vi "Main_Practice.vi"() -> ()   [LabVIEW 2015]
panel:
  in  "Snap Number Counting":dbl=12.0
  out "Movie Point cluster":cluster{"Movie Y":dbl[], "Movie X":dbl[]}={"Movie Y"=[-12.0, -12.0, -12.0, -12.0, -12.0, -12.0, -2.92, -2.92, -2.92, -2.92, -2.92, -2.92], "Movie X"=[-1.0, -1.0, -1.0, -1.0, -1.0, -1.0, 1.02, 1.02, 1.02, 1.02, 1.02, 1.02]}
  out "Movie Point  Y Array":dbl[](array[numeric])=[-12.0, -12.0, -12.0, -12.0, -12.0, -12.0, -2.92, -2.92, -2.92, -2.92, -2.92, -2.92]
  out "Movie Point  X Array":dbl[](array[numeric])=[-1.0, -1.0, -1.0, -1.0, -1.0, -1.0, 1.02, 1.02, 1.02, 1.02, 1.02, 1.02]
  out "Snap Point cluster":cluster{"Snap Y":dbl[], "Snap X":dbl[]}
  out "Snap Point  Y Array":dbl[](array[numeric])
  out "Snap Point  X Array":dbl[](array[numeric])
  out "Stage XY Cluster":cluster{"Stage Y ":dbl[], "Stage X":dbl[]}
  in  "Previous Light control":T1={"Filter Set"=0, "Lasers DO"=[FALSE, FALSE, FALSE, FALSE, FALSE, FALSE], "Lasers AO (V)"=[0.0, 0.0, 0.0, 0.0, 0.0, 0.0], "LED"=FALSE, "Global"=FALSE} {"Lasers AO (V)" min=0.0 max=5.0 step=0.01 scale=0.0..5.0 scale format="%#1.2f"; "Filter Set" items=["R-QuasAr", "R-Cy5", "R-mCherry", "R-mOrange", "R-GFP", "R-CFP/DAPI", "R-BFP", "R-LED", "SDC-Cy5", "SDC-mCherry", "SDC-mO2", "SDC-GFP", "SDC-CFP/DAPI", "SDC-BFP", "SDC-LED"]}
  out "Image Info":T2={"Status"="Ready", "scale bar (μm)"=65.0, "Image"=array512x512[262144 elements], "Histogram"={"max value"=1766, "mean"=1643, "min value"=1545, "Histogram"={"X Values"=[1546.105, 1548.315, 1550.525, 1552.7350000000001, 1554.9450000000002, 1557.1550000000002, 1559.3650000000002, 1561.5750000000003, 1563.7850000000003, 1565.9950000000003, 1568.2050000000004, 1570.4150000000004, 1572.6250000000005, 1574.8350000000005, 1577.0450000000005, 1579.2550000000006, 1581.4650000000006, 1583.6750000000006, 1585.8850000000007, 1588.0950000000007, 1590.3050000000007, 1592.5150000000008, 1594.7250000000008, 1596.9350000000009, 1599.145000000001, 1601.355000000001, 1603.565000000001, 1605.775000000001, 1607.985000000001, 1610.195000000001, 1612.405000000001, 1614.6150000000011, 1616.8250000000012, 1619.0350000000012, 1621.2450000000013, 1623.4550000000013, 1625.6650000000013, 1627.8750000000014, 1630.0850000000014, 1632.2950000000014, 1634.5050000000015, 1636.7150000000015, 1638.9250000000015, 1641.1350000000016, 1643.3450000000016, 1645.5550000000017, 1647.7650000000017, 1649.9750000000017, 1652.1850000000018, 1654.3950000000018, 1656.6050000000018, 1658.8150000000019, 1661.025000000002, 1663.235000000002, 1665.445000000002, 1667.655000000002, 1669.865000000002, 1672.075000000002, 1674.2850000000021, 1676.4950000000022, 1678.7050000000022, 1680.9150000000022, 1683.1250000000023, 1685.3350000000023, 1687.5450000000023, 1689.7550000000024, 1691.9650000000024, 1694.1750000000025, 1696.3850000000025, 1698.5950000000025, 1700.8050000000026, 1703.0150000000026, 1705.2250000000026, 1707.4350000000027, 1709.6450000000027, 1711.8550000000027, 1714.0650000000028, 1716.2750000000028, 1718.4850000000029, 1720.695000000003, 1722.905000000003, 1725.115000000003, 1727.325000000003, 1729.535000000003, 1731.745000000003, 1733.955000000003, 1736.1650000000031, 1738.3750000000032, 1740.5850000000032, 1742.7950000000033, 1745.0050000000033, 1747.2150000000033, 1749.4250000000034, 1751.6350000000034, 1753.8450000000034, 1756.0550000000035, 1758.2650000000035, 1760.4750000000035, 1762.6850000000036, 1764.8950000000036], "Histogram: h(x)"=[1, 1, 0, 1, 1, 4, 2, 5, 3, 18, 22, 16, 26, 37, 83, 73, 96, 128, 153, 340, 297, 408, 511, 1003, 839, 1047, 1268, 1532, 2908, 2476, 2946, 3424, 3916, 7140, 5665, 6592, 6956, 7907, 13141, 9628, 10167, 10808, 16785, 11493, 11379, 11298, 11102, 15845, 9865, 9151, 8683, 7999, 10287, 6013, 5256, 4358, 3885, 4618, 2525, 2027, 1707, 1987, 906, 827, 574, 438, 582, 244, 189, 143, 113, 100, 44, 30, 24, 22, 15, 12, 12, 2, 0, 3, 2, 4, 2, 1, 1, 0, 0, 1, 0, 0, 0, 0, 0, 0, 0, 0, 0, 1]}}, "Scale Info"={"Pixel size (nm)"=650.0, "Total x width (μm)"=332.8, "Total y width (μm)"=332.8}, "Camera View indicator"=array512x512[262144 elements], "max frame rate (Hz)"=100.0}
  out "log path":path=path "C:/Register info of scope/201707 regiser info.txt"
  out "ROI cursor":T3={"Bin"=1, "ROI"={"x offset"=0, "y offset"=376, "x width"=512, "y width"=1296}} caption="ROI" {"ROI"."x offset" min=1 max=512 step=1; "ROI"."y offset" min=1 max=512 step=1; "ROI"."x width" min=1 max=512 step=1; "ROI"."y width" min=1 max=512 step=1; "Bin" items=["1x1"=1, "2x2"=2, "4x4"=4]}
  out "Previous ROI":T3={"Bin"=1, "ROI"={"x offset"=250, "y offset"=500, "x width"=1500, "y width"=1000}} caption="ROI" {"ROI"."x offset" min=1 max=512 step=1; "ROI"."y offset" min=1 max=512 step=1; "ROI"."x width" min=1 max=512 step=1; "ROI"."y width" min=1 max=512 step=1; "Bin" items=["1x1"=1, "2x2"=2, "4x4"=4]}
  in  "Tab":T4(tab)
  in  "Load Excel to table":bool
  in  "Write table to excel":bool
  in  "Goto destination":bool
  in  "Clear Table":bool
  in  "Track on?":bool
  in  "Stage on?":bool
  out "SDC initialized":bool
  in  "Confocal on?":bool
  in  "Camera on?":bool
  out "Stage initialized":bool
  out "Camera initialized":bool[](array[boolean])
  in  "Light control":T1={"Filter Set"=7, "Lasers DO"=[FALSE, FALSE, FALSE, FALSE, FALSE, FALSE], "Lasers AO (V)"=[0.3, 0.3, 0.3, 0.3, 0.3, 0.3], "LED"=TRUE, "Global"=FALSE} {"Lasers AO (V)" min=0.2 max=5.0 step=0.01 scale=0.0..5.0 scale format="%#1.2f"; "Filter Set" items=["R-QuasAr", "R-Cy5", "R-mCherry", "R-mOrange", "R-GFP", "R-CFP/DAPI", "R-BFP", "R-LED", "SDC-Cy5", "SDC-mCherry", "SDC-mO2", "SDC-GFP", "SDC-CFP/DAPI", "SDC-BFP", "SDC-LED", "SDC-Cy3", "SDC-Di4"]}
  in  "Confocal scanner":T5={"SDC shutter"=FALSE, "Filter wheel"=0, "FW speed"=3, "Disk spinning"=FALSE, "Disk speed (rpm)"=3000.0} {"Disk speed (rpm)" min=1500.0 max=10000.0; "FW speed" min=1 max=5 step=1; "Filter wheel" items=["CFP"=1, "GFP"=2, "mCherry"=3, "Alexa-647"=4, "OFP"=5, "empty"=6]}
  in  "Stage-Ctrl":T6={"Console"={"L"=FALSE, "R"=FALSE, "FWD"=FALSE, "BACK"=FALSE}, "Step Width [mm]"=0.2, "Destination [mm]"=[0.0, 0.0], "Move "=FALSE} {"Destination [mm]" format="%_6g"; "Step Width [mm]" min=0.0 format="%_6f"}
  out "Stage Status":T7={" Current Position"=[-1.0, -12.0, 0.0], "Number of Axis"=3, "ILSID"=1}
  in  "Camera Ctrl":T8={"Chosen Camera"=1, "ROI selection"=0, "Live"=FALSE, "ROI define"=FALSE, "Snap"=FALSE, "ROI update"=FALSE, "ROI previous "=FALSE, "ROI"={"Bin"=4, "ROI"={"x offset"=0, "y offset"=0, "x width"=512, "y width"=512}}, "Exposure (ms)"=100.0, "Symmetrical"=TRUE, "Autoscale"=TRUE, "Scale"={"Scale.Min"=2730, "Scale.Max"=5572}} {"Scale"."Scale.Max" min=1 max=5000 step=1; "Scale"."Scale.Min" min=1 max=5000 step=1; "Exposure (ms)" min=1.0 max=5000.0 step=1.0; "ROI"."ROI"."x offset" min=1 max=512 step=1; "ROI"."ROI"."y offset" min=1 max=512 step=1; "ROI"."ROI"."x width" min=1 max=512 step=1; "ROI"."ROI"."y width" min=1 max=512 step=1; "ROI"."Bin" items=["1x1"=1, "2x2"=2, "4x4"=4]; "ROI selection" items=["Full ROI", "Central quad", "Confocal", "Patch 500", "Patch 1000"]; "Chosen Camera" items=["Left", "Right"]}
  in  "TI-Ctrl":T9={"Obj"=2, "Cube Bottom"=2, "Cube Top"=2, "PFS-Ctrl"={"PFS IO"=FALSE, "PSF Err"=FALSE, "PSF Pos"=0}, "Z-Ctrl"={"Z-pos"=499.625, "Home"=TRUE, "Sensitivity"=1}, "Condenser"=2, "Lightpath"=enum."R100"} {"Condenser" items=["A"=1, "DICN2"=2, "- empty 3 -"=3, "- empty 4 -"=4, "- empty 5 -"=5, "- empty 6 -"=6]; "Z-Ctrl"."Sensitivity" min=1 max=3 step=1 scale=1.0..3.0; "PFS-Ctrl"."PSF Pos" scale=0.0..16400.0; "Cube Top" items=["Quad-O"=1, "Quad-R"=2, "empty"=3, "empty"=4, "empty"=5, "DIC"=6]; "Cube Bottom" items=["Cy5"=1, "RFP"=2, "mO2"=3, "empty"=4, "CFP"=5, "GFP"=6]; "Obj" items=["20x/.75 Dry PFS"=1, "40x/1.3 Oil PFS"=2, "60x/1.4 Oil PFS"=3, "- empty 4 -"=4, "- empty 5 -"=5, "- empty 6 -"=6]}
  in  "Scope on?":bool
  out "Ti-E initialized":bool
  in  "stop program":bool
  in  "Record Table":string[][](table)
  out "Stage Trajec":cluster{"Value":dbl[], "Value":dbl[]}[](graph)=[{"Value"=[], "Value"=[]}, {"Value"=[], "Value"=[]}, {"Value"=[-12.0, -12.0, -12.0, -12.0, -12.0, -12.0, -2.92, -2.92, -2.92, -2.92, -2.92, -2.92], "Value"=[-1.0, -1.0, -1.0, -1.0, -1.0, -1.0, 1.02, 1.02, 1.02, 1.02, 1.02, 1.02]}]
  in  "Number":dbl
  out "Color Acquiring":bool
  out "T Acquired Progress":i32(slide)=100 scale=0.0..100.0
  in  "Load from Exel (For XY Scan)":bool
  in  "Load from table (For XY Scan)":bool
  in  "Generate Tiling":bool
  in  "XY Scan List":string[][](table)
  in  "Cal step num":bool
  in  "Cal step size":bool
  in  "Define 1":bool
  in  "Define 2":bool
  in  "Z-Stack":T10={"Z end"=1000.0, "Step Num"=10, "Step Size"=-200.0, "Z0"=3000.0, "z-stack?"=FALSE}
  in  "MD acquisition":bool
  in  "Channel settings":T11={"Take?"=[FALSE, TRUE, FALSE, FALSE], "Channel"=[1, 2, 3, 4], "Exposure time (msec)"=[100.0, 100.0, 100.0, 100.0], "Cumulation"=[1, 1, 1, 1], "Name"=["Cy5", "mCh", "GFO", "CFP"]} {"Exposure time (msec)" format="%0.0f"; "Channel" items=["R-QuasAr", "R-Cy5", "R-mCherry", "R-mOrange", "R-GFP", "R-CFP/DAPI", "R-BFP", "R-LED", "SDC-Cy5", "SDC-mCherry", "SDC-mO2", "SDC-GFP", "SDC-CFP/DAPI", "SDC-BFP", "SDC-LED", "SDC-Cy3"]}
  in  "Period (s)":u32=3
  in  "Timelapse Cycles":i32=100 caption="# Cycles"
  in  "Timelapse?":bool=TRUE
  out "Timelapse Acquired":i32=100 caption="Acquired"
  out "Timelapse Time (s)":dbl=297.037 caption="Time (s)"
  in  "Movie frame rate (Hz)":dbl=10.0 format="%0.0f"
  out "Frames Recorded":i32=1000
  in  "Stream movie":bool
  in  "# frames":i32=1000
  in  "Total time (sec)":dbl=100.0 min=1.0 max=5000.0 step=1.0
  out "Elapsed time (sec)":dbl=100.541 min=1.0 max=5000.0 step=1.0
  in  "Base folder":path=path "C:/Users/ZouOptics/Desktop/test"
  in  "Sub-folder":string="Image"
  out "Full path":path=path "C:/Users/ZouOptics/Desktop/test321/153424_step"
  in  "XY tiling":T12={"Tiling?"=FALSE, "YY/XX"=[1, 1], "X0Y0"=[-1.0, -12.0, 0.0]}
  in  "Excel Loading Path":path=path "X:/Data and analysis/Sicong Wang/Fluorescence Images/test.xlsx"
  out "Z Stack Aquired":i32(slide)=10 scale=0.0..1.0
  out "Stage Trajec for tiling":cluster{"Value":dbl[], "Value":dbl[]}[](graph)
  in  "Ranking":u16(ring) items=["Identical", "Minimum Distance", "Snake"]
  in  "Waveform channels":T13={"Lasers"=[FALSE, FALSE, FALSE, FALSE, FALSE, TRUE], "Patch"=TRUE, "Camera Output"=TRUE}
  out "Lasers DO waveform":digitalwaveform[](graph)=[{"t0"=timestamp(0 s since 1904-01-01), "dt"=4.7260140608370336e-05, "Y"={"transitions"=[0, 255999], "data"=[[0], [0]]}}]
  out "Lasers AO waveform":waveform(dbl)[](graph)=[{"t0"=timestamp(0 s since 1904-01-01), "dt"=4.7260140608370336e-05, "Y"=array[256000 elements]}]
  in  "Load waveform":bool
  in  "Waveform info":T14={"Waveform folder"=path "C:/Users/ZouOptics/Desktop/MATLAB codes/ephys waveforms_new/Voltage step -70 to +30_(Baseline -30)_Sync/1058Hz", "Exposure time (ms)"=0.9452} {"Exposure time (ms)" format="%0.5f"}
  out "AI Waveform":cluster{"xo":i32, dbl, "data":dbl[][]}(graph)={"xo"=0, 4.7260140608370336e-05, "data"=array2x256000[512000 elements]}
  in  "Run waveform":bool
  out "Patch Ex. Command AO waveform":waveform(dbl)(graph)={"t0"=timestamp(0 s since 1904-01-01), "dt"=4.7260140608370336e-05, "Y"=array[256000 elements]}
  out "Seal test DAQ params":T15={"samples"=40000, "Duration (sec)"=2.0, "Downsampling factor"=2000.0}
  out "Patch seal test waveform":waveform(dbl)(graph)={"t0"=timestamp(0 s since 1904-01-01), "dt"=5e-05, "Y"=array[40000 elements]}
  in  "Save patch param":bool
  in  "Pipet tuning parameters":T16={"Amplitude (mV)"=5.0, "Number of repeats"=20, "DAQ rate (Hz)"=18000.0, "Frequency (Hz)"=9.0}
  in  "Test patch":bool
  out "Patch output":cluster{"xo":i32, dbl, "data":dbl[][]}(graph)={"xo"=0, 5e-05, "data"=array2x40000[80000 elements]}
  out "Average I-t curve":cluster{"xo":i32, dbl, dbl[]}(graph)={"xo"=0, 5e-05, [2.0417260685456067, 1253.8993045801826, 886.9786190905347, 94.0376108026094, 3.737020498750642, 2.5067554541169064, 2.855059414906045, 1.8381668770481967, 2.1624219933656548, 1.9509218040771357, 1.934813958158526, 2.2168142088177545, 1.9751965042279445, 2.2611672520831196, 2.8471184161871936, 2.1381472934482746, 1.820186708359053, 1.8463337280397083, 2.2310497350559673, 2.359686654433676, 2.6274513784474043, 1.8685102501320947, 1.719343272932873, 2.1502846440331758, 1.6187256933524625, 1.90072594427519, 1.820186708977287, 1.9952748485030591, 2.1684906670373976, 2.0821086148710837, 2.051765240438174, 1.9411084888144587, 1.8764512456996978, 1.874578923916529, 2.2046768589871264, 2.1624219918808265, 1.777931841388993, 2.214941887916387, 1.5865099995033718, 2.1561274612778965, 1.953019982143028, 2.114098451653413, 1.8120198568928094, 1.7615981390665891, 1.9873338533952503, 1.5101671186868888, 2.104059280816585, 1.8323240586872382, 2.073715905629104, 1.7900691917396214, 2.0618044140191816, 1.6973926068748197, 1.9369121343479463, 1.7174709524842522, 1.939010311682769, 1.7135004544061427, 1.808049358815561, 1.9187061113508848, 2.061804414954046, 1.7819023411100938, 1.8320982021780146, 2.080010438463449, 2.321176429831114, 1.8804217432799095, 1.7898433359161992, 2.2492557591611586, 1.8524024023892816, 1.7114022777723337, 1.5745985068678088, 2.3396083096232805, 1.564559333332313, 2.0235200440709096, 1.9992453448323426, 1.6187256932242051, 1.834196378125948, 1.946951307212812, 1.8885885943614502, 2.2511280790218255, 2.0396278915798467, 1.699490784714807, 1.7898433353808931, 2.2611672530931894, 1.7618239955382338, 1.6047160227187378, 1.578569003498251, 2.0898237532207324, 2.2933829443265292, 2.0597062362316056, 2.188794867746452, 1.8262553835988153, 1.8685102503505795, 2.1201671266063107, 1.9772946809825582, 1.725637803912771, 2.2368925526404, 2.226853380581651, 1.7779318435295863, 1.848431904597925, 1.8038530048083343, 1.9831374992754824, 1.8906867722017346, 2.242961227578504, 2.3295691366227467, 1.866412072533204, 2.087951432500877, 1.8442355506519916, 2.3276968156918723, 1.9289711402578082, 1.9107651168613171, 1.6026178463637668, 1.650941386990575, 1.7074317797698197, 1.4476080503819675, 2.0034416998411837, 1.6509413870358998, 2.301323940994293, 1.6992649283715244, 2.083980935372533, 2.025618221993952, 1.9871079960415765, 2.130206299742764, 1.98313749960743, 2.2249810606757805, 2.0375297146743794, 2.3496474822170694, 2.073941762296804, 2.1243634807635647, 1.836294555506038, 1.5664316540898264, 1.930843460246671, 1.9168337909245647, 1.6107846986292407, 1.7335787989451874, 1.4697845726476597, 2.3375101320698337, 2.0517652410334306, 1.7860986942118973, 1.9691278286266753, 1.7919415130173741, 1.8019806849853486, 1.7174709514363364, 2.1019611029006007, 1.9609609777484944, 2.108029777258671, 1.7819023399187264, 1.9107651151653482, 1.8220590280317805, 2.011382695446457, 1.5986473490021436, 2.265137749580131, 1.842363231100096, 1.4879905973859955, 1.5120394387436262, 1.7800300195077283, 1.7819023391951578, 1.7275101247383826, 1.9772946813973518, 1.8001083639634634, 1.9208042890704071, 2.2025786827075478, 1.9329416381848765, 2.408010195015801, 1.6448727121581632, 1.6791865836289506, 2.0375297144183495, 1.369166992411865, 1.5986473484971557, 1.4375688791075958, 1.5846376787829186, 1.7758336646792983, 1.165833657363045, 1.5302454630146518, 1.9590886567945887, 1.7536571442906714, 2.0013435235088277, 2.238990729530317, 1.655137741170631, 1.9429808095646772, 1.6973926079604522, 2.174559343686368, 1.961186834514391, 1.7858728386224914, 1.9086669384784112, 1.6691474113143505, 1.7394216168008125, 1.8806475999774614, 1.6268925449166818, 1.610784697701938, 2.124137624156634, 2.261167251630461, 1.5685298315907779, 1.7214414495520016, 1.8463337274816893, 1.302637428259863, 1.791941511532541, 1.846333727579565, 1.9730983264031752, 1.969127829425819, 1.7576276417275907, 1.991078494677416, 1.9630591549931873, 1.5603629801471233, 1.8341963779526336, 2.365755329394038, 1.5381864584692415, 1.5181081136589667, 2.365981184961349, 2.3860595294170515, 2.0657749121649114, 2.2308238787652064, 1.898627766299558, 2.154480997036838, 2.3659811852779677, 1.9973730254462516, 1.8825199198835336, 1.969127828920743, 1.8402650527700013, 1.9710001491584872, 1.8484319062491823, 2.2751769222263425, 2.1885690137774216, 2.210745534633673, 1.9892061737384172, 2.3113631129776775, 2.218912385707873, 1.8302258808848253, 2.037755571206306, 1.9651573322226212, 2.3034221162794326, 2.363883009171796, 2.774520177572746, 2.7343634893465834, 2.448392740557692, 2.168490667059863, 1.9408826329759599, 1.96725550825349, 2.178529840196197, 1.8341963784501956, 2.136274973994527, 1.8825199199289142, 1.5664316549795019, 2.073715907310632, 2.1180689501080687, 1.9569904799798323, 2.047568887547033, 2.5511084966285056, 2.017677226969594, 1.81224571403525, 2.11012795493249, 1.8967554466046705, 1.846333727715335, 2.2450594046719448, 2.065774910958578, 1.7798041628477348, 2.408236051403954, 1.9691278298484172, 2.466598764172413, 1.9369121352221241, 2.5188928036985687, 1.7819023398360951, 1.5281472863354846, 2.0578339158734598, 1.5704021517532982, 2.196735862801343, 2.0697454084259803, 2.2186865290702857, 2.053637560366814, 2.0253923651455765, 2.1624219928001716, 1.894431412571606, 2.5571771705714292, 2.0818827578493018, 2.0839809349204486, 1.8724807475689245, 2.0797845824899195, 1.749686645662408, 1.8262553834025186, 1.9189319664129132, 1.6147551962849764, 2.0940201076798166, 1.870608427474335, 1.7919415123238305, 1.8442355508250536, 2.003215844093438, 1.8785494218434278, 1.9147356148789598, 2.198834040694207, 1.9770688248126298, 2.0335592170639467, 1.7114022770863602, 2.055735739503272, 1.5262749656755685, 2.180402160539605, 1.9532458383132008, 2.083980934257628, 2.45843191267586, 1.554294304734296, 2.0678730880224783, 2.1201671253702488, 2.1563533186241064, 1.6450985692932814, 2.21471603171652, 1.8141180334816578, 1.6950685736262683, 1.9369121349281533, 1.6570100613482273, 1.9833633560259472, 1.769764990367449, 1.7940396893950517, 1.9229024642871313, 2.206775036615826, 2.412206549685168, 1.916833790336706, 1.8402650531921256, 2.0557357386966673, 2.301323941575197, 1.6208238698884838, 1.650941386719193, 2.156579174876892, 2.021421868025013, 2.0655490548943023, 2.1946376876522877, 2.1040592798361732, 1.6168533722554814, 1.963059154714062, 1.7396474737095133, 1.3892453377342557, 1.7317064786621372, 1.7214414495968833, 1.9046964418630892, 2.100088782806101, 1.8967554459785505, 1.8524024018016176, 1.9450789871106495, 1.9229024648752293, 1.876451245247103, 1.7919415118941568, 1.8080493590714146, 1.8685102498604655, 1.6448727123768145, 2.0113826953788307, 2.1666183468220446, 1.5500979507351607, 1.6530395637526554, 1.6992649284091805, 1.9067946188889788, 1.7359028328044417, 2.355716156801489, 1.6289907218597313, 1.7436179718854632, 2.3255986392535473, 1.886716273422966, 1.4837942429649134, 1.9210301439589335, 1.62479436811703, 2.0940201079136984, 1.701363104847044, 2.1624219936219564, 1.904696441139299, 1.6630787368364583, 1.5904804965029962, 2.019323690893603, 1.3810784859965395, 1.8241572054572108, 1.7517848232237825, 2.126235801815576, 1.6672750906319491, 1.658882382007932, 1.7034612820839665, 1.8162162109902826, 1.920804288572947, 1.383402520481611, 1.733352941674445, 1.6350593975817627, 1.8019806846911155, 1.8927849489185578, 1.9812651783670654, 1.6509413872696557, 1.7053336024875314, 1.3710393132749839, 1.7940396901564575, 1.9913043503875825, 1.6810589033090495, 1.4476080507361315, 1.3409217971827674, 2.452363237986799, 1.8444614063696958, 1.745716148685112, 2.1182948050494703, 1.6026178456251612, 2.041726068779284, 1.4938334142013308, 1.7576276408757612, 1.8302258813597438, 1.52814728633553, 1.4214610319755243, 1.878549423109973, 1.7618239950556533, 1.8745789255600032, 1.9651573323658094, 2.1423436488193692, 2.017451371055501, 1.928971140001302, 1.9630591539753304, 1.7779318424741113, 1.8019806843820845, 2.29128476931349, 2.108029776775793, 2.2168142086895632, 2.2249810601480116, 2.4887752870341155, 2.132304475652921, 2.1061574572237833, 2.2329220556553806, 1.8785494224843942, 1.9348139584750979, 2.227079238327499, 2.1283339782084414, 1.6551377418114765, 1.9952748491212586, 2.079784582172961, 2.4483927403386407, 2.1785298407089932, 2.3477751616410893, 2.291284770067482, 2.4283143968777567, 2.023520044598679, 1.8806475996686687, 1.7798041623124692, 2.220784706978223, 1.908892794588293, 2.011382694760579, 2.2147160312866627, 2.1180689502740497, 1.7657944929827276, 2.3235004622125333, 1.7457161492882058, 2.2289515586405377, 1.7517848232386506, 1.8986277666611477, 1.7879710155428539, 1.7879710154295854, 2.218912386446616, 1.9387844564703096, 2.242961227789147, 1.8827457768074318, 1.9511476610468554, 2.086079112888892, 1.8703825705431725, 2.2812455957394695, 1.6107846981542202, 2.1988340414854135, 1.9913043504330088, 2.03355921701147, 1.9651573317476483, 1.8524024026533008, 2.438353567232566, 1.9509218038736127, 1.632961218980307, 1.9852356755026288, 2.049667064173556, 2.206775037784609, 1.9871079979416972, 1.9268729632921413, 1.8944314126771873, 2.3699516830767524, 1.4798237450527842, 1.7053336029549873, 2.3678535064352397, 1.7980101868397715, 1.8563728999845757, 2.4000692013024674, 2.277275098445713, 2.1663924901472225, 2.2651377490071303, 1.8825199191826052, 1.854274722740175, 2.1845985137470225, 2.1624219933434756, 2.2530003997646686, 2.112000275931785, 1.707431779468222, 1.701363105661214, 2.0013435232297954, 1.8846180975655467, 2.204676858218378, 1.6289907219202926, 2.1502846428042903, 2.1201671267041435, 2.0396278910672074, 1.7980101863421625, 1.6612064160634072, 1.9733241835983628, 1.9691278283705214, 1.963059153636181, 1.9046964411016603, 2.0235200452016717, 2.1323044764669574, 2.182500337648151, 1.8040788622149084, 1.8503042248289991, 1.7697649911059035, 1.805951182791855, 1.7758336655993383, 1.9088927954323456, 1.4195887120167645, 1.8584710766789028, 2.023520045239711, 2.4042655536885458, 1.6128828744942023, 2.090049610355841, 1.6065883433184167, 2.0074121986127915, 1.7980101870129108, 2.0718435857913406, 1.7377751532079873, 2.019549546739697, 2.1423436490304035, 1.8965295890471285, 1.99924534705629, 1.4415393762732072, 2.283117917047806, 1.7475884692320447, 1.7858728371901473, 1.9046964415991179, 1.781902340190157, 1.810147536888862, 2.0739417631712658, 2.1684906673838857, 1.977294680914829, 1.5886081763107165, 1.9025982639480632, 1.9955007057585885, 1.3409217970243839, 1.971226005954126, 1.6490690674842847, 1.9973730261396336, 1.5444809893511395, 1.701363105058187, 2.0235200450283837, 1.5603629802450054, 2.2852160932823677, 1.5624611576705827, 1.771863167973424, 1.491961093813074, 2.2168142094204515, 2.00531402025977, 1.8946572682140463, 2.0256182217754595, 1.5846376785116276, 1.49802976991177, 2.377892679677175, 1.3651964956905198, 1.7819023397377836, 1.886490417252868, 1.7375492973018554, 1.6992649271048936, 1.5886081764537678, 1.7657944935180827, 1.8563729006631113, 1.699264928371419, 1.67918658408144, 1.5946768507056814, 2.1423436484047174, 1.7840005173140974, 1.7676668136652258, 1.72773598120236, 1.604716023095719, 1.872480746913144, 1.9873338536287857, 2.0898237537486155, 1.4396670565254317, 1.564333477078996, 1.846333727805688, 2.017451369660728, 1.8080493589355398, 1.9551181600662755, 1.808049359109039, 1.9992453442071179, 1.862441574862212, 1.7798041628474537, 1.6731179084498968, 1.7354511194166367, 2.0958924281287343, 2.045696567211292, 1.4658140752029742, 1.7800300193493699, 1.586735856389554, 1.562461156818712, 1.5886081765592495, 1.649069066685036, 1.5503238077193355, 1.9952748481034626, 1.3472163287882577, 1.5664316544592356, 1.4256573866455704, 1.4618435778338141, 2.0456965661409017, 1.8241572074096462, 2.259069075479168, 1.8442355508777972, 1.5825395013424584, 2.1806280173880213, 2.397971021653007, 1.8080493600589471, 1.7536571440568602, 2.0176772259364153, 2.051765240882705, 2.2289515589421964, 2.0335592163180163, 2.359686654049342, 1.8059511815780986, 2.122265304220414, 2.313461289701952, 1.8362945553102352, 1.890686771817199, 1.965157329976442, 2.200706361994751, 2.5450398228886644, 2.494618105711745, 2.1904413330199235, 2.6757749198812735, 2.468471086355231, 2.418275224208858, 2.091921930020546, 2.1302062988454225, 1.7095299565622932, 2.112226131747266, 2.454461415419455, 2.2611672517059094, 1.9308434599905215, 2.619510383098207, 2.508853631165441, 2.148412323071361, 1.6026178459114735, 2.3498733382136674, 1.9651573312350017, 1.9873338529956706, 2.0697454090668015, 1.6208238705367437, 1.6971667506368033, 2.0314610395482378, 2.081882758294369, 1.69716675031265, 2.0898237522183702, 1.9913043505610195, 2.039627892280825, 1.953019983236565, 2.204676858353588, 2.045696566155969, 2.1241376243299483, 2.381863176420567, 1.9590886574805249, 2.065774910853025, 2.1785298392461905, 1.878549421971616, 2.0919219290709794, 1.8423632305647184, 1.7837746604730462, 2.025392365808859, 1.9509218056825584, 2.2329220559043526, 1.8624415748398215, 2.055735739578704, 1.9651573315893587, 1.7478143261558152, 2.025618220795598, 2.1465400027810166, 1.9852356762638328, 1.9390103115926507, 1.9469513073710882, 2.0496670640602064, 2.3778926790741464, 2.424118042509189, 2.0092845183075756, 2.2812455968629446, 1.739647473294951, 2.406137874076526, 2.31158897020288, 1.580441324120492, 2.1764316620847914, 1.799882507386555, 2.1442159703315484, 2.3979710221734156, 2.367853505967976, 2.1906671885266733, 2.101961102192137, 1.993176671243468, 1.840265052852742, 2.267010069335583, 1.5643334773127218, 2.259069074845976, 2.4586577696071203, 1.878549422763292, 2.122265303549268, 1.6147551956214825, 1.7235396269471088, 1.8524024030452582, 2.130206299064254, 2.3314414590240005, 1.7716373119846025, 2.2368925522561764, 2.164520170361931, 1.8806475991936273, 2.3517456592733406, 2.0174513700601957, 1.8101475366626159, 1.9973730254015747, 2.134402653560974, 2.0657749107927996, 1.5160099363767034, 2.0858532546083617, 1.7053336025028405, 1.729608301922552, 2.248804045132951, 2.353617980302397, 1.9691278289359335, 1.576470826774048, 1.900725944494141, 2.1785298397364916, 1.803853004876159, 1.9691278281896698, 1.924774786319161, 2.021421867512374, 1.7858728373632624, 1.9429808098588175, 1.961186834069544, 1.959088657066307, 1.8745789240068607, 1.7375492972417583, 2.158451496562146, 2.2651377493767613, 1.8101475365420427, 1.7174709528459722, 1.6670492340472745, 2.0356573943612837, 2.003441700866309, 1.9429808093686736, 1.8362945561922113, 1.995274848759331, 2.162421992807744, 1.5360882811947394, 2.357588477332434, 1.725411947162465, 1.5442551335883163, 1.9651573312726034, 2.0779122605179836, 1.8281277037157608, 1.387373017677481, 1.6068142007096986, 1.74174565114249, 1.8341963787291373, 1.5463533100711915, 1.7454902917237356, 1.8061770395725318, 1.9490494839598624, 1.5563924819863342, 2.2228828829187854, 1.5965491712222444, 2.0153531932455446, 1.705333603520487, 1.594450994226552, 1.9005000872837428, 1.8239313494074774, 1.92290246530461, 2.047794743091245, 1.933167494580854, 1.6752160861316114, 1.4135200365887752, 2.1423436485705554, 1.9551181589955593, 1.528147285129337, 2.335637812450552, 1.260382561900118, 1.6892257561172657, 1.9046964397373736, 1.5302454630447389, 1.7898433351470369, 1.8664120721185586, 1.3710393138251529, 1.7013631053219356, 1.385274840508333, 1.950921805599686, 1.8080493595688558, 1.846333728069487, 1.8745789237582116, 1.5685298316208696, 1.3792061662563857, 1.5967750285834772, 1.806177039323624, 2.273304600767557, 1.5946768509769889, 2.0435983893713594, 1.8605692546547727, 1.8846180966985673, 1.935039814886539, 1.6430003925839731, 1.65303956305978, 1.6187256929000884, 2.0214218684397056, 1.4718827504802703, 1.693196253644707, 2.1603238164381002, 2.067873087803662, 1.852402402962366, 2.162421992483728, 1.8885885943013212, 2.295481122136617, 1.830225880605879, 1.7093041004900509, 2.265137749188581, 1.8503042258685907, 2.0134808722009763, 1.9168337911509812, 2.315559467511979, 1.939010312821067, 1.8381668754652298, 1.7135004542781156, 1.9651573323582845, 2.3860595301333176, 2.4402258888723853, 2.49461810426367, 2.005314020915589, 2.2207847056594536, 2.410108371400865, 2.1484123228528658, 2.025618220795421, 2.1906671898843872, 2.236892553273628, 2.186696692175095, 2.011382695831485, 2.081882757449709, 2.146314145653459, 2.4243438994483095, 1.9408826330969298, 1.775833666360646, 1.715598632253843, 2.1785298397437356, 2.047794743159447, 1.8864904172451549, 2.1140984526107105, 1.934813958248939, 2.043598389190301, 1.3710393134105237, 1.9791670010324602, 2.325598638575598, 1.8001083642952824, 2.041726069517973, 1.7798041628100871, 1.8806475993067047, 1.8563728998867977, 2.1140984516759396, 2.0538634182628557, 1.961186834770241, 2.2107455335854826, 1.834196378367258, 1.8524024030903585, 2.116196629184252, 2.184598514885569, 2.478736114146293, 1.995274848246722, 1.7676668133335827, 1.9670296527695688, 1.9630591552418681, 2.077912260758919, 2.162421992272752, 1.83045173823091, 1.6068142010263737, 2.102186959070956, 1.8603433979116544, 2.0074121986954863, 1.693196253094183, 1.8825199193181597, 1.9268729612718754, 2.5772555167305544, 1.9854615321248892, 1.6086865204274308, 2.464500587598284, 1.9350398148941326, 1.7436179716291214, 2.2268533808608058, 1.5643334777725424, 2.1423436487139504, 1.9147356131975624, 1.8885885941659173, 1.8120198573301292, 1.8563729004899763, 1.8925590923489641, 1.7335787991410883, 2.180628017357733, 2.265137749421933, 1.8888144501775364, 1.7235396278366626, 2.071843586522187, 2.0174513703618246, 1.9128632931633556, 2.0034416994869524, 2.1320786189252074, 1.5421569553861434, 2.462402410852292, 2.4946181038188757, 1.9710001501237118, 1.7013631057744147, 2.269108247808897, 1.3992845101544231, 1.7737354879776164, 1.7919415115929296, 2.0940201070771485, 2.1523828207269036, 1.9411084890481254, 1.624794367521645, 1.944853130315382, 2.083980935538873, 1.7114022768526274, 1.6331870768313388, 2.1262358001874127, 1.842363230398724, 1.5844118220022894, 2.291284768981405, 1.5141376161541737, 2.1059316004209334, 1.9025982654403493, 1.9348139579851817, 1.5162357935870643, 1.5745985071468078, 2.247157580936482, 1.8703825698344547, 1.864539752317799, 1.6691474112088915, 2.0618044127147663, 2.146314145660671, 2.200706361158693, 2.5793536922414733, 1.377107988431434, 1.4858924201866643, 1.9287452831678833, 1.6630787360900006, 2.0839809345284572, 1.9952748482394085, 1.8542747227628096, 1.29656875336726, 1.83022588099789, 1.62479436795867, 1.9852356762110739, 1.8383927327959004, 1.892784947735756, 1.8624415744550988, 1.6752160865916694, 1.665176912987819, 1.7900691927422279, 1.886716273460648, 1.804078861634215, 2.188569012541085, 1.7536571447883835, 1.7636963155196688, 1.876677101582973, 1.6488432095199888, 1.9226766081094695, 1.7415197946107235, 1.8542747236297008, 2.2046768588663426, 2.4544614149372355, 1.8040788617474774, 1.7314806220171064, 1.852402402728548, 1.8524024021179462, 2.295481122128775, 1.8745789247985618, 1.9873338535156835, 1.7536571439059827, 1.812019856154121, 1.3530591466893196, 1.9147356136573879, 1.8383927331956578, 2.075814083152592, 1.6247943672801977, 1.4576472227868826, 1.9490494837712802, 1.657010061845593, 1.8080493587772708, 1.798010187457645, 2.03168689660025, 1.9973730265015823, 1.705333602668602, 1.854274723576904, 2.0718435858739515, 1.7275101241127848, 2.150284642457391, 1.7114022773877988, 1.876451244855222, 1.5181081136514354, 1.7858728381699671, 1.9793928576544404, 1.9892061741306855, 1.6691474114427807, 1.7256378035509747, 1.6591082391354803, 1.6633045929611012, 1.4616177206762926, 1.7114022775009439]}
  out "Patch quality":T17={"Ra (MΩ)"=7.986924854740489, "Rm (MΩ)"=2698.372739361534, "Cm (pF)"=11.553090440401073, "RC constant (msec)"=0.09227366518750409, "Steady state current (pA)"=1.8529686158862757}
  in  "Path of saving register":path=path "C:/Register info of scope"
  in  "Calibrate stage":bool
  in  "Hardware Settings":T18={"DAQ ports"={"Lasers DO lines"=["Dev2/port0/line0", "Dev2/port0/line1", "Dev2/port0/line2", "Dev2/port0/line3", "Dev2/port0/line4", "Dev2/port0/line5"], "Lasers AO lines"=["Dev2/ao0", "Dev2/ao1", "Dev2/ao2", "Dev2/ao3", "Dev2/ao4", "Dev2/ao5"], "Patch AO line"="Dev1/ao1", "Patch AI lines 1"={"Patch scaled output"="Dev1/ai13", "Patch 10 V_m "="Dev1/ai8"}, "Camera timing DI"="Dev1/port0/line8", "Dev1 timing DO "="Dev1/port0/line15", "Dev1 trigger source"="/Dev1/PFI0", "Dev2 trigger source"="/Dev2/PFI0", "LED line"="Dev1/port0/line0", "Global Shutter line"="Dev2/port0/line6", "Patch AI lines 2"={"Cell capacitance"="Dev1/ai9", "Mode"="Dev1/ai10", "Frequency"="Dev1/ai11", "Gain"="Dev1/ai12"}}, "Camera Setting"={"Camera Output triger mode setiting"={"Mode"=3, "Polarity"=2, "Period"=0.0005, "Delay"=0.0}, "Camera timing port for trigering"=enum."3"}, "Stage setting"={"Baudrate"=57600, "COM Port"="COM10", "Xmax"=118.5, "Xmin"=15.0, "Ymax"=76.5, "Ymin"=12.2}, "Confocal VISA Setting"="COM1"} {"Camera Setting"."Camera Output triger mode setiting"."Polarity" items=["Negative"=1, "Positive"=2]; "Camera Setting"."Camera Output triger mode setiting"."Mode" items=["Low"=1, "Global Exposure"=2, "Programmable"=3, "Trigger Ready"=4, "High"=5]}
  out "Camera":errorcluster
  out "Stage":errorcluster
  out "Confocal":errorcluster
  out "Camera Info":T19={"Camera Details Array"=[{"Model"="C11440-22C", "Camera ID"="S/N: 003222", "Firmware"="3.20.A"}, {"Model"="C11440-22C", "Camera ID"="S/N: 003223", "Firmware"="3.20.A"}], "Handle"=1, "Camera in use "={"Model"="C11440-22C", "Camera ID"="S/N: 003223", "Bits"=16}}
  out "Confocal Info":T20={"Actual Disk speed (rpm)"="3000", "Actual FW speed (rpm)"=3}
  in  "Ti Control Lib":refnum<k7>
  out "TiE Ref":T21 caption="Ref (can be hidden)"
  out "Previous Bin":u16(ring)=1 caption="Cursor Bin" items=["1x1"=1, "2x2"=2, "4x4"=4]
  # "Nikon Scope v2.12"
  # "Red"
  # "637"
  # "561"
  # "488"
  # "405"
  # "532"
  # "Camera"
  # "Left Camera"
  # "Right Camera"
  # "Stage"
  # "DON'T Close the window \nuntil this button turns RED!"
  # "Stage Status"
  # "Confocal Scanner"
  # "Nikon control"
  # "Red"
  # "637"
  # "561"
  # "488"
  # "405"
  # "532"
  # "X"
  # "Y"
  # "X"
  # "Y"
  # "File I/O"
  # "Multidimensional acquisition"
  # "Stream"
  # "1. Timelapse"
  # "2. Channel"
  # "grey out at start up"
  # "3. XY Scan"
  # "4. Z-stack"
  # "Need to add tiling function"
  # "X"
  # "Y"
  # "Load waveform"
  # "637"
  # "561"
  # "532"
  # "488"
  # "405"
  # "Red"
  # "Pipet tuning"
  # "Need to restart the program if these settings are changed."
  # "Trigger source: PFI0= right camera (default);\n                           PFI8= left camera"
  # "637"
  # "561"
  # "532"
  # "488"
  # "405"
  # "Red"
  # "Camera information"
  # "Confocal Status"
  # "Power calibration (2017-02-09) Confocal mode\nLaser\t     Voltage\t   mW\n405nm     1             1.22\n488nm\t    1\t            2.90    \n532nm\t    1\t            4.76    \n561nm\t    1\t            4.47       \n637nm\t   \t1             9.95"
  # "Low gain = 100mV/nA\nWith external set to div10,\nthis means DAQ 1mV = 1 pA"
  # "When updating filter set information, please edit:\nsubDAQ_SetFilterSet.vi"
  # "Global shutter mode : 4"
  # "Minimum AO for all lasers: 0.3 V"
  # "Frame        DAQ rate       Exposure\nrate (Hz)       (Hz)            time (ms)\n986.1          9681.46         1.03290\n1058          21159.48        0.9452"
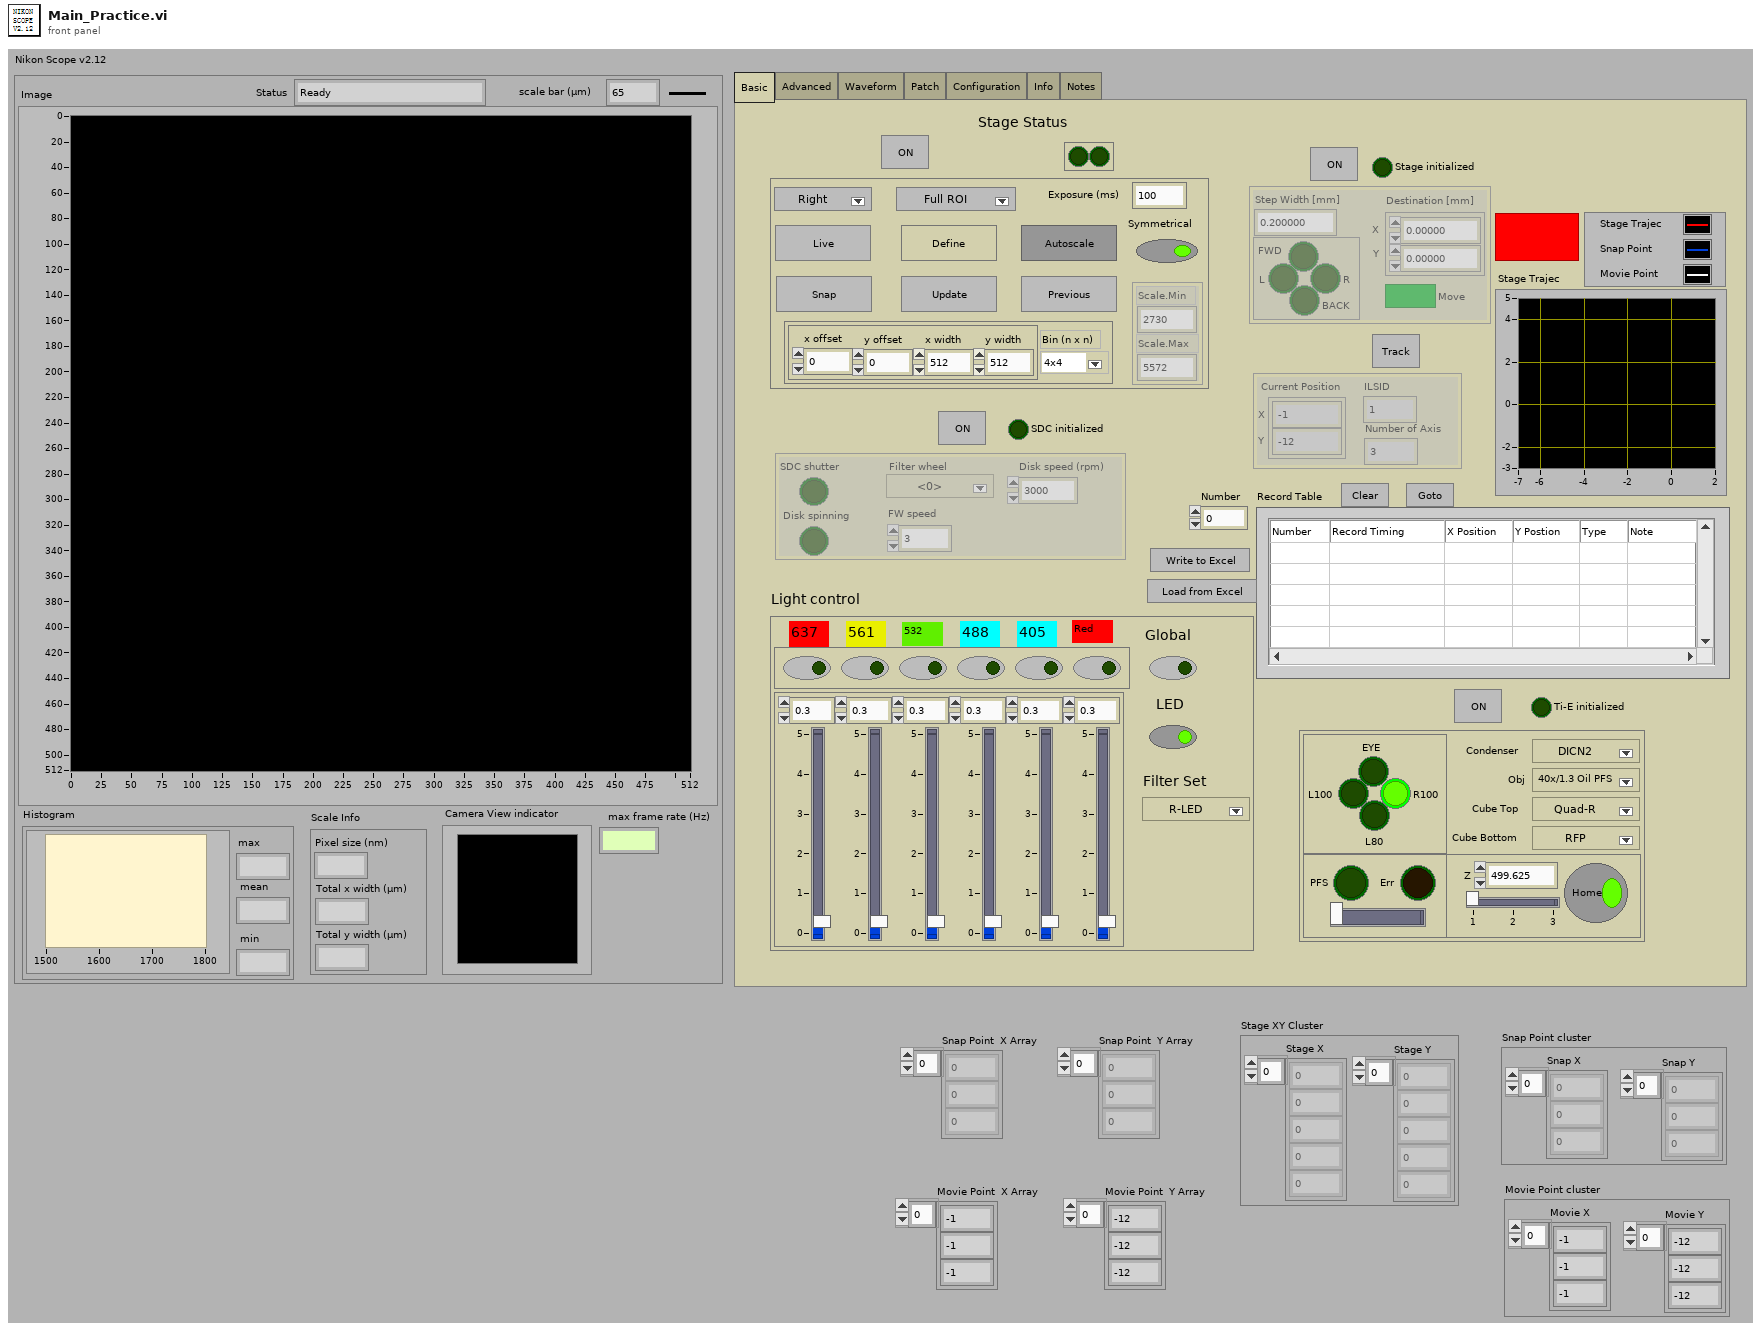
[diagram p1: front panel]
types:
  T1 = cluster{"Filter Set":i32, "Lasers DO":bool[], "Lasers AO (V)":dbl[], "LED":bool, "Global":bool}
  T2 = cluster{"Status":string, "scale bar (μm)":dbl, "Image":u16[][], "Histogram":cluster{"max value":u16, "mean":i16, "min value":u16, "Histogram":cluster{"X Values":dbl[], "Histogram: h(x)":i32[]}}, "Scale Info":cluster{"Pixel size (nm)":dbl, "Total x width (μm)":dbl, "Total y width (μm)":dbl}, "Camera View indicator":u16[][], "max frame rate (Hz)":dbl}
  T3 = cluster{"Bin":u16, "ROI":cluster{"x offset":i32, "y offset":i32, "x width":i32, "y width":i32}}
  T4 = enum32{"Basic", "Advanced", "Waveform", "Patch", "Configuration", "Info", "Notes"}
  T5 = cluster{"SDC shutter":bool, "Filter wheel":u16, "FW speed":i32, "Disk spinning":bool, "Disk speed (rpm)":dbl}
  T6 = cluster{"Console":cluster{"L":bool, "R":bool, "FWD":bool, "BACK":bool}, "Step Width [mm]":dbl, "Destination [mm]":dbl[], "Move ":bool}
  T7 = cluster{" Current Position":dbl[], "Number of Axis":i32, "ILSID":i32}
  T8 = cluster{"Chosen Camera":u32, "ROI selection":u16, "Live":bool, "ROI define":bool, "Snap":bool, "ROI update":bool, "ROI previous ":bool, "ROI":cluster{"Bin":u16, "ROI":cluster{"x offset":i32, "y offset":i32, "x width":i32, "y width":i32}}, "Exposure (ms)":dbl, "Symmetrical":bool, "Autoscale":bool, "Scale":cluster{"Scale.Min":i32, "Scale.Max":i32}}
  T9 = cluster{"Obj":u16, "Cube Bottom":u16, "Cube Top":u16, "PFS-Ctrl":cluster{"PFS IO":bool, "PSF Err":bool, "PSF Pos":u32}, "Z-Ctrl":cluster{"Z-pos":dbl, "Home":bool, "Sensitivity":u8}, "Condenser":u16, "Lightpath":enum32{"EYE", "L100", "R100", "L80"}}
  T10 = cluster{"Z end":dbl, "Step Num":i32, "Step Size":dbl, "Z0":dbl, "z-stack?":bool}
  T11 = cluster{"Take?":bool[], "Channel":i32[], "Exposure time (msec)":dbl[], "Cumulation":i32[], "Name":string[]}
  T12 = cluster{"Tiling?":bool, "YY/XX":i32[], "X0Y0":dbl[]}
  T13 = cluster{"Lasers":bool[], "Patch":bool, "Camera Output":bool}
  T14 = cluster{"Waveform folder":path, "Exposure time (ms)":dbl}
  T15 = cluster{"samples":i32, "Duration (sec)":dbl, "Downsampling factor":dbl}
  T16 = cluster{"Amplitude (mV)":dbl, "Number of repeats":i32, "DAQ rate (Hz)":dbl, "Frequency (Hz)":dbl}
  T17 = cluster{"Ra (MΩ)":dbl, "Rm (MΩ)":dbl, "Cm (pF)":dbl, "RC constant (msec)":dbl, "Steady state current (pA)":dbl}
  T18 = cluster{"DAQ ports":cluster{"Lasers DO lines":tag[], "Lasers AO lines":tag[], "Patch AO line":tag, "Patch AI lines 1":cluster{"Patch scaled output":tag, "Patch 10 V_m ":tag}, "Camera timing DI":tag, "Dev1 timing DO ":tag, "Dev1 trigger source":tag, "Dev2 trigger source":tag, "LED line":tag, "Global Shutter line":tag, "Patch AI lines 2":cluster{"Cell capacitance":tag, "Mode":tag, "Frequency":tag, "Gain":tag}}, "Camera Setting":cluster{"Camera Output triger mode setiting":cluster{"Mode":u32, "Polarity":u32, "Period":dbl, "Delay":dbl}, "Camera timing port for trigering":enum16{"1", "2", "3"}}, "Stage setting":cluster{"Baudrate":i32, "COM Port":string, "Xmax":dbl, "Xmin":dbl, "Ymax":dbl, "Ymin":dbl}, "Confocal VISA Setting":refnum<visa-resource-name>}
  T19 = cluster{"Camera Details Array":cluster{"Model":string, "Camera ID":string, "Firmware":string}[], "Handle":u32, "Camera in use ":cluster{"Model":string, "Camera ID":string, "Bits":i32}}
  T20 = cluster{"Actual Disk speed (rpm)":string, "Actual FW speed (rpm)":i32}
  T21 = cluster{"TI":refnum<k7>, "Nosepiece":refnum<k7>, "LightPathDrive":refnum<k7>, "ZDrive":refnum<k7>, "PFS":refnum<k7>, "CondenserCassette":refnum<k7>, "FilterBlockCassette1":refnum<k7>, "FilterBlockCassette2":refnum<k7>}
  T22 = cluster{"width":u32, "height":u32, "datatype":u32}
  T23 = enum8{"Enabled", "Disabled", "Disabled and Grayed Out"}
  T24 = cluster{"SDC shutter":bool, "FWPosition":i32, "FW speed":i32, "Disk spinning?":bool, "Disk speed (rpm)":dbl}
  T25 = cluster{"Lasers DO lines":tag[], "Lasers AO lines":tag[], "Patch AO line":tag, "Patch AI lines 1":cluster{"Patch scaled output":tag, "Patch 10 V_m ":tag}, "Camera timing DI":tag, "Dev1 timing DO ":tag, "Dev1 trigger source":tag, "Dev2 trigger source":tag, "LED line":tag, "Global Shutter line":tag, "Patch AI lines 2":cluster{"Cell capacitance":tag, "Mode":tag, "Frequency":tag, "Gain":tag}}
  T26 = cluster{"Baudrate":i32, "COM Port":string, "Xmax":dbl, "Xmin":dbl, "Ymax":dbl, "Ymin":dbl}
  T27 = cluster{"LEFT":bool, "RIGHT":bool, "FWD":bool, "BACK":bool}
  T28 = cluster{"Total x width (μm)":refnum<vi>, "Total y width (μm)":refnum<vi>, "Pixel size (nm)":refnum<vi>, "scale bar (μm)":refnum<vi>}
  T29 = cluster{"Ra (Mohm)":dbl, "Rm (Mohm)":dbl, "Cm (pF)":dbl, "RC constant (msec)":dbl, "Steady state current (pA)":dbl}
  T30 = cluster{"max value":u16, "mean":i16, "min value":u16, "Histogram":cluster{"X Values":dbl[], "Histogram: h(x)":i32[]}}
  T31 = cluster{"Camera Output triger mode setiting":cluster{"Mode":u32, "Polarity":u32, "Period":dbl, "Delay":dbl}, "Camera timing port for trigering":enum16{"1", "2", "3"}}
  T32 = cluster{"Model":string, "Camera ID":string, "Bits":i32}
  T33 = cluster{"Lasers DO lines":tag[], "Lasers AO lines":tag[], "Patch AO line":tag, "Patch AI lines":tag[], "Dev1 timing DO":tag, "Camera timing DI":tag, "Dev1 trigger source":tag, "Dev2 trigger source":tag}
  T34 = cluster{"Sampling rate (Hz)":dbl, "dt (sec)":dbl, "total time (sec)":dbl, "# samples":i32, "Exposure time (ms)":dbl, "# frames":i32}
  T35 = cluster{"TI-Ctrl":refnum<vi>, "TiE Ref":cluster{"TI":refnum<k7>, "Nosepiece":refnum<k7>, "LightPathDrive":refnum<k7>, "ZDrive":refnum<k7>, "PFS":refnum<k7>, "CondenserCassette":refnum<k7>, "FilterBlockCassette1":refnum<k7>, "FilterBlockCassette2":refnum<k7>}}
  T36 = cluster{"Filter Set":i32, "Light control":refnum<vi>, "Confocal scanner":refnum<vi>, "Value":cluster{"Lasers DO lines":tag[], "Lasers AO lines":tag[], "Patch AO line":tag, "Patch AI lines 1":cluster{"Patch scaled output":tag, "Patch 10 V_m ":tag}, "Camera timing DI":tag, "Dev1 timing DO ":tag, "Dev1 trigger source":tag, "Dev2 trigger source":tag, "LED line":tag, "Global Shutter line":tag, "Patch AI lines 2":cluster{"Cell capacitance":tag, "Mode":tag, "Frequency":tag, "Gain":tag}}, "Value":refnum<visa-resource-name>}
  T37 = cluster{"XY tiling":cluster{"Tiling?":bool, "YY/XX":i32[], "X0Y0":dbl[]}, "Stage Status":refnum<vi>}
  T38 = cluster{i32, "appended path":path, "Z-Stack":cluster{"Z end":dbl, "Step Num":i32, "Step Size":dbl, "Z0":dbl, "z-stack?":bool}, "Arch_Dragon cumulation":i32, "Image Info":refnum<vi>, "Camera Ctrl":cluster{"Chosen Camera":u32, "ROI selection":u16, "Live":bool, "ROI define":bool, "Snap":bool, "ROI update":bool, "ROI previous ":bool, "ROI":cluster{"Bin":u16, "ROI":cluster{"x offset":i32, "y offset":i32, "x width":i32, "y width":i32}}, "Exposure (ms)":dbl, "Symmetrical":bool, "Autoscale":bool, "Scale":cluster{"Scale.Min":i32, "Scale.Max":i32}}}
  T39 = cluster{"NewVal":i32, "Light control":refnum<vi>, "Confocal scanner":refnum<vi>, "Value":cluster{"Lasers DO lines":tag[], "Lasers AO lines":tag[], "Patch AO line":tag, "Patch AI lines 1":cluster{"Patch scaled output":tag, "Patch 10 V_m ":tag}, "Camera timing DI":tag, "Dev1 timing DO ":tag, "Dev1 trigger source":tag, "Dev2 trigger source":tag, "LED line":tag, "Global Shutter line":tag, "Patch AI lines 2":cluster{"Cell capacitance":tag, "Mode":tag, "Frequency":tag, "Gain":tag}}, "Value":refnum<visa-resource-name>}
  T40 = cluster{"Obj":u16, "Cube 1":u16, "Cube 2":u16, "PFS-Ctrl":cluster{"PFS IO":bool, "PSF Err":bool, "PSF Pos":u32}, "Z-Ctrl":cluster{"Z-pos":dbl, "Home":bool, "Sensitivity":u8}, "Condenser":u16, "Lightpath":enum32{"EYE", "L100", "R100", "L80"}}
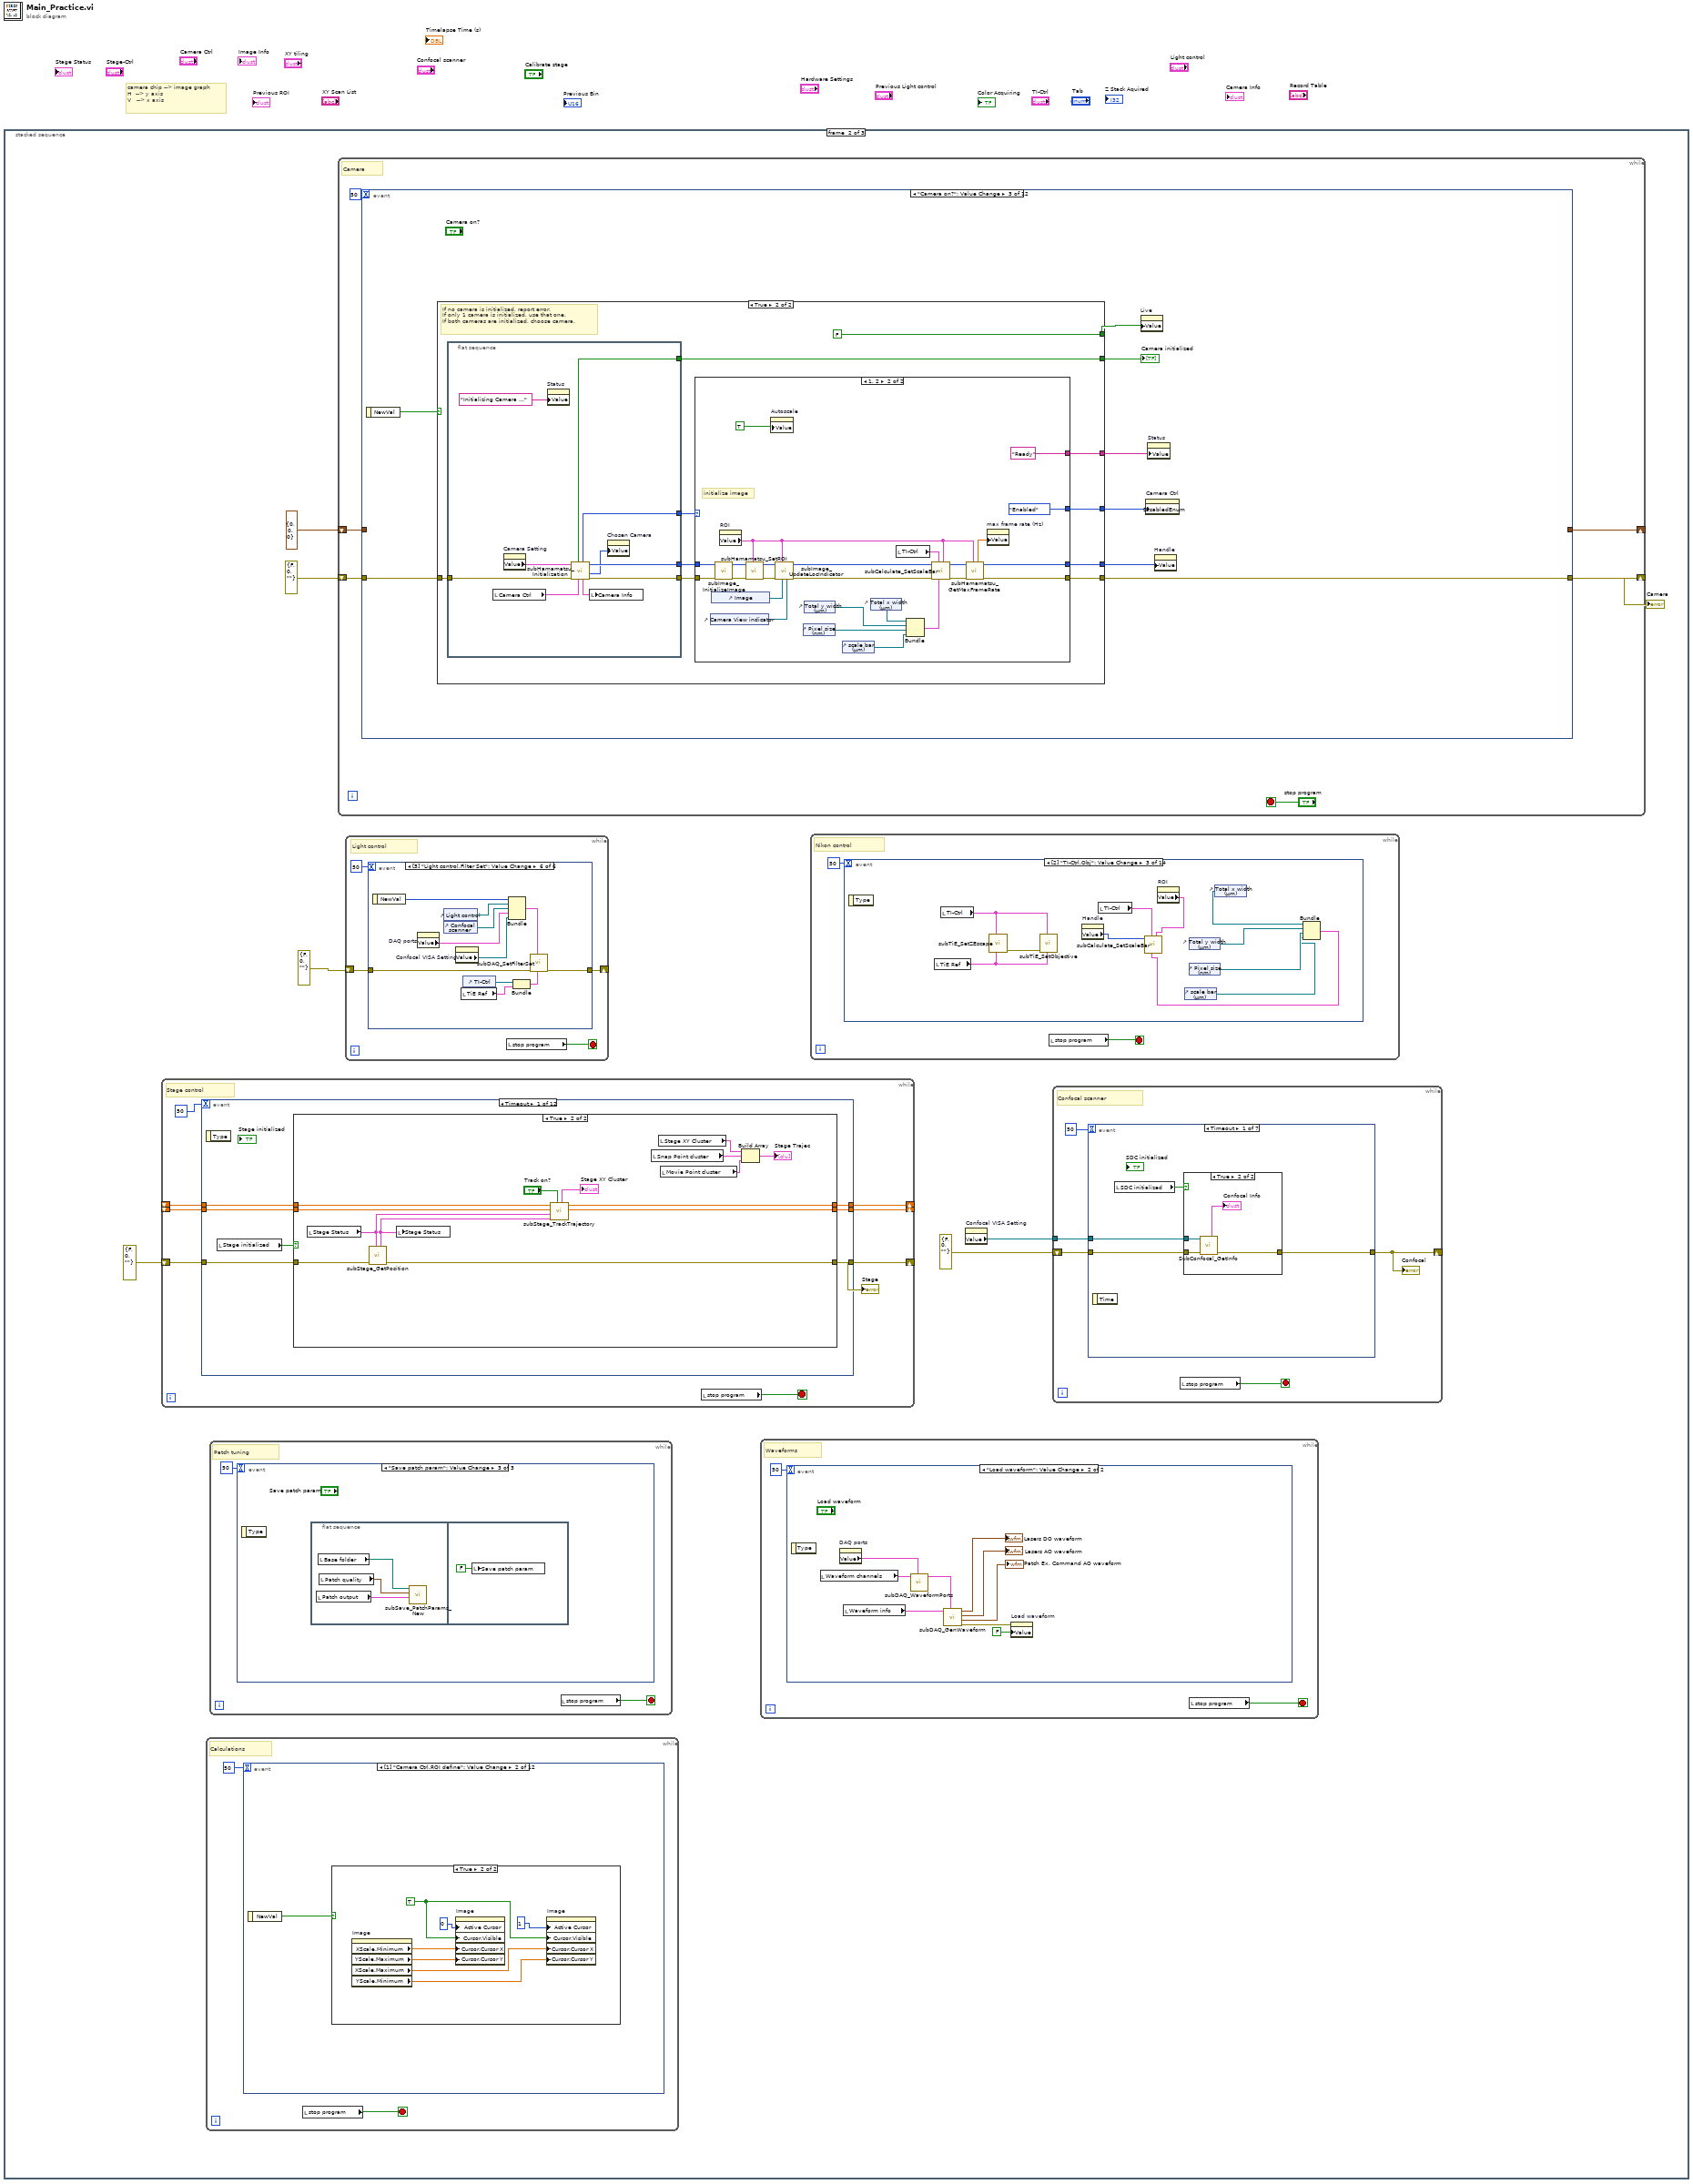
[diagram p0: block diagram]
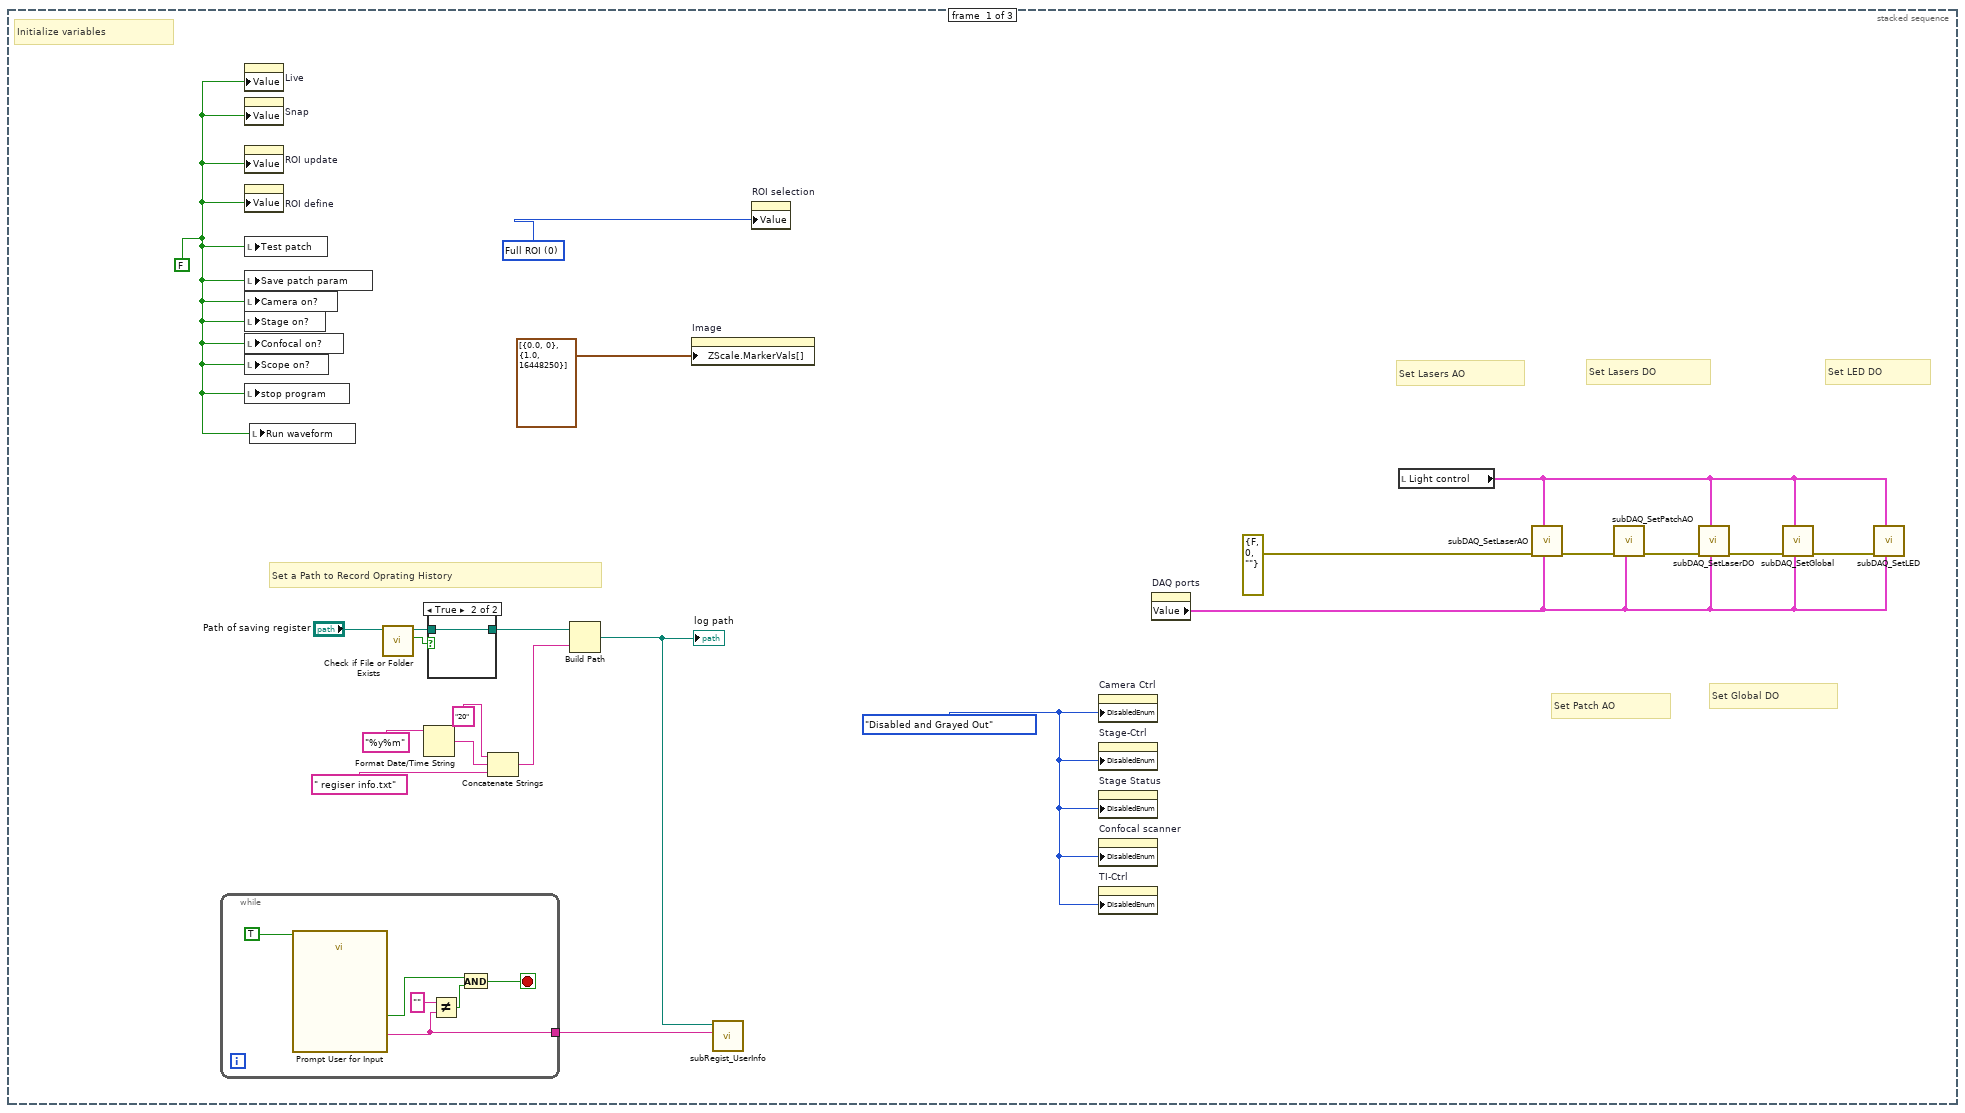
[diagram p2: hidden frame]
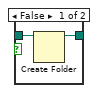
[diagram p3: hidden frame]
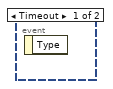
[diagram p4: hidden frame]
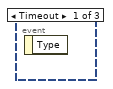
[diagram p5: hidden frame]
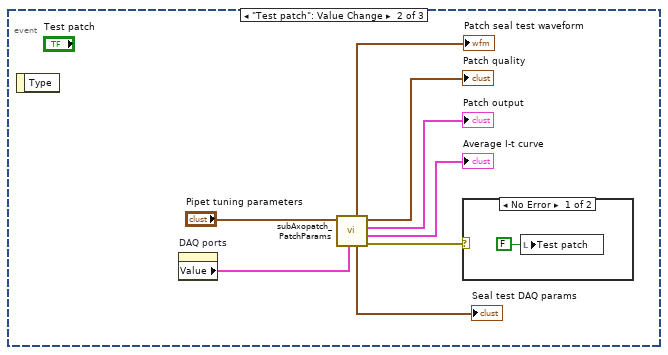
[diagram p6: hidden frame]
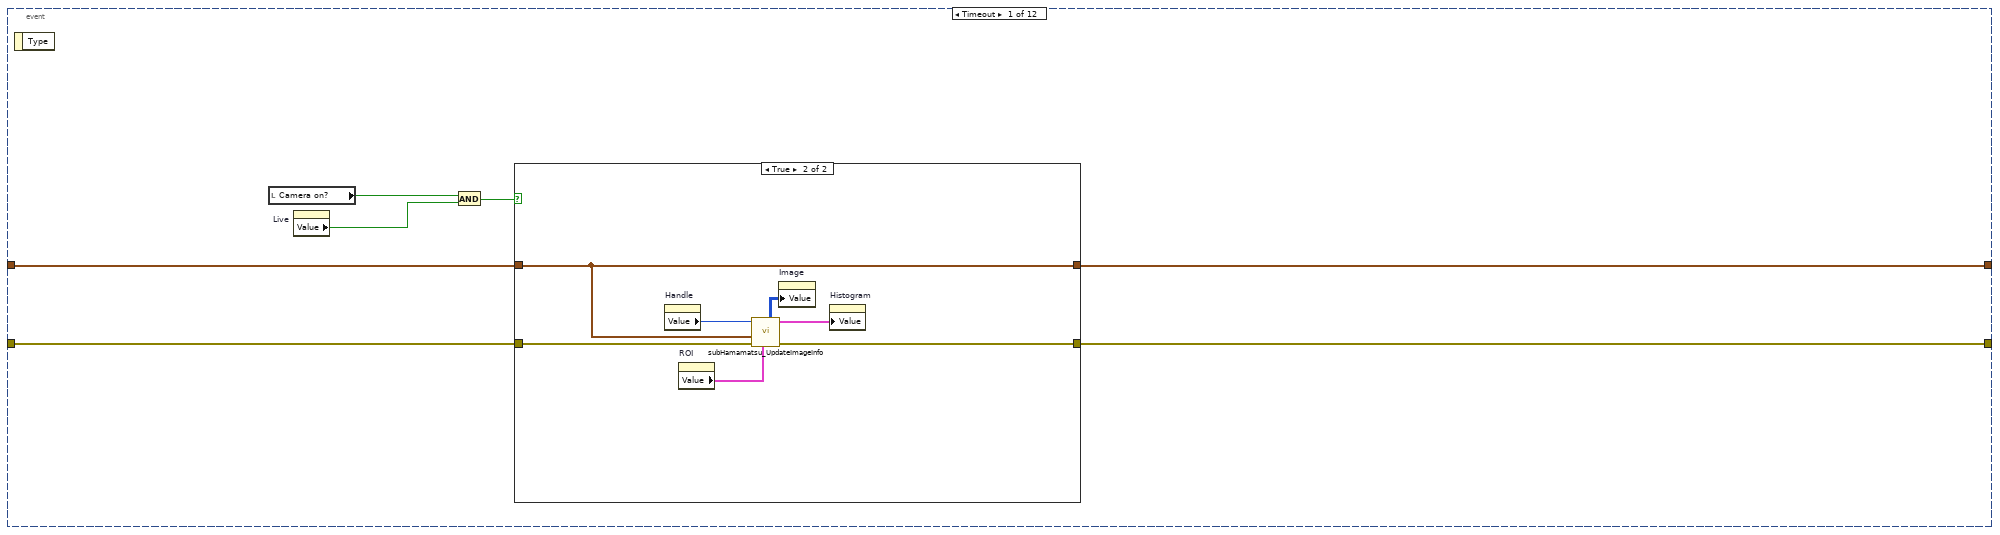
[diagram p8: hidden frame]
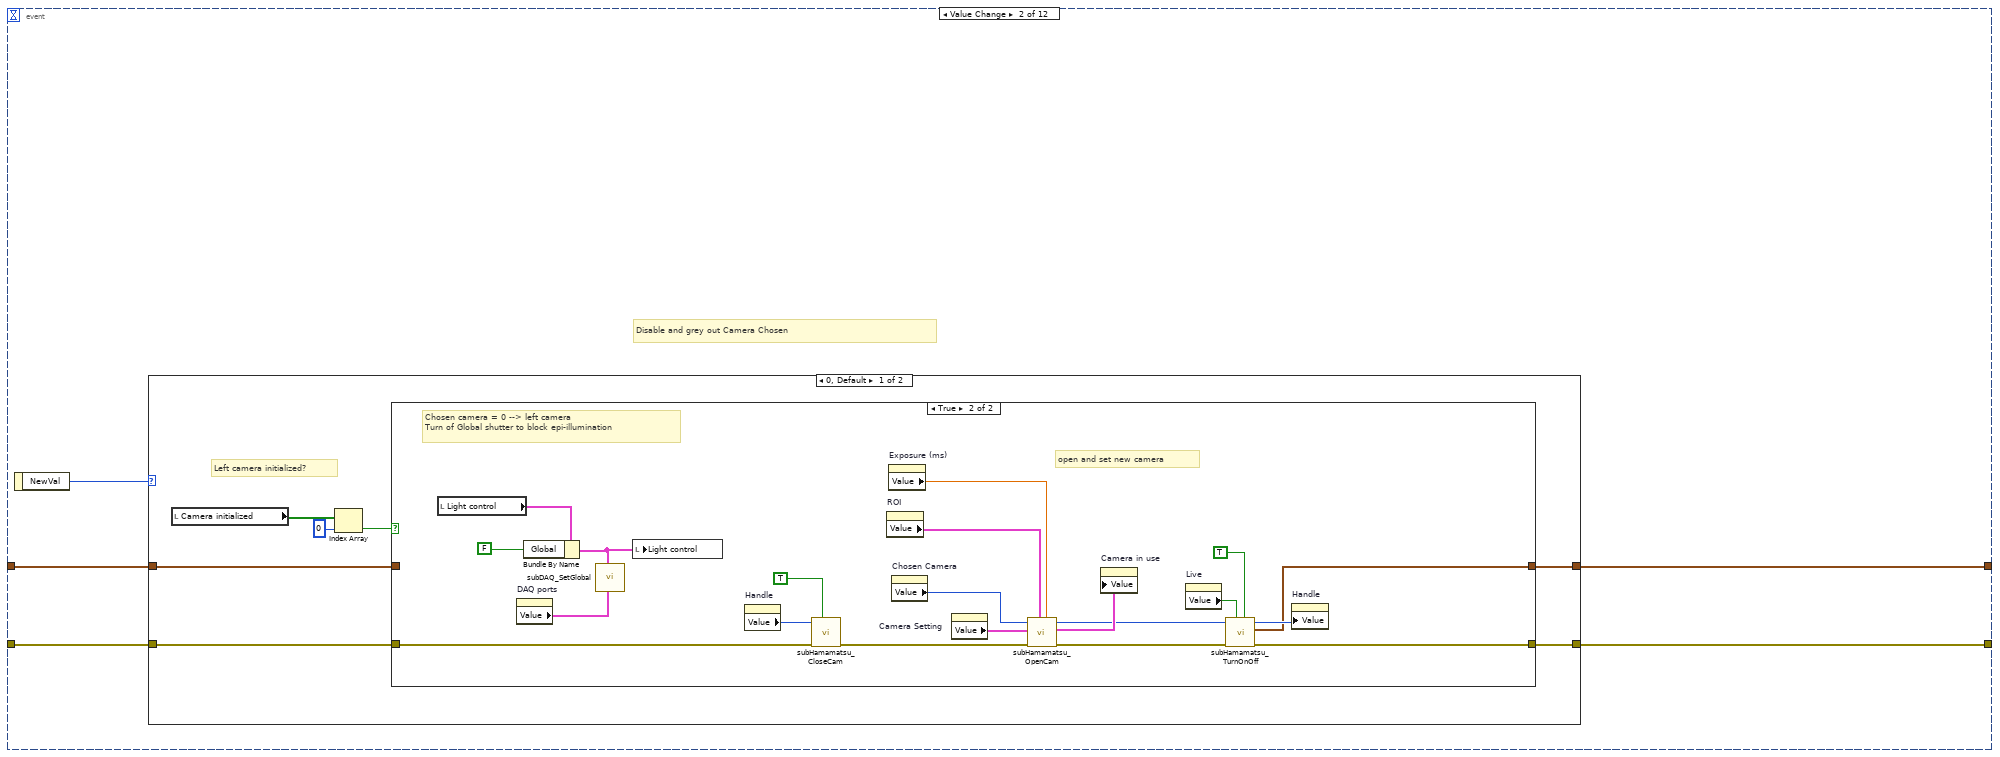
[diagram p10: hidden frame]
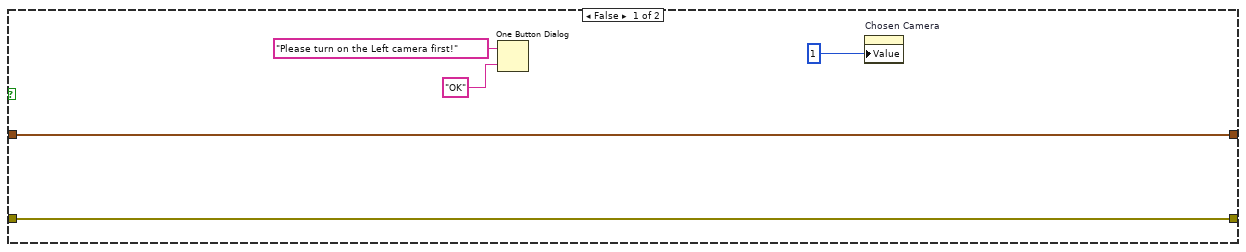
[diagram p11: hidden frame]
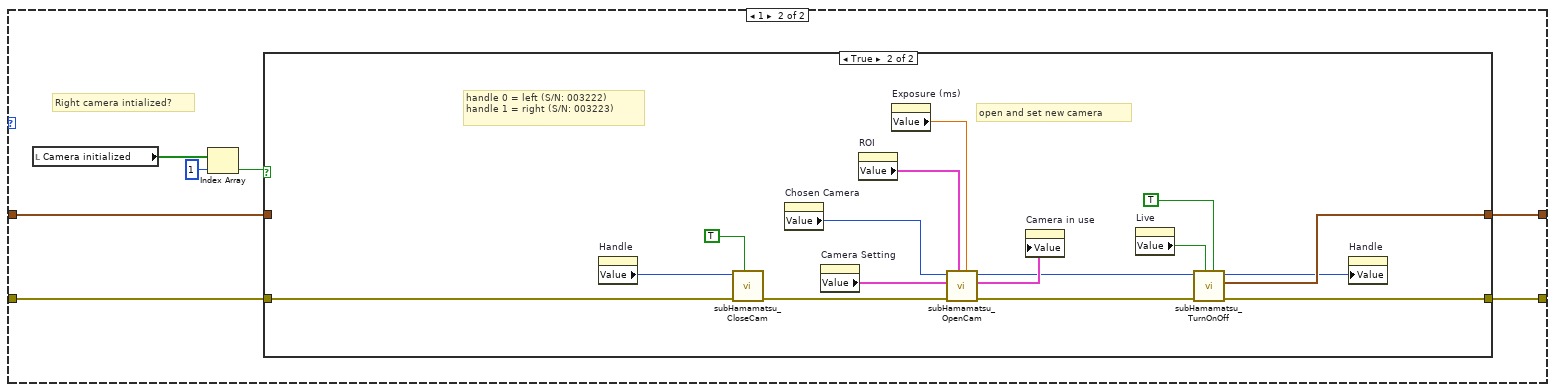
[diagram p12: hidden frame]
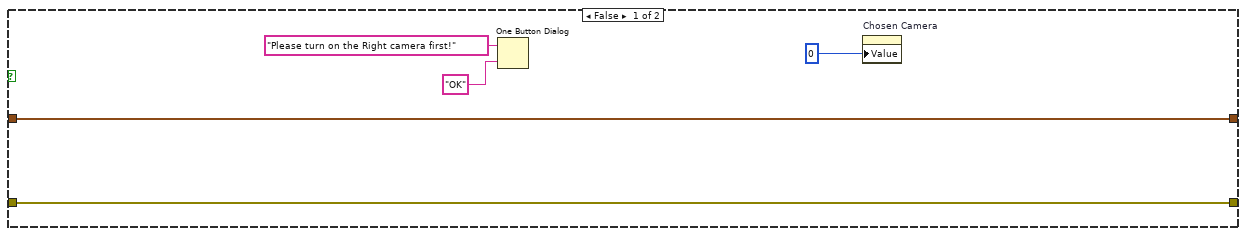
[diagram p13: hidden frame]
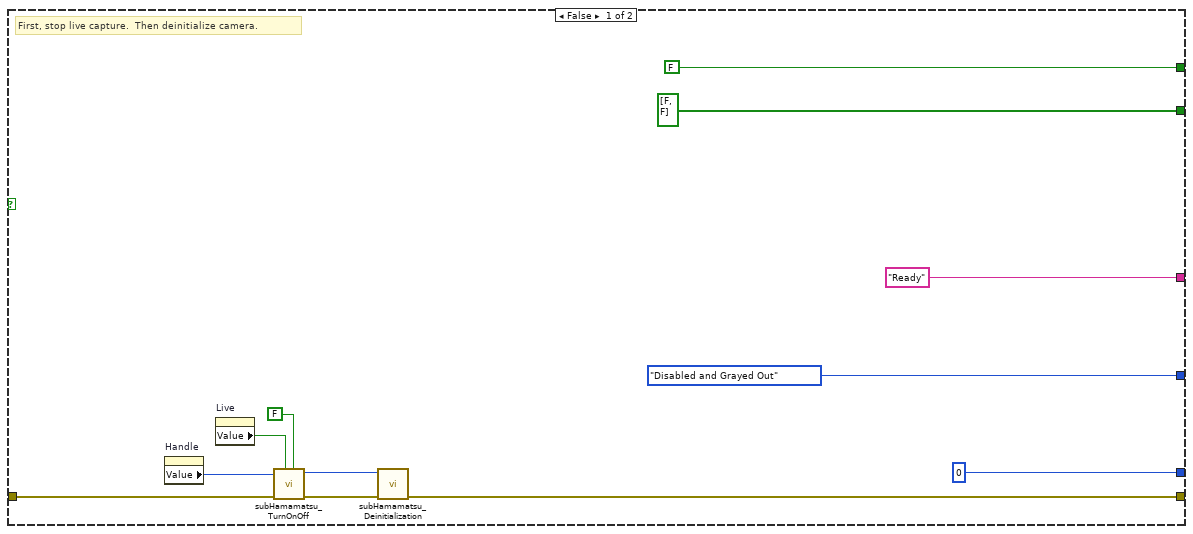
[diagram p14: hidden frame]
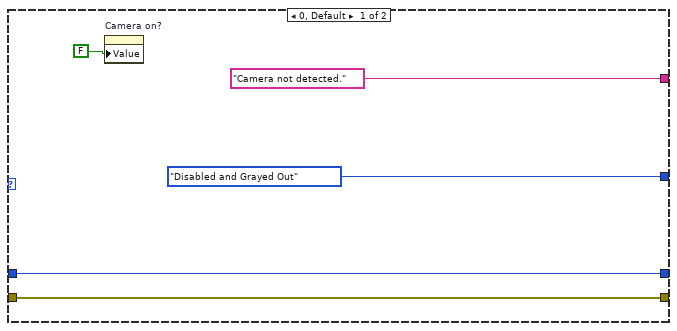
[diagram p15: hidden frame]
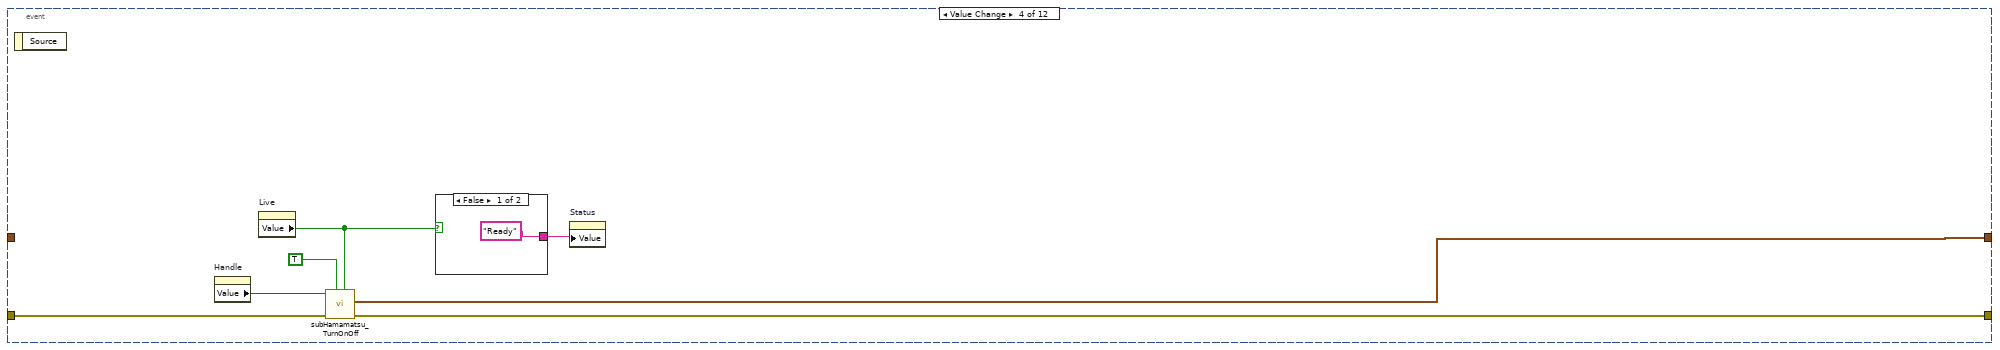
[diagram p16: hidden frame]
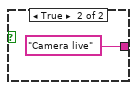
[diagram p17: hidden frame]
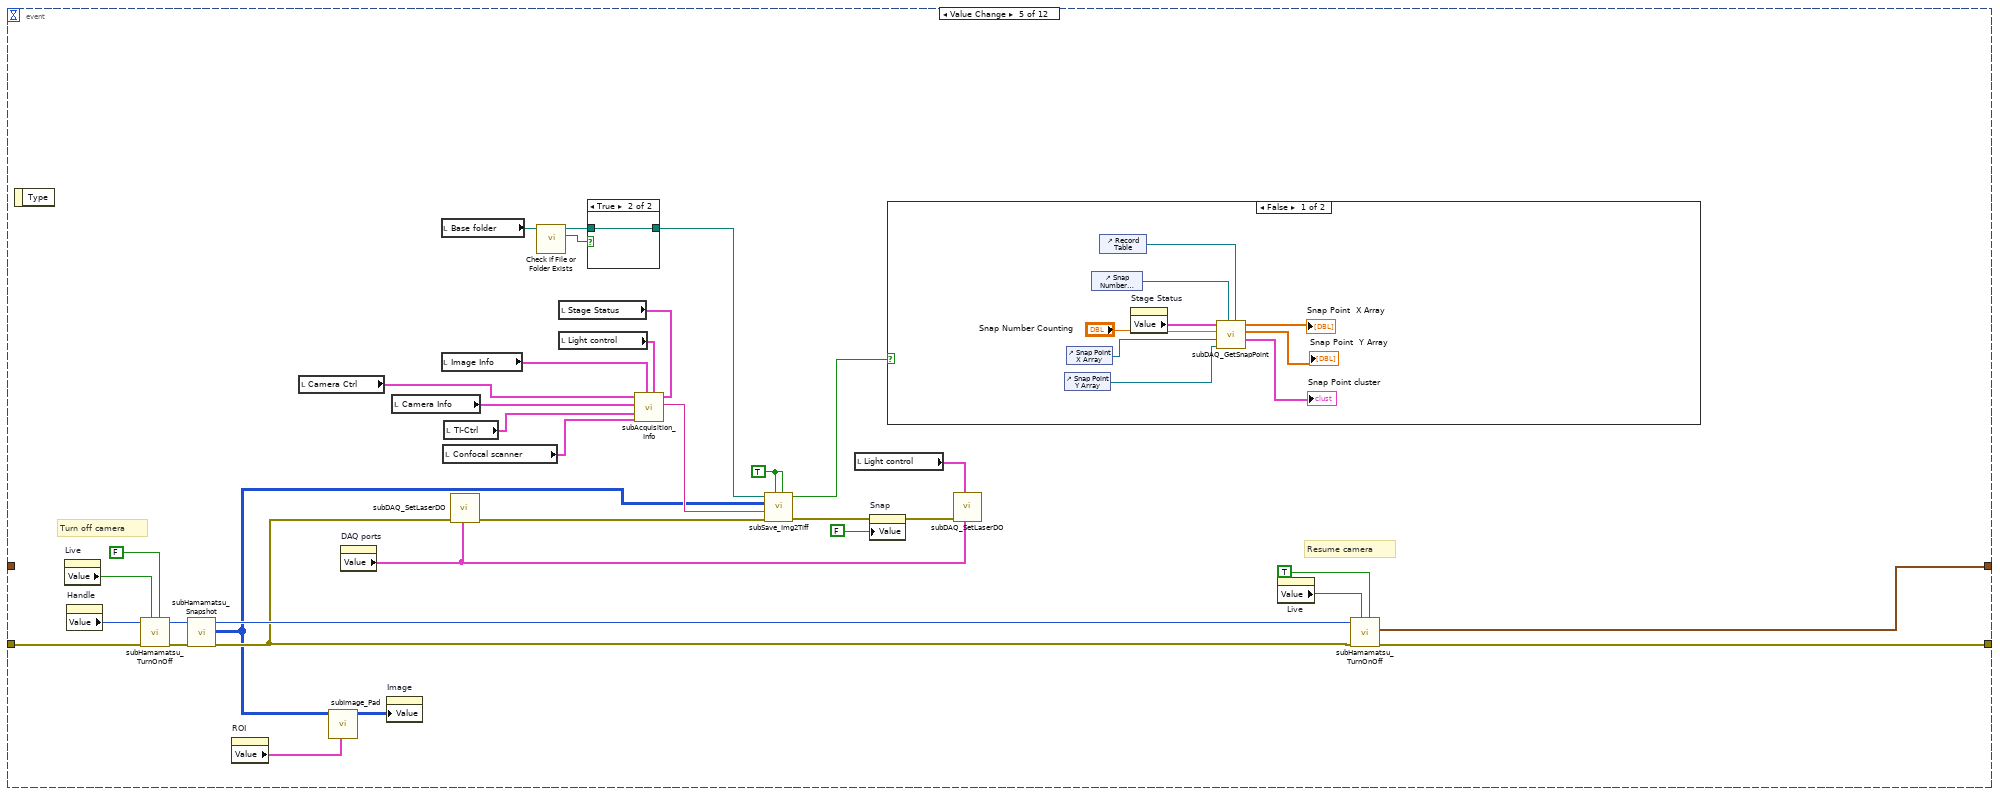
[diagram p18: hidden frame]
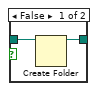
[diagram p20: hidden frame]
diagram:
  # "camera chip --> image graph\nH  --> y axis\nV   --> x axis"
  n1 = stacked-sequence {
    frame #0 {
      w5 = T23."Disabled and Grayed Out" ("Disabled")
      w3 = u16 0 items=["Full ROI", "Central quad", "Custom ROI"] ("ROI selection")
      w4 = FALSE ("stop program")
      # "Set LED DO"
      # "Set Global DO"
      # "Set Patch AO"
      # "Set Lasers DO"
      # "Set Lasers AO"
      # "Set a Path to Record Oprating History"
      # "Initialize variables"
      n2 = while {
        tunnel: [w23] -> w20
        stop <- w24 stop-if-true
        n3 = call "Prompt User for Input"("Enable"=TRUE) -> ("Name"=w23:string, "OK"=w28:bool)  [unwired: 16 in, 1 out]
        n4 = Not Equal?(x="", y=w23) -> (x != y?=w27:bool)
        n5 = And(x=w28, y=w27) -> (x .and. y?=w24:bool)
      }
      n6 = property on="Live" class="Bool (strict)"("Value"=w4) -> ()  [unwired: 2 in, 2 out]
      n7 = property on="Snap" class="Bool (strict)"("Value"=w4) -> ()  [unwired: 2 in, 2 out]
      n8 = property on="ROI update" class="Bool (strict)"("Value"=w4) -> ()  [unwired: 2 in, 2 out]
      n9 = property on="ROI define" class="Bool (strict)"("Value"=w4) -> ()  [unwired: 2 in, 2 out]
      n10 = local write "Test patch"(w4) -> ()
      n11 = local write "Save patch param"(w4) -> ()
      n12 = local write "Camera on?"(w4) -> ()
      n13 = local write "Stage on?"(w4) -> ()
      n14 = local write "Confocal on?"(w4) -> ()
      n15 = local write "Scope on?"(w4) -> ()
      n16 = local write "stop program"(w4) -> ()
      n17 = local write "Run waveform"(w4) -> ()
      n18 = call <vilib>:"Check if File or Folder Exists.vi"("path"="Path of saving register") -> ("file or folder exists?"=w21:bool, "dup path"=w22:path)  [unwired: 8 in, 1 out]
      n19 = Format Date/Time String(time format string (%c)="%y%m") -> (date/time string=w18:string)  [unwired: 2 in]
      n20 = case shown="True" w21 {
        tunnel: w22 -> [w30 w31]
        tunnel: [w29 w31] -> w14
        frame False {
          n21 = Create Folder(path (use dialog)=w30) -> (created path=w29:path)  [unwired: 2 in, 2 out]
        }
        frame True {
        }
      }
      n22 = Concatenate Strings("20" ("string"), w18, " regiser info.txt" ("string")) -> (w17:string)
      n23 = Build Path(base path=w14, name or relative path=w17) -> (appended path=w6:path)
      "log path" <- w6
      n24 = property on="Image" class="IntGraph (strict)"("ZScale.MarkerVals[]"=cluster{dbl, u32}[] [{0.0, 0}, {1.0, 16448250}] ("Z Scale.Marker Values[]")) -> ()  [unwired: 2 in, 2 out]
      n25 = call "subRegist_UserInfo.vi"("user name"=w20, "log path"=w6) -> ()  [unwired: 10 in]
      n26 = property on="ROI selection" class="Ring (strict)"("Value"=w3) -> ()  [unwired: 2 in, 2 out]
      n27 = property on="Camera Ctrl" class="Clust (strict)"("DisabledEnum"=w5) -> ()  [unwired: 2 in, 2 out]
      n28 = property on="Stage-Ctrl" class="Clust (strict)"("DisabledEnum"=w5) -> ()  [unwired: 2 in, 2 out]
      n29 = property on="Stage Status" class="Clust (strict)"("DisabledEnum"=w5) -> ()  [unwired: 2 in, 2 out]
      n30 = property on="Confocal scanner" class="Clust (strict)"("DisabledEnum"=w5) -> ()  [unwired: 2 in, 2 out]
      n31 = property on="TI-Ctrl" class="Clust (strict)"("DisabledEnum"=w5) -> ()  [unwired: 2 in, 2 out]
      n32 = property on="DAQ ports" class="Clust (strict)"() -> ("Value"=w1:T25)  [unwired: 2 in, 2 out]
      n33 = local read "Light control"() -> (w7:T1)
      n34 = call "subDAQ_SetLaserAO.vi"("DAQ ports"=w1, "Light control (All off)"=w7, "Error in (no error)"=errorcluster {"status"=FALSE, "code"=0, "source"=""} ("error out")) -> ("Error out"=w11:errorcluster)  [unwired: 8 in]
      n35 = call "subDAQ_SetPatchAO.vi"("DAQ ports"=w1, "Error in (no error)"=w11) -> ("Error out"=w10:errorcluster)  [unwired: 9 in]
      n36 = call "subDAQ_SetLaserDO.vi"("DAQ ports"=w1, "Light control (All off)"=w7, "Error in (no error)"=w10) -> ("Error out"=w9:errorcluster)  [unwired: 8 in]
      n37 = call "subDAQ_SetGlobal.vi"("DAQ ports"=w1, "Light control (All off)"=w7, "Error in (no error)"=w9) -> ("Error out"=w8:errorcluster)  [unwired: 8 in]
      n38 = call "subDAQ_SetLED.vi"("DAQ ports"=w1, "Light control (All Off)"=w7, "Error in (no error)"=w8) -> ()  [unwired: 8 in, 1 out]
    }
    frame #1 {
      n39 = while {
        shift-right: [w786] -> _
        shift-left: errorcluster {"status"=FALSE, "code"=0, "source"=""} ("Error out") -> [w788]
        shift-right: [w785] -> _
        shift-left: _ -> [w784]
        shift-right: [w783] -> _
        shift-left: _ -> [w782]
        stop <- w787 stop-if-true
        # "Stage control"
        n40 = event shown="[0] Timeout" {
          selector: _ -> [_ _ _ _ _ _ _ _ _ _ _ _]
          dyn-events: _ -> [_ _ _ _ _ _ _ _ _ _ _ _]
          timeout: 50 -> [_ _ _ _ _ _ _ _ _ _ _ _]
          tunnel: w788 -> [w796 _ w824 w835 w841 w850 w860 w868 w875 w900 w920 w927]
          tunnel: [w795 _ w822 w833 w846 w847 w856 w864 w877 w896 w916 w925] -> w786
          tunnel: [w793 _ w817 w837 w843 w852 w861 w869 _ w892 w911 w921] -> w785
          tunnel: w784 -> [w792 _ w817 w837 w843 w852 w861 w869 _ w892 w911 w921]
          tunnel: [w791 _ w818 w838 w844 w853 w862 w870 _ w893 w912 w922] -> w783
          tunnel: w782 -> [w790 _ w818 w838 w844 w853 w862 w870 _ w893 w912 w922]
          event Timeout {
            n41 = event-data() -> ()  [unwired: 1 in, 1 out]
            n42 = local read "Stage initialized"() -> (w794:bool)
            n43 = case shown="True" w794 {
              tunnel: w796 -> [w799 w812]
              tunnel: [w799 w813] -> w795
              tunnel: [w797 w806] -> w793
              tunnel: w792 -> [w797 w809]
              tunnel: [w798 w807] -> w791
              tunnel: w790 -> [w798 w808]
              frame False {
              }
              frame True {
                n44 = local read "Stage Status"() -> (w810:T7)
                n45 = call "subStage_GetPosition.vi"("Stage Info In"=w810, "Error In"=w812) -> ("Error out"=w813:errorcluster, "Stage Info Out"=w811:T7)  [unwired: 8 in]
                n46 = local write "Stage Status"(w811) -> ()
                n47 = call "subStage_TrackTrajectory.vi"("Track on?"="Track on?", "Stage Current Status"=w811, "Stage Previous Status"=w810, "Stage X Array In"=w809, "Stage Y Array In"=w808) -> ("Stage X Array Out"=w806:dbl[], "Stage Y Array Out"=w807:dbl[], "Stage XY Cluster"=→"Stage XY Cluster":cluster{dbl[], dbl[]})  [unwired: 4 in]
                n48 = local read "Snap Point cluster"() -> (w802:cluster{"Snap Y":dbl[], "Snap X":dbl[]})
                n49 = local read "Stage XY Cluster"() -> (w803:cluster{"Stage Y ":dbl[], "Stage X":dbl[]})
                n50 = local read "Movie Point cluster"() -> (w801:cluster{"Movie Y":dbl[], "Movie X":dbl[]})
                n51 = Build Array(w803, w802, w801) -> (→"Stage Trajec":cluster{"Movie Y":dbl[], "Movie X":dbl[]}[])
              }
            }
          }
          event "Track on?": Value Change {
            w815 = dbl[] [] ("Movie Point  X Array")
            w816 = cluster{dbl[], dbl[]} {[], []}
            n52 = event-data() -> ()  [unwired: 1 in, 1 out]
            n53 = property on="Snap Point cluster" class="Clust (strict)"("Value"=w816) -> ()  [unwired: 2 in, 2 out]
            n54 = property on="Stage XY Cluster" class="Clust (strict)"("Value"=w816) -> ()  [unwired: 2 in, 2 out]
            n55 = property on="Movie Point cluster" class="Clust (strict)"("Value"=w816) -> ()  [unwired: 2 in, 2 out]
            n56 = property on="Movie Point  X Array" class="Arr (strict)"("Value"=w815) -> ()  [unwired: 2 in, 2 out]
            n57 = property on="Movie Point  Y Array" class="Arr (strict)"("Value"=w815) -> ()  [unwired: 2 in, 2 out]
            n58 = property on="Snap Number Counting" class="DigNum (strict)"("Value"=0.0 ("Snap Number Counting")) -> ()  [unwired: 2 in, 2 out]
            n59 = property on="Snap Point  X Array" class="Arr (strict)"("Value"=w815) -> ()  [unwired: 2 in, 2 out]
            n60 = property on="Snap Point  Y Array" class="Arr (strict)"("Value"=w815) -> ()  [unwired: 2 in, 2 out]
          }
          event "Clear Table": Value Change {
            n61 = event-data() -> ()  [unwired: 1 in, 1 out]
            n62 = Two Button Dialog(message="Are you sure to clear this table?\nPlease write the tabel to Excel first.") -> (T button?=w819:bool)  [unwired: 2 in]
            n63 = case shown="True" w819 {
              tunnel: w824 -> [w825 w829]
              tunnel: [w825 w827] -> w823
              frame False {
              }
              frame True {
                w826 = string[][] [] ("Record Table")
                n64 = property on="Record Table" class="Tbl (strict)"(error in=w829, "Value"=w826) -> (error out=w828:errorcluster)  [unwired: 1 in, 1 out]
                n65 = property on="XY Scan List" class="Tbl (strict)"(error in=w828, "Value"=w826) -> (error out=w827:errorcluster)  [unwired: 1 in, 1 out]
              }
            }
            n66 = property on="Clear Table" class="Bool (strict)"(error in=w823, "Value"=FALSE ("Clear Table")) -> (error out=w822:errorcluster)  [unwired: 1 in, 1 out]
          }
          event "Goto destination": Value Change {
            n67 = event-data() -> ()  [unwired: 1 in, 1 out]
            n68 = local read "Record Table"() -> (w830:string[][])
            n69 = property on="ILSID" class="DigNum (strict)"() -> ("Value"=w832:i32)  [unwired: 2 in, 2 out]
            n70 = call "subStage_GotoAccordingtoTable.vi"("Record Table"=w830, "error in (no error)"=w835, "ILSID"=w832, "Number"="Number") -> ("error out"=w834:errorcluster)  [unwired: 7 in]
            n71 = property on="Goto destination" class="Bool (strict)"(error in=w834, "Value"=FALSE ("Goto destination")) -> (error out=w833:errorcluster)  [unwired: 1 in, 1 out]
          }
          event "Write table to excel": Value Change {
            n72 = event-data() -> ()  [unwired: 1 in, 1 out]
            n73 = local read "Excel Loading Path"() -> (w839:path)
            n74 = local read "Record Table"() -> (w842:string[][])
            n75 = call "SubStage_WriteTableToExcel.vi"("Record Table"=w842, "error in (no error)"=w841, "Path"=w839) -> ("error out"=w840:errorcluster)  [unwired: 8 in]
            n76 = property on="Write table to excel" class="Bool (strict)"(error in=w840, "Value"=FALSE ("Write table to excel")) -> (error out=w846:errorcluster)  [unwired: 1 in, 1 out]
          }
          event "Load Excel to table": Value Change {
            n77 = event-data() -> ()  [unwired: 1 in, 1 out]
            n78 = call "subStage_ReadExcelToTable.vi"("error in (no error)"=w850, "File Path"="Excel Loading Path") -> ("error out"=w848:errorcluster, "Record Table"=w851:string[][])  [unwired: 8 in]
            n79 = local write "Record Table"(w851) -> ()
            n80 = property on="Load Excel to table" class="Bool (strict)"(error in=w848, "Value"=FALSE ("Load Excel to table")) -> (error out=w847:errorcluster)  [unwired: 1 in, 1 out]
          }
          event "Load from table (For XY Scan)": Value Change {
            n81 = event-data() -> ()  [unwired: 1 in, 1 out]
            n82 = property on="Record Table" class="Tbl (strict)"(error in=w860) -> (error out=w859:errorcluster, "Value"=w858:string[][])  [unwired: 1 in, 1 out]
            n83 = property on="XY Scan List" class="Tbl (strict)"(error in=w859, "Value"=w858) -> (error out=w857:errorcluster)  [unwired: 1 in, 1 out]
            n84 = property on="Load from table (For XY Scan)" class="Bool (strict)"(error in=w857, "Value"=FALSE ("Load from table (For XY Scan)")) -> (error out=w856:errorcluster)  [unwired: 1 in, 1 out]
          }
          event "Load from Exel (For XY Scan)": Value Change {
            n85 = event-data() -> ()  [unwired: 1 in, 1 out]
            n86 = local read "Excel Loading Path"() -> (w866:path)
            n87 = call "subStage_ReadExcelToTable.vi"("error in (no error)"=w868, "File Path"=w866) -> ("error out"=w865:errorcluster, "Record Table"=w867:string[][])  [unwired: 8 in]
            n88 = local write "XY Scan List"(w867) -> ()
            n89 = property on="Load from Exel (For XY Scan)" class="Bool (strict)"(error in=w865, "Value"=FALSE ("Load Excel to table")) -> (error out=w864:errorcluster)  [unwired: 1 in, 1 out]
          }
          event "Stage on?": Value Change {
            n90 = event-data() -> ("NewVal"=w876:bool)  [unwired: 1 in]
            n91 = case shown="False" w876 {
              tunnel: [w881 w889] -> w877
              tunnel: w875 -> [w880 w890]
              tunnel: [T23."Disabled and Grayed Out" ("Disabled") T23."Enabled" ("Disabled")] -> w874
              tunnel: [FALSE w888] -> w873
              tunnel: [T23."Disabled and Grayed Out" ("Disabled") T23."Enabled" ("Disabled")] -> w872
              tunnel: [T7 {" Current Position"=[-1.0, -12.0, 0.0], "Number of Axis"=3, "ILSID"=1} ("Stage Info") w886] -> w871
              frame False {
                n92 = local read "Stage Status"() -> (w879:T7)
                n93 = call "Disconnect.vi"("Stage Info"=w879, "Error In"=w880) -> ("Error out"=w881:errorcluster)  [unwired: 9 in]
              }
              frame True {
                n94 = property on="Stage setting" class="Clust (strict)"() -> ("Value"=w885:T26)  [unwired: 2 in, 2 out]
                n95 = call "subStage_Initialize.vi"("Stage setting"=w885, "Error In"=w890) -> ("Error out"=w889:errorcluster, "Stage initialized"=w888:bool, "Stage Info"=w886:T7)  [unwired: 7 in]
              }
            }
            n96 = property on="Stage Status" class="Clust (strict)"("Value"=w871) -> ()  [unwired: 2 in, 2 out]
            n97 = property on="Stage initialized" class="Bool (strict)"("Value"=w873) -> ()  [unwired: 2 in, 2 out]
            n98 = property on="Stage Status" class="Clust (strict)"("DisabledEnum"=w872) -> ()  [unwired: 2 in, 2 out]
            n99 = property on="Stage-Ctrl" class="Clust (strict)"("DisabledEnum"=w874) -> ()  [unwired: 2 in, 2 out]
          }
          event "Stage-Ctrl.Move": Value Change {
            n100 = event-data() -> ()  [unwired: 1 in, 1 out]
            n101 = local read "Stage-Ctrl"() -> (w898:T6)
            n102 = property on="Stage setting" class="Clust (strict)"() -> ("Value"=w894:T26)  [unwired: 2 in, 2 out]
            n103 = call "subStage_MoveLimitation.vi"("Stage-Ctrl"=w898, "Stage setting"=w894) -> ("Allow?"=w902:bool)  [unwired: 9 in]
            n104 = case shown="False" w902 {
              selector: w902 -> [w908 _]
              tunnel: [w908 w909] -> w901
              frame True {
              }
              frame False, Default {
                n105 = Two Button Dialog(message="WARNING: Are you sure?\n It may collide the objective.") -> (T button?=w909:bool)  [unwired: 2 in]
              }
            }
            n106 = local read "Stage Status"() -> (w899:T7)
            n107 = case shown="True" w901 {
              tunnel: w900 -> [w903 w907]
              tunnel: [w903 w906] -> w897
              tunnel: w898 -> [_ w904]
              tunnel: w899 -> [_ w905]
              frame False {
              }
              frame True {
                n108 = call "subStage_MoveAbs.vi"("Stage Info"=w905, "error in (no error)"=w907, "Stage-Ctrl"=w904) -> ("error out"=w906:errorcluster)  [unwired: 8 in]
              }
            }
            n109 = property on="Move" class="Bool (strict)"(error in=w897, "Value"=FALSE ("Move absolute")) -> (error out=w896:errorcluster)  [unwired: 1 in, 1 out]
          }
          event "Calibrate stage": Value Change {
            n110 = event-data() -> ()  [unwired: 1 in, 1 out]
            n111 = local read "TiE Ref"() -> (w914:T21)
            n112 = local read "TI-Ctrl"() -> (w913:T9)
            n113 = call "subTiE_SetZEscape.vi"("Wait for a second? (F)"=TRUE, "Ref"=w914, "TI-Ctrl"=w913, "error in"=w920) -> ("error out"=w919:errorcluster)  [unwired: 7 in]
            n114 = local read "Stage Status"() -> (w918:T7)
            n115 = call "subStage_Calibrate.vi"("Stage Info"=w918, "error in (no error)"=w919) -> ("error out"=w916:errorcluster, "Calibrate"=w917:bool)  [unwired: 7 in]
            n116 = property on="Calibrate stage" class="Bool (strict)"("Value"=w917) -> ()  [unwired: 2 in, 2 out]
          }
          event "Stage-Ctrl.Console": Value Change {
            n117 = event-data() -> ()  [unwired: 1 in, 1 out]
            n118 = local read "Stage Status"() -> (w926:T7)
            n119 = local read "Stage-Ctrl"() -> (w923:T6)
            n120 = call "subStage_MoveRelative.vi"("Stage-Ctrl"=w923, "error in"=w927, "Stage Info"=w926) -> ("error out"=w925:errorcluster, "Console Out"=w924:T27)  [unwired: 7 in]
            n121 = property on="Console" class="Clust (strict)"("Value"=w924) -> ()  [unwired: 2 in, 2 out]
          }
        }
        "Stage" <- w786
        n122 = local read "stop program"() -> (w787:bool)
      }
      n123 = while {
        stop <- w628 stop-if-true
        # "Calculations"
        n124 = event shown="[1] \"Camera Ctrl.ROI define\": Value Change" {
          selector: _ -> [_ _ _ _ _ _ _ _ _ _ _ _]
          dyn-events: _ -> [_ _ _ _ _ _ _ _ _ _ _ _]
          timeout: 50 -> [_ _ _ _ _ _ _ _ _ _ _ _]
          event Timeout {
            n125 = event-data() -> ()  [unwired: 1 in, 1 out]
            n126 = local read "Camera on?"() -> (w630:bool)
            n127 = case shown="True" w630 {
              frame False {
              }
              frame True {
                n128 = property on="ROI define" class="Bool (strict)"() -> ("Value"=w632:bool)  [unwired: 2 in, 2 out]
                n129 = property on="Autoscale" class="Bool (strict)"() -> ("Value"=w631:bool)  [unwired: 2 in, 2 out]
                n130 = case shown="True" w632 {
                  frame False {
                  }
                  frame True {
                    # "set ROI cursor"
                    # "calculate frame rate\nbased on cursor"
                    # "update cursor info"
                    n131 = control-ref of="Image"() -> (w634:refnum<vi>)
                    n132 = property on="ROI" class="Clust (strict)"() -> ("Value"=w637:T3)  [unwired: 2 in, 2 out]
                    n133 = property on="Symmetrical" class="Bool (strict)"() -> ("Value"=w635:bool)  [unwired: 2 in, 2 out]
                    n134 = call "subImage_ApplyCursorLimit.vi"("Symmetrical ROI"=w635, "IntGraph Refnum"=w634, "Current ROI"=w637) -> ("ROI cursor"=w633:T3)  [unwired: 8 in]
                    "ROI cursor" <- w633
                    n135 = call "subHamamatsu_GetMaxFrameRate.vi"("ROI in"=w633) -> ("max frame rate (Hz)"=w636:dbl)  [unwired: 8 in, 2 out]
                    n136 = property on="max frame rate (Hz)" class="DigNum (strict)"("Value"=w636) -> ()  [unwired: 2 in, 2 out]
                  }
                }
                n137 = case shown="False" w631 {
                  frame False {
                    # "update cursor info"
                    n138 = control-ref of="Image"() -> (w640:refnum<vi>)
                    n139 = control-ref of="Histogram"() -> (w639:refnum<vi>)
                    n140 = call "subHistogram_ApplyScaleLimit.vi"("IntGraph Refnum"=w640, "XYGraph Refnum"=w639) -> ("Scale"=w638:cluster{"Scale.Min":i32, "Scale.Max":i32})  [unwired: 8 in, 1 out]
                    n141 = property on="Scale" class="Clust (strict)"("Value"=w638) -> ()  [unwired: 2 in, 2 out]
                  }
                  frame True {
                  }
                }
              }
            }
          }
          event "Camera Ctrl.ROI define": Value Change {
            n142 = event-data() -> ("NewVal"=w641:bool)  [unwired: 1 in]
            n143 = case shown="True" w641 {
              frame False {
                w643 = FALSE ("Visible")
                # "hide cursors from image graph"
                n144 = property on="Image" class="IntGraph (strict)"("Active Cursor"=u32 0, "Cursor.Visible"=w643) -> ()  [unwired: 2 in, 2 out]
                n145 = property on="Image" class="IntGraph (strict)"("Active Cursor"=u32 1, "Cursor.Visible"=w643) -> ()  [unwired: 2 in, 2 out]
              }
              frame True {
                w645 = TRUE ("Visible")
                n146 = property on="Image" class="IntGraph (strict)"() -> ("XScale.Minimum"=w650:dbl, "YScale.Maximum"=w649:dbl, "XScale.Maximum"=w648:dbl, "YScale.Minimum"=w647:dbl)  [unwired: 2 in, 2 out]
                n147 = property on="Image" class="IntGraph (strict)"("Active Cursor"=u32 0, "Cursor.Visible"=w645, "Cursor.Cursor X"=w650, "Cursor.Cursor Y"=w649) -> ()  [unwired: 2 in, 2 out]
                n148 = property on="Image" class="IntGraph (strict)"("Active Cursor"=u32 1, "Cursor.Visible"=w645, "Cursor.Cursor X"=w648, "Cursor.Cursor Y"=w647) -> ()  [unwired: 2 in, 2 out]
              }
            }
          }
          event "Timelapse?": Value Change {
            n149 = event-data() -> ()  [unwired: 1 in, 1 out]
            n150 = Select(t=T23."Enabled" ("Disabled"), s="Timelapse?", f=T23."Disabled and Grayed Out" ("Disabled")) -> (s? t:f=w652:T23)
            n151 = property on="Timelapse Wait (s)" class="DigNum (strict)"("DisabledEnum"=w652) -> ()  [unwired: 2 in, 2 out]
            n152 = property on="Timelapse Cycles" class="DigNum (strict)"("DisabledEnum"=w652) -> ()  [unwired: 2 in, 2 out]
          }
          event "Camera Ctrl.Autoscale": Value Change {
            n153 = event-data() -> ("NewVal"=w658:bool)  [unwired: 1 in]
            n154 = case shown="False" w658 {
              tunnel: [T23."Enabled" ("Disabled") T23."Disabled and Grayed Out" ("Disabled")] -> w656
              tunnel: [u8 0 ("X Scale.Scale Fit") u8 2 ("X Scale.Scale Fit")] -> w657
              frame False {
                # "autoscale OFF"
                # "initialize scale cursors to\nthe current histogram"
                n155 = property on="Histogram" class="XYGraph (strict)"() -> ("XScale.Minimum"=w663:dbl, "XScale.Maximum"=w659:dbl)  [unwired: 2 in, 2 out]
                n156 = property on="Histogram" class="XYGraph (strict)"("Active Cursor"=u32 0, "Cursor.Visible"=TRUE, "Cursor.Cursor X"=w663, "Cursor.Cursor Y"=-1000.0 ("y")) -> ()  [unwired: 2 in, 2 out]
                n157 = property on="Histogram" class="XYGraph (strict)"("Active Cursor"=u32 1, "Cursor.Visible"=TRUE, "Cursor.Cursor X"=w659, "Cursor.Cursor Y"=-1000.0 ("y")) -> ()  [unwired: 2 in, 2 out]
              }
              frame True {
                w669 = FALSE ("Visible")
                # "autoscale ON"
                # "hide cursors from image graph"
                n158 = property on="Histogram" class="XYGraph (strict)"("Active Cursor"=u32 0, "Cursor.Visible"=w669) -> ()  [unwired: 2 in, 2 out]
                n159 = property on="Histogram" class="XYGraph (strict)"("Active Cursor"=u32 1, "Cursor.Visible"=w669) -> ()  [unwired: 2 in, 2 out]
              }
            }
            n160 = property on="Histogram" class="XYGraph (strict)"("XScale.ScaleFit"=w657) -> ()  [unwired: 2 in, 2 out]
            n161 = property on="Image" class="IntGraph (strict)"("ZScale.ScaleFit"=w657) -> ()  [unwired: 2 in, 2 out]
            n162 = property on="Scale" class="Clust (strict)"("DisabledEnum"=w656) -> ()  [unwired: 2 in, 2 out]
          }
          event "Camera Ctrl.Scale": Value Change {
            n163 = event-data() -> ("NewVal"=w680:cluster{"Scale.Min":i32, "Scale.Max":i32})  [unwired: 1 in]
            n164 = Unbundle By Name(w680) -> ("Scale.Min"=w678:i32, "Scale.Max"=w674:i32)
            n165 = property on="Histogram" class="XYGraph (strict)"("Active Cursor"=u32 0, "Cursor.Visible"=TRUE, "Cursor.Cursor X"=w678) -> ()  [unwired: 2 in, 2 out]
            n166 = property on="Histogram" class="XYGraph (strict)"("Active Cursor"=u32 1, "Cursor.Visible"=TRUE, "Cursor.Cursor X"=w674) -> ()  [unwired: 2 in, 2 out]
            n167 = property on="Image" class="IntGraph (strict)"("ZScale.Minimum"=w678, "ZScale.Maximum"=w674) -> ()  [unwired: 2 in, 2 out]
          }
          event "Cal step num": Value Change {
            n168 = event-data() -> ()  [unwired: 1 in, 1 out]
            n169 = local read "Z-Stack"() -> (w688:T10)
            n170 = Unbundle By Name(w688) -> ("Z end"=w687:dbl, "Z0"=w686:dbl, "Step Size"=w685:dbl)
            n171 = Subtract(x=w687, y=w686) -> (x-y=w689:dbl)
            n172 = Divide(x=w689, y=w685) -> (x/y=w684:dbl)
            n173 = local read "Z-Stack"() -> (w683:T10)
            n174 = Bundle By Name(cluster=w683, "Step Num"=w684) -> (w682:T10)
            n175 = local write "Z-Stack"(w682) -> ()
            n176 = local write "Cal step size"(FALSE) -> ()
          }
          event "Cal step size": Value Change {
            n177 = event-data() -> ()  [unwired: 1 in, 1 out]
            n178 = local read "Z-Stack"() -> (w696:T10)
            n179 = Unbundle By Name(w696) -> ("Z end"=w695:dbl, "Z0"=w694:dbl, "Step Num"=w693:i32)
            n180 = Subtract(x=w695, y=w694) -> (x-y=w698:dbl)
            n181 = Divide(x=w698, y=w693) -> (x/y=w692:dbl)
            n182 = local read "Z-Stack"() -> (w691:T10)
            n183 = Bundle By Name(cluster=w691, "Step Size"=w692) -> (w690:T10)
            n184 = local write "Z-Stack"(w690) -> ()
            n185 = local write "Cal step size"(FALSE) -> ()
          }
          event "# frames": Value Change {
            n186 = event-data() -> ()  [unwired: 1 in, 1 out]
            n187 = local read "Movie frame rate (Hz)"() -> (w699:dbl)
            n188 = Divide(x="# frames", y=w699) -> (x/y=w701:dbl)
            n189 = local write "Total time (sec)"(w701) -> ()
          }
          event "Total time (sec)": Value Change {
            n190 = event-data() -> ()  [unwired: 1 in, 1 out]
            n191 = local read "Movie frame rate (Hz)"() -> (w702:dbl)
            n192 = Multiply(x="Total time (sec)", y=w702) -> (x*y=w704:dbl)
            n193 = Round To Nearest(number=w704) -> (nearest integer value=w703:dbl)
            n194 = Divide(x=w703, y=w702) -> (x/y=w706:dbl)
            n195 = local write "# frames"(w703) -> ()
            n196 = local write "Total time (sec)"(w706) -> ()
          }
          event "Movie frame rate (Hz)": Value Change {
            n197 = event-data() -> ()  [unwired: 1 in, 1 out]
            n198 = local read "# frames"() -> (w709:i32)
            n199 = Divide(x=w709, y="Movie frame rate (Hz)") -> (x/y=w707:dbl)
            n200 = local write "Total time (sec)"(w707) -> ()
          }
          event "Scope on?", "Camera on?", "TI-Ctrl.Obj": Value Change {
            n201 = event-data() -> ()  [unwired: 1 in, 1 out]
            n202 = control-ref of="Pixel size (nm)"() -> (w714:refnum<vi>)
            n203 = control-ref of="Total y width (μm)"() -> (w713:refnum<vi>)
            n204 = control-ref of="scale bar (μm)"() -> (w711:refnum<vi>)
            n205 = control-ref of="Total x width (μm)"() -> (w712:refnum<vi>)
            n206 = local read "TI-Ctrl"() -> (w716:T9)
            n207 = property on="ROI" class="Clust (strict)"() -> ("Value"=w715:T3)  [unwired: 2 in, 2 out]
            n208 = Bundle("Total x width (μm)"=w712, "Total y width (μm)"=w713, "Pixel size (nm)"=w714, "scale bar (μm)"=w711) -> (w710:T28)  [unwired: 1 in]
            n209 = call "subCalculate_SetScaleBar.vi"("ROI in"=w715, "Scale calculation cluster"=w710, "TI-Ctrl"=w716) -> ()  [unwired: 7 in, 2 out]
          }
          event "Generate Tiling": Value Change {
            n210 = event-data() -> ()  [unwired: 1 in, 1 out]
            n211 = case shown="0, Default" "Ranking" {
              frame 0, Default {
                n212 = property on="Record Table" class="Tbl (strict)"() -> (error out=w718:errorcluster, "Value"=w721:string[][])  [unwired: 2 in, 1 out]
                n213 = property on="XY Scan List" class="Tbl (strict)"(error in=w718, "Value"=w721) -> (error out=w719:errorcluster)  [unwired: 1 in, 1 out]
                n214 = property on="Generate Tiling" class="Bool (strict)"(error in=w719, "Value"=FALSE ("Generate Tiling")) -> ()  [unwired: 1 in, 2 out]
              }
              frame 1 {
                n215 = local read "XY Scan List"() -> (w725:string[][])
                n216 = call "subStage_GetMinimumMovingDistance.vi"("XY Scan List"=w725) -> ("error out"=w723:errorcluster, "XY Scan List (reorder)"=w724:string[][])  [unwired: 9 in]
                n217 = local write "XY Scan List"(w724) -> ()
                n218 = property on="Generate Tiling" class="Bool (strict)"(error in=w723, "Value"=FALSE ("Generate Tiling")) -> ()  [unwired: 1 in, 2 out]
              }
              frame 2 {
                n219 = local write "XY Scan List"(string[][] [] ("XY Scan List")) -> ()
                n220 = property on="Generate Tiling" class="Bool (strict)"("Value"=FALSE ("Generate Tiling")) -> ()  [unwired: 2 in, 2 out]
              }
            }
          }
        }
        n221 = local read "stop program"() -> (w628:bool)
      }
      n222 = while {
        stop <- w50 stop-if-true
        # "Patch tuning"
        n223 = event shown="[2] \"Save patch param\": Value Change" {
          selector: _ -> [_ _ _]
          dyn-events: _ -> [_ _ _]
          timeout: 50 -> [_ _ _]
          event Timeout {
            n224 = event-data() -> ()  [unwired: 1 in, 1 out]
          }
          event "Test patch": Value Change {
            n225 = event-data() -> ()  [unwired: 1 in, 1 out]
            n226 = property on="DAQ ports" class="Clust (strict)"() -> ("Value"=w52:T25)  [unwired: 2 in, 2 out]
            n227 = call "subAxopatch_PatchParams.vi"("DAQ ports"=w52, "Pipet tuning parameters"="Pipet tuning parameters") -> ("Error out"=w58:errorcluster, "Average I-t curve"=→"Average I-t curve":cluster{"xo":i32, dbl, dbl[]}, "Patch output"=→"Patch output":cluster{"xo":i32, dbl, "data":dbl[][]}, "Patch quality"=→"Patch quality":T29, "Seal test DAQ params"=→"Seal test DAQ params":T15, "Patch seal test waveform"=→"Patch seal test waveform":waveform(dbl))  [unwired: 4 in]
            n228 = case shown="No Error" w58 {
              frame No Error {
                n229 = local write "Test patch"(FALSE ("Test patch")) -> ()
              }
              frame Error {
              }
            }
          }
          event "Save patch param": Value Change {
            n230 = event-data() -> ()  [unwired: 1 in, 1 out]
            n231 = flat-sequence {
              frame #0 {
                n232 = local read "Patch output"() -> (w61:cluster{"xo":i32, dbl, "data":dbl[][]})
                n233 = local read "Base folder"() -> (w63:path)
                n234 = local read "Patch quality"() -> (w62:T17)
                n235 = call "subSave_PatchParams_New.vi"("Scaled output"=w61, "Patch quality"=w62, "Base path"=w63) -> ()  [unwired: 9 in]
              }
              frame #1 {
                n236 = local write "Save patch param"(FALSE ("Save patch param")) -> ()
              }
            }
          }
        }
        n237 = local read "stop program"() -> (w50:bool)
      }
      n238 = while {
        shift-right: [w65] -> _
        shift-left: T22 {"width"=0, "height"=0, "datatype"=0} ("Buffer") -> [w69]
        shift-right: [w68] -> w36
        shift-left: errorcluster {"status"=FALSE, "code"=0, "source"=""} ("camera \ninitialization\nerror") -> [w67]
        stop <- "stop program" stop-if-true
        # "Camera"
        n239 = event shown="[2] \"Camera on?\": Value Change" {
          selector: _ -> [_ _ _ _ _ _ _ _ _ _ _ _]
          dyn-events: _ -> [_ _ _ _ _ _ _ _ _ _ _ _]
          timeout: 50 -> [_ _ _ _ _ _ _ _ _ _ _ _]
          tunnel: w69 -> [w77 w88 _ _ _ _ _ _ w386 _ _ _]
          tunnel: w67 -> [w76 w91 w158 w228 w259 w308 w351 w381 w387 w402 w468 w526]
          tunnel: [w75 w90 w159 w227 w258 w307 w350 w380 w389 w401 w463 w525] -> w68
          tunnel: [w71 w89 _ w223 w240 w302 w344 w376 w386 w399 w461 w524] -> w65
          event Timeout {
            n240 = event-data() -> ()  [unwired: 1 in, 1 out]
            n241 = local read "Camera on?"() -> (w74:bool)
            n242 = property on="Live" class="Bool (strict)"() -> ("Value"=w72:bool)  [unwired: 2 in, 2 out]
            n243 = And(x=w74, y=w72) -> (x .and. y?=w73:bool)
            n244 = case shown="True" w73 {
              tunnel: w76 -> [w79 w84]
              tunnel: [w79 w86] -> w75
              tunnel: w77 -> [w78 w85]
              tunnel: [w78 w85] -> w71
              frame False {
              }
              frame True {
                n245 = property on="Handle" class="DigNum (strict)"() -> ("Value"=w83:u32)  [unwired: 2 in, 2 out]
                n246 = property on="ROI" class="Clust (strict)"() -> ("Value"=w82:T3)  [unwired: 2 in, 2 out]
                n247 = call "subHamamatsu_UpdateImageInfo.vi"("ROI"=w82, "Error In"=w84, "Image Buffer"=w85, "Handle in"=w83) -> ("Error out"=w86:errorcluster, "Histogram"=w80:T30, "Image out"=w81:u16[][])  [unwired: 5 in]
                n248 = property on="Image" class="IntGraph (strict)"("Value"=w81) -> ()  [unwired: 2 in, 2 out]
                n249 = property on="Histogram" class="Clust (strict)"("Value"=w80) -> ()  [unwired: 2 in, 2 out]
              }
            }
          }
          event "Camera Ctrl.Chosen Camera": Value Change {
            # "Disable and grey out Camera Chosen"
            n250 = event-data() -> ("NewVal"=w87:u32)  [unwired: 1 in]
            n251 = case shown="0, Default" w87 {
              tunnel: w91 -> [w98 w128]
              tunnel: [w97 w129] -> w90
              tunnel: [w95 w127] -> w89
              tunnel: w88 -> [w96 w130]
              frame 0, Default {
                # "Left camera initialized?"
                n252 = local read "Camera initialized"() -> (w93:bool[])
                n253 = Index Array(array=w93, index=0) -> (element=w92:bool)
                n254 = case shown="True" w92 {
                  tunnel: w98 -> [w103 w116]
                  tunnel: [w103 w107] -> w97
                  tunnel: w96 -> [w99 _]
                  tunnel: [w99 w106] -> w95
                  frame False {
                    n255 = One Button Dialog(message="Please turn on the Left camera first!", button name ("OK")="OK") -> ()  [unwired: 1 out]
                    n256 = property on="Chosen Camera" class="Ring (strict)"("Value"=u32 1) -> ()  [unwired: 2 in, 2 out]
                  }
                  frame True {
                    # "open and set new camera"
                    # "Chosen camera = 0 --> left camera\nTurn of Global shutter to block epi-illumination"
                    n257 = local read "Light control"() -> (w122:T1)
                    n258 = property on="DAQ ports" class="Clust (strict)"() -> ("Value"=w105:T25)  [unwired: 2 in, 2 out]
                    n259 = Bundle By Name(cluster=w122, "Global"=FALSE ("new element/subarray")) -> (w121:T1)
                    n260 = call "subDAQ_SetGlobal.vi"("DAQ ports"=w105, "Light control (All off)"=w121) -> ()  [unwired: 9 in, 1 out]
                    n261 = local write "Light control"(w121) -> ()
                    n262 = property on="Handle" class="DigNum (strict)"() -> ("Value"=w114:u32)  [unwired: 2 in, 2 out]
                    n263 = call "subHamamatsu_CloseCam.vi"("Live"=TRUE, "error in (no error)"=w116, "Handle in"=w114) -> ("error out"=w117:errorcluster)  [unwired: 8 in]
                    n264 = property on="ROI" class="Clust (strict)"() -> ("Value"=w118:T3)  [unwired: 2 in, 2 out]
                    n265 = property on="Exposure (ms)" class="DigNum (strict)"() -> ("Value"=w119:dbl)  [unwired: 2 in, 2 out]
                    n266 = property on="Chosen Camera" class="Ring (strict)"() -> ("Value"=w115:u32)  [unwired: 2 in, 2 out]
                    n267 = property on="Camera Setting" class="Clust (strict)"() -> ("Value"=w104:T31)  [unwired: 2 in, 2 out]
                    n268 = call "subHamamatsu_OpenCam.vi"("Exposure (ms)"=w119, "ROI"=w118, "error in (no error)"=w117, "Camera Setting"=w104, "Handle in"=w115) -> ("error out"=w112:errorcluster, "Camera in use"=w120:T32, "Handle out"=w111:u32)  [unwired: 4 in]
                    n269 = property on="Camera in use" class="Clust (strict)"("Value"=w120) -> ()  [unwired: 2 in, 2 out]
                    n270 = property on="Live" class="Bool (strict)"() -> ("Value"=w109:bool)  [unwired: 2 in, 2 out]
                    n271 = call "subHamamatsu_TurnOnOff.vi"("logic 2"=TRUE ("logic 1"), "logic 1"=w109, "error in (no error)"=w112, "Handle in"=w111) -> ("error out"=w107:errorcluster, "Buffer"=w106:T22, "Handle out"=w110:u32)  [unwired: 5 in]
                    n272 = property on="Handle" class="DigNum (strict)"("Value"=w110) -> ()  [unwired: 2 in, 2 out]
                  }
                }
              }
              frame 1 {
                # "Right camera intialized?"
                # "handle 0 = left (S/N: 003222)\nhandle 1 = right (S/N: 003223)"
                n273 = local read "Camera initialized"() -> (w125:bool[])
                n274 = Index Array(array=w125, index=1) -> (element=w124:bool)
                n275 = case shown="True" w124 {
                  tunnel: w128 -> [w135 w147]
                  tunnel: [w135 w143] -> w129
                  tunnel: w130 -> [w131 _]
                  tunnel: [w131 w139] -> w127
                  frame False {
                    n276 = One Button Dialog(message="Please turn on the Right camera first!", button name ("OK")="OK") -> ()  [unwired: 1 out]
                    n277 = property on="Chosen Camera" class="Ring (strict)"("Value"=u32 0) -> ()  [unwired: 2 in, 2 out]
                  }
                  frame True {
                    # "open and set new camera"
                    n278 = property on="Handle" class="DigNum (strict)"() -> ("Value"=w145:u32)  [unwired: 2 in, 2 out]
                    n279 = call "subHamamatsu_CloseCam.vi"("Live"=TRUE, "error in (no error)"=w147, "Handle in"=w145) -> ("error out"=w148:errorcluster)  [unwired: 8 in]
                    n280 = property on="Chosen Camera" class="Ring (strict)"() -> ("Value"=w146:u32)  [unwired: 2 in, 2 out]
                    n281 = property on="Camera Setting" class="Clust (strict)"() -> ("Value"=w136:T31)  [unwired: 2 in, 2 out]
                    n282 = property on="ROI" class="Clust (strict)"() -> ("Value"=w149:T3)  [unwired: 2 in, 2 out]
                    n283 = property on="Exposure (ms)" class="DigNum (strict)"() -> ("Value"=w150:dbl)  [unwired: 2 in, 2 out]
                    n284 = call "subHamamatsu_OpenCam.vi"("Exposure (ms)"=w150, "ROI"=w149, "error in (no error)"=w148, "Camera Setting"=w136, "Handle in"=w146) -> ("error out"=w142:errorcluster, "Camera in use"=w151:T32, "Handle out"=w138:u32)  [unwired: 4 in]
                    n285 = property on="Camera in use" class="Clust (strict)"("Value"=w151) -> ()  [unwired: 2 in, 2 out]
                    n286 = property on="Live" class="Bool (strict)"() -> ("Value"=w141:bool)  [unwired: 2 in, 2 out]
                    n287 = call "subHamamatsu_TurnOnOff.vi"("logic 2"=TRUE ("logic 1"), "logic 1"=w141, "error in (no error)"=w142, "Handle in"=w138) -> ("error out"=w143:errorcluster, "Buffer"=w139:T22, "Handle out"=w137:u32)  [unwired: 5 in]
                    n288 = property on="Handle" class="DigNum (strict)"("Value"=w137) -> ()  [unwired: 2 in, 2 out]
                  }
                }
              }
            }
          }
          event "Camera on?": Value Change {
            n289 = event-data() -> ("NewVal"=w152:bool)  [unwired: 1 in]
            n290 = case shown="True" w152 {
              tunnel: [w171 w181] -> w159
              tunnel: w158 -> [w170 w177]
              tunnel: [FALSE FALSE] -> w155
              tunnel: [bool[] [FALSE, FALSE] ("Camera initialized") w175] -> w157
              tunnel: [T23."Disabled and Grayed Out" ("Disabled") w176] -> w156
              tunnel: ["Ready" ("Status") w173] -> w154
              tunnel: [u32 0 ("Handle out") w172] -> w153
              frame False {
                # "First, stop live capture.  Then deinitialize camera."
                n291 = property on="Handle" class="DigNum (strict)"() -> ("Value"=w163:u32)  [unwired: 2 in, 2 out]
                n292 = property on="Live" class="Bool (strict)"() -> ("Value"=w164:bool)  [unwired: 2 in, 2 out]
                n293 = call "subHamamatsu_TurnOnOff.vi"("logic 2"=FALSE, "logic 1"=w164, "error in (no error)"=w170, "Handle in"=w163) -> ("error out"=w169:errorcluster, "Handle out"=w162:u32)  [unwired: 5 in, 1 out]
                n294 = call "subHamamatsu_Deinitialization.vi"("error in (no error)"=w169, "Handle"=w162) -> ("error out"=w171:errorcluster)  [unwired: 9 in]
              }
              frame True {
                # "If no camera is initialized, report error.\nIf only 1 camera is initialized, use that one.\nIf both cameras are initialized, choose camera."
                n295 = flat-sequence {
                  tunnel: [w186] -> w179
                  tunnel: [w191] -> w178
                  tunnel: w177 -> [w190]
                  tunnel: [w188] -> w175
                  tunnel: [w189] -> w174
                  frame #0 {
                    n296 = local read "Camera Ctrl"() -> (w185:T8)
                    n297 = property on="Camera Setting" class="Clust (strict)"() -> ("Value"=w182:T31)  [unwired: 2 in, 2 out]
                    n298 = property on="Status" class="Str"("Value"="Initializing Camera ..." ("Status")) -> ()  [unwired: 2 in, 2 out]
                    n299 = call "subHamamatsu_Initialization.vi"("Camera Ctrl"=w185, "error in (no error)"=w190, "Camera Setting"=w182) -> ("error out"=w191:errorcluster, "Chosen Camera"=w183:u32, "Handle out"=w186:u32, "Camera Info"=w184:T19, "Number Of Cameras"=w189:u32, "Camera initialized"=w188:bool[])  [unwired: 3 in]
                    n300 = local write "Camera Info"(w184) -> ()
                    n301 = property on="Chosen Camera" class="Ring (strict)"("Value"=w183) -> ()  [unwired: 2 in, 2 out]
                  }
                }
                n302 = case shown="1, 2" w174 {
                  tunnel: w178 -> [w196 w219]
                  tunnel: w179 -> [w193 w217]
                  tunnel: [w196 w199] -> w181
                  tunnel: [T23."Disabled and Grayed Out" ("Disabled") T23."Enabled" ("Disabled")] -> w176
                  tunnel: [w193 w197] -> w172
                  tunnel: ["Camera not detected." ("Status") "Ready" ("Status")] -> w173
                  frame 0, Default {
                    n303 = property on="Camera on?" class="Bool (strict)"("Value"=FALSE ("Camera on?")) -> ()  [unwired: 2 in, 2 out]
                  }
                  frame 1, 2 {
                    # "initialize image"
                    n304 = control-ref of="Camera View indicator"() -> (w210:refnum<vi>)
                    n305 = control-ref of="Image"() -> (w211:refnum<vi>)
                    n306 = call "subImage_InitializeImage.vi"("error in (no error)"=w219, "Handle in"=w217) -> ("error out"=w218:errorcluster, "Handle out"=w216:u32)  [unwired: 7 in, 1 out]
                    n307 = property on="ROI" class="Clust (strict)"() -> ("Value"=w213:T3)  [unwired: 2 in, 2 out]
                    n308 = call "subHamamatsu_SetROI.vi"("ROI"=w213, "error in (no error)"=w218, "Handle in"=w216) -> ("error out"=w203:errorcluster, "Handle out"=w204:u32)  [unwired: 6 in, 1 out]
                    n309 = property on="Autoscale" class="Bool (strict)"("Value"=TRUE ("Autoscale")) -> ()  [unwired: 2 in, 2 out]
                    n310 = call "subImage_UpdateLocIndicator.vi"("Camera View Indicator Ref"=w210, "Image Refnum"=w211, "ROI"=w213, "error in"=w203, "Handle in"=w204) -> ("error out"=w202:errorcluster, "Handle out"=w201:u32)  [unwired: 5 in]
                    n311 = control-ref of="Pixel size (nm)"() -> (w208:refnum<vi>)
                    n312 = control-ref of="Total y width (μm)"() -> (w207:refnum<vi>)
                    n313 = control-ref of="scale bar (μm)"() -> (w209:refnum<vi>)
                    n314 = control-ref of="Total x width (μm)"() -> (w206:refnum<vi>)
                    n315 = local read "TI-Ctrl"() -> (w214:T9)
                    n316 = Bundle("Total x width (μm)"=w206, "Total y width (μm)"=w207, "Pixel size (nm)"=w208, "scale bar (μm)"=w209) -> (w205:T28)  [unwired: 1 in]
                    n317 = call "subCalculate_SetScaleBar.vi"("ROI in"=w213, "Scale calculation cluster"=w205, "TI-Ctrl"=w214, "error in"=w202, "Handle in"=w201) -> ("error out"=w200:errorcluster, "Handle out"=w198:u32)  [unwired: 5 in]
                    n318 = call "subHamamatsu_GetMaxFrameRate.vi"("ROI in"=w213, "error in"=w200, "Handle in"=w198) -> ("error out"=w199:errorcluster, "Handle out"=w197:u32, "max frame rate (Hz)"=w215:dbl)  [unwired: 6 in]
                    n319 = property on="max frame rate (Hz)" class="DigNum (strict)"("Value"=w215) -> ()  [unwired: 2 in, 2 out]
                  }
                }
              }
            }
            "Camera initialized" <- w157
            n320 = property on="Live" class="Bool (strict)"("Value"=w155) -> ()  [unwired: 2 in, 2 out]
            n321 = property on="Camera Ctrl" class="Clust (strict)"("DisabledEnum"=w156) -> ()  [unwired: 2 in, 2 out]
            n322 = property on="Status" class="Str"("Value"=w154) -> ()  [unwired: 2 in, 2 out]
            n323 = property on="Handle" class="DigNum (strict)"("Value"=w153) -> ()  [unwired: 2 in, 2 out]
          }
          event "Camera Ctrl.Live": Value Change {
            n324 = event-data() -> ()  [unwired: 1 in, 1 out]
            n325 = property on="Handle" class="DigNum (strict)"() -> ("Value"=w222:u32)  [unwired: 2 in, 2 out]
            n326 = property on="Live" class="Bool (strict)"() -> ("Value"=w225:bool)  [unwired: 2 in, 2 out]
            n327 = call "subHamamatsu_TurnOnOff.vi"("logic 2"=w225, "logic 1"=TRUE ("Status pre"), "error in (no error)"=w228, "Handle in"=w222) -> ("error out"=w227:errorcluster, "Buffer"=w223:T22)  [unwired: 5 in, 1 out]
            n328 = case shown="False" w225 {
              tunnel: ["Ready" ("Status") "Camera live" ("Status")] -> w224
              frame False {
              }
              frame True {
              }
            }
            n329 = property on="Status" class="Str"("Value"=w224) -> ()  [unwired: 2 in, 2 out]
          }
          event "Camera Ctrl.Snap": Value Change {
            w257 = TRUE ("Snap&Save")
            # "Resume camera"
            # "Turn off camera"
            n330 = event-data() -> ()  [unwired: 1 in, 1 out]
            n331 = property on="Live" class="Bool (strict)"() -> ("Value"=w252:bool)  [unwired: 2 in, 2 out]
            n332 = property on="Handle" class="DigNum (strict)"() -> ("Value"=w239:u32)  [unwired: 2 in, 2 out]
            n333 = call "subHamamatsu_TurnOnOff.vi"("logic 2"=FALSE, "logic 1"=w252, "error in (no error)"=w259, "Handle in"=w239) -> ("error out"=w261:errorcluster, "Handle out"=w238:u32)  [unwired: 5 in, 1 out]
            n334 = call "subHamamatsu_Snapshot.vi"("Error in"=w261, "Value"=w238) -> ("Error out"=w251:errorcluster, "Image"=w237:u16[][], "Handle out"=w255:u32)  [unwired: 7 in]
            n335 = property on="ROI" class="Clust (strict)"() -> ("Value"=w236:T3)  [unwired: 2 in, 2 out]
            n336 = local read "Camera Ctrl"() -> (w231:T8)
            n337 = call "subImage_Pad.vi"("ROI"=w236, "Image in"=w237) -> ("Image out"=w235:u16[][])  [unwired: 7 in, 2 out]
            n338 = property on="DAQ ports" class="Clust (strict)"() -> ("Value"=w234:T25)  [unwired: 2 in, 2 out]
            n339 = property on="Image" class="IntGraph (strict)"("Value"=w235) -> ()  [unwired: 2 in, 2 out]
            n340 = local read "Camera Info"() -> (w232:T19)
            n341 = local read "Base folder"() -> (w264:path)
            n342 = local read "Image Info"() -> (w245:T2)
            n343 = local read "Confocal scanner"() -> (w247:T5)
            n344 = local read "TI-Ctrl"() -> (w244:T9)
            n345 = call "subDAQ_SetLaserDO.vi"("DAQ ports"=w234, "Error in (no error)"=w251) -> ("Error out"=w254:errorcluster)  [unwired: 9 in]
            n346 = call <vilib>:"Check if File or Folder Exists.vi"("path"=w264) -> ("file or folder exists?"=w263:bool, "dup path"=w262:path)  [unwired: 8 in, 1 out]
            n347 = local read "Stage Status"() -> (w246:T7)
            n348 = local read "Light control"() -> (w248:T1)
            n349 = case shown="True" w263 {
              tunnel: w262 -> [w276 w277]
              tunnel: [w275 w277] -> w256
              frame False {
                n350 = Create Folder(path (use dialog)=w276) -> (created path=w275:path)  [unwired: 2 in, 2 out]
              }
              frame True {
              }
            }
            n351 = call "subAcquisition_Info.vi"("Stage Status"=w246, "Light control"=w248, "Image Info"=w245, "Confocal scanner"=w247, "TI-Ctrl"=w244, "Camera Info"=w232, "Camera Ctrl"=w231) -> ("Text"=w249:string)  [unwired: 4 in]
            n352 = call "subSave_Img2Tiff.vi"("Open file dialog? (F)"=w257, "Save Text file? (F)"=w257, "Error in (no error)"=w254, "text"=w249, "Image"=w237, "File path/name"=w256) -> ("Error out"=w243:errorcluster, "Cancel or not?"=w233:bool)  [unwired: 4 in]
            n353 = local read "Light control"() -> (w253:T1)
            n354 = property on="Snap" class="Bool (strict)"(error in=w243, "Value"=FALSE ("Snap&Save")) -> (error out=w242:errorcluster)  [unwired: 1 in, 1 out]
            n355 = case shown="False" w233 {
              frame False {
                n356 = control-ref of="Snap Point  Y Array"() -> (w267:refnum<vi>)
                n357 = control-ref of="Snap Point  X Array"() -> (w268:refnum<vi>)
                n358 = control-ref of="Snap Number Counting"() -> (w269:refnum<vi>)
                n359 = control-ref of="Record Table"() -> (w266:refnum<vi>)
                n360 = property on="Stage Status" class="Clust (strict)"() -> ("Value"=w274:T7)  [unwired: 2 in, 2 out]
                n361 = call "subDAQ_GetSnapPoint.vi"("Record Table Refnum"=w266, "Snap Number Refnum"=w269, "Snap Point Y Arr Refnum"=w267, "Snap Point X Arr Refnum"=w268, "Snap Number Counting"="Snap Number Counting", "Stage Status"=w274) -> ("Snap Point cluster"=→"Snap Point cluster":cluster{"Snap Y":dbl[], "Snap X":dbl[]}, "Snap Point  Y Array"=→"Snap Point  Y Array":dbl[], "Snap Point  X Array"=→"Snap Point  X Array":dbl[])  [unwired: 3 in]
              }
              frame True {
              }
            }
            n362 = call "subDAQ_SetLaserDO.vi"("DAQ ports"=w234, "Light control (All off)"=w253, "Error in (no error)"=w242) -> ()  [unwired: 8 in, 1 out]
            n363 = property on="Live" class="Bool (strict)"() -> ("Value"=w250:bool)  [unwired: 2 in, 2 out]
            n364 = call "subHamamatsu_TurnOnOff.vi"("logic 2"=TRUE, "logic 1"=w250, "error in (no error)"=w251, "Handle in"=w255) -> ("error out"=w258:errorcluster, "Buffer"=w240:T22)  [unwired: 5 in, 1 out]
          }
          event "Camera Ctrl.ROI update": Value Change {
            n365 = event-data() -> ()  [unwired: 1 in, 1 out]
            n366 = property on="Handle" class="DigNum (strict)"() -> ("Value"=w300:u32)  [unwired: 2 in, 2 out]
            n367 = property on="Live" class="Bool (strict)"() -> ("Value"=w304:bool)  [unwired: 2 in, 2 out]
            n368 = call "subHamamatsu_TurnOnOff.vi"("logic 2"=FALSE ("Status post"), "logic 1"=w304, "error in (no error)"=w308, "Handle in"=w300) -> ("error out"=w305:errorcluster, "Handle out"=w306:u32)  [unwired: 5 in, 1 out]
            n369 = property on="ROI define" class="Bool (strict)"() -> ("Value"=w299:bool)  [unwired: 2 in, 2 out]
            n370 = property on="ROI cursor" class="Clust (strict)"() -> ("Value"=w301:T3)  [unwired: 2 in, 2 out]
            n371 = property on="ROI" class="Clust (strict)"() -> ("Value"=w296:T3)  [unwired: 2 in, 2 out]
            n372 = property on="ROI selection" class="Ring (strict)"() -> ("Value"=w298:u16)  [unwired: 2 in, 2 out]
            n373 = call "subHamamatsu_DefineROI.vi"("ROI selection"=w298, "ROI define"=w299, "ROI cursor"=w301) -> ("ROI out"=w297:T3)  [unwired: 8 in]
            n374 = call "subCalculate_SwitchROI.vi"("ROI 2 in"=w296, "ROI 1 in"=w297) -> ("ROI 2 out"=w294:T3, "ROI 1 out"=w295:T3)  [unwired: 8 in]
            n375 = call "subHamamatsu_SetROI.vi"("ROI"=w294, "error in (no error)"=w305, "Handle in"=w306) -> ("error out"=w284:errorcluster, "Handle out"=w285:u32)  [unwired: 6 in, 1 out]
            n376 = control-ref of="Camera View indicator"() -> (w291:refnum<vi>)
            n377 = control-ref of="Image"() -> (w292:refnum<vi>)
            n378 = property on="Previous ROI" class="Clust (strict)"("Value"=w295) -> ()  [unwired: 2 in, 2 out]
            n379 = call "subImage_UpdateLocIndicator.vi"("Camera View Indicator Ref"=w291, "Image Refnum"=w292, "ROI"=w294, "error in"=w284, "Handle in"=w285) -> ("error out"=w282:errorcluster, "Handle out"=w283:u32)  [unwired: 5 in]
            n380 = control-ref of="Pixel size (nm)"() -> (w289:refnum<vi>)
            n381 = control-ref of="Total y width (μm)"() -> (w288:refnum<vi>)
            n382 = control-ref of="scale bar (μm)"() -> (w290:refnum<vi>)
            n383 = control-ref of="Total x width (μm)"() -> (w287:refnum<vi>)
            n384 = local read "TI-Ctrl"() -> (w293:T9)
            n385 = Bundle("Total x width (μm)"=w287, "Total y width (μm)"=w288, "Pixel size (nm)"=w289, "scale bar (μm)"=w290) -> (w286:T28)  [unwired: 1 in]
            n386 = call "subCalculate_SetScaleBar.vi"("ROI in"=w294, "Scale calculation cluster"=w286, "TI-Ctrl"=w293, "error in"=w282, "Handle in"=w283) -> ("error out"=w280:errorcluster, "Handle out"=w281:u32)  [unwired: 5 in]
            n387 = call "subHamamatsu_GetMaxFrameRate.vi"("ROI in"=w294, "error in"=w280, "Handle in"=w281) -> ("error out"=w278:errorcluster, "Handle out"=w279:u32, "max frame rate (Hz)"=w303:dbl)  [unwired: 6 in]
            n388 = property on="max frame rate (Hz)" class="DigNum (strict)"("Value"=w303) -> ()  [unwired: 2 in, 2 out]
            n389 = property on="ROI" class="Clust (strict)"("Value"=w294) -> ()  [unwired: 2 in, 2 out]
            n390 = flat-sequence {
              tunnel: w279 -> [w318]
              tunnel: w278 -> [w317]
              tunnel: [w316] -> w302
              tunnel: [w314] -> w307
              frame #0 {
                w311 = FALSE ("Visible")
                n391 = property on="Live" class="Bool (strict)"() -> ("Value"=w310:bool)  [unwired: 2 in, 2 out]
                n392 = property on="ROI update" class="Bool (strict)"("Value"=w311) -> ()  [unwired: 2 in, 2 out]
                n393 = property on="ROI define" class="Bool (strict)"("Value"=w311) -> ()  [unwired: 2 in, 2 out]
                n394 = call "subHamamatsu_TurnOnOff.vi"("logic 2"=TRUE, "logic 1"=w310, "error in (no error)"=w317, "Handle in"=w318) -> ("error out"=w314:errorcluster, "Buffer"=w316:T22)  [unwired: 5 in, 1 out]
                n395 = property on="Image" class="IntGraph (strict)"("Active Cursor"=u32 0, "Cursor.Visible"=w311) -> ()  [unwired: 2 in, 2 out]
                n396 = property on="Image" class="IntGraph (strict)"("Active Cursor"=u32 1, "Cursor.Visible"=w311) -> ()  [unwired: 2 in, 2 out]
              }
            }
          }
          event "Camera Ctrl.ROI previous": Value Change {
            w347 = FALSE ("Update ROI")
            n397 = event-data() -> ()  [unwired: 1 in, 1 out]
            n398 = property on="Handle" class="DigNum (strict)"() -> ("Value"=w342:u32)  [unwired: 2 in, 2 out]
            n399 = property on="ROI previous" class="Bool (strict)"("Value"=w347) -> ()  [unwired: 2 in, 2 out]
            n400 = property on="ROI define" class="Bool (strict)"("Value"=w347) -> ()  [unwired: 2 in, 2 out]
            n401 = property on="Image" class="IntGraph (strict)"("Active Cursor"=u32 0, "Cursor.Visible"=w347) -> ()  [unwired: 2 in, 2 out]
            n402 = property on="Image" class="IntGraph (strict)"("Active Cursor"=u32 1, "Cursor.Visible"=w347) -> ()  [unwired: 2 in, 2 out]
            n403 = property on="Live" class="Bool (strict)"() -> ("Value"=w345:bool)  [unwired: 2 in, 2 out]
            n404 = call "subHamamatsu_TurnOnOff.vi"("logic 2"=FALSE, "logic 1"=w345, "error in (no error)"=w351, "Handle in"=w342) -> ("error out"=w336:errorcluster, "Handle out"=w335:u32)  [unwired: 5 in, 1 out]
            n405 = local read "Previous ROI"() -> (w340:T3)
            n406 = property on="ROI" class="Clust (strict)"() -> ("Value"=w341:T3)  [unwired: 2 in, 2 out]
            n407 = call "subCalculate_SwitchROI.vi"("ROI 2 in"=w341, "ROI 1 in"=w340) -> ("ROI 2 out"=w334:T3, "ROI 1 out"=w339:T3)  [unwired: 8 in]
            n408 = call "subHamamatsu_SetROI.vi"("ROI"=w334, "error in (no error)"=w336, "Handle in"=w335) -> ("error out"=w326:errorcluster, "Handle out"=w322:u32)  [unwired: 6 in, 1 out]
            n409 = control-ref of="Camera View indicator"() -> (w333:refnum<vi>)
            n410 = control-ref of="Image"() -> (w332:refnum<vi>)
            n411 = property on="Previous ROI" class="Clust (strict)"("Value"=w339) -> ()  [unwired: 2 in, 2 out]
            n412 = call "subImage_UpdateLocIndicator.vi"("Camera View Indicator Ref"=w333, "Image Refnum"=w332, "ROI"=w334, "error in"=w326, "Handle in"=w322) -> ("error out"=w325:errorcluster, "Handle out"=w321:u32)  [unwired: 5 in]
            n413 = control-ref of="Pixel size (nm)"() -> (w327:refnum<vi>)
            n414 = control-ref of="Total x width (μm)"() -> (w329:refnum<vi>)
            n415 = control-ref of="Total y width (μm)"() -> (w330:refnum<vi>)
            n416 = control-ref of="scale bar (μm)"() -> (w331:refnum<vi>)
            n417 = local read "TI-Ctrl"() -> (w337:T9)
            n418 = Bundle("Total x width (μm)"=w329, "Total y width (μm)"=w330, "Pixel size (nm)"=w327, "scale bar (μm)"=w331) -> (w328:T28)  [unwired: 1 in]
            n419 = call "subCalculate_SetScaleBar.vi"("ROI in"=w334, "Scale calculation cluster"=w328, "TI-Ctrl"=w337, "error in"=w325, "Handle in"=w321) -> ("error out"=w324:errorcluster, "Handle out"=w320:u32)  [unwired: 5 in]
            n420 = call "subHamamatsu_GetMaxFrameRate.vi"("ROI in"=w334, "error in"=w324, "Handle in"=w320) -> ("error out"=w323:errorcluster, "Handle out"=w319:u32, "max frame rate (Hz)"=w338:dbl)  [unwired: 6 in]
            n421 = property on="max frame rate (Hz)" class="DigNum (strict)"("Value"=w338) -> ()  [unwired: 2 in, 2 out]
            n422 = property on="ROI" class="Clust (strict)"("Value"=w334) -> ()  [unwired: 2 in, 2 out]
            n423 = property on="Live" class="Bool (strict)"() -> ("Value"=w346:bool)  [unwired: 2 in, 2 out]
            n424 = call "subHamamatsu_TurnOnOff.vi"("logic 2"=TRUE, "logic 1"=w346, "error in (no error)"=w323, "Handle in"=w319) -> ("error out"=w350:errorcluster, "Buffer"=w344:T22)  [unwired: 5 in, 1 out]
          }
          event "Camera Ctrl.ROI.Bin": Value Change {
            # "Recalculate ROI"
            n425 = event-data() -> ("OldVal"=w384:u16, "NewVal"=w379:u16)  [unwired: 1 in]
            n426 = property on="Handle" class="DigNum (strict)"() -> ("Value"=w375:u32)  [unwired: 2 in, 2 out]
            n427 = control-ref of="Image"() -> (w373:refnum<vi>)
            n428 = property on="ROI" class="Clust (strict)"() -> ("Value"=w374:T3)  [unwired: 2 in, 2 out]
            n429 = property on="Live" class="Bool (strict)"() -> ("Value"=w378:bool)  [unwired: 2 in, 2 out]
            n430 = call "subHamamatsu_TurnOnOff.vi"("logic 2"=FALSE ("Status post"), "logic 1"=w378, "error in (no error)"=w381, "Handle in"=w375) -> ("error out"=w361:errorcluster, "Handle out"=w363:u32)  [unwired: 5 in, 1 out]
            n431 = call "subImage_UpdateBin.vi"("Bin (n x n)"=w379, "Previous bin"=w384, "Image Refnum"=w373, "ROI in"=w374) -> ("ROI out"=w362:T3)  [unwired: 7 in]
            n432 = call "subHamamatsu_SetBin.vi"("ROI"=w362, "error in (no error)"=w361, "Handle in"=w363) -> ("error out"=w360:errorcluster, "Handle out"=w355:u32)  [unwired: 7 in]
            n433 = control-ref of="Camera View indicator"() -> (w369:refnum<vi>)
            n434 = control-ref of="Image"() -> (w370:refnum<vi>)
            n435 = call "subImage_UpdateLocIndicator.vi"("Camera View Indicator Ref"=w369, "Image Refnum"=w370, "ROI"=w362, "error in"=w360, "Handle in"=w355) -> ("error out"=w359:errorcluster, "Handle out"=w354:u32)  [unwired: 5 in]
            n436 = control-ref of="Total x width (μm)"() -> (w366:refnum<vi>)
            n437 = control-ref of="Total y width (μm)"() -> (w367:refnum<vi>)
            n438 = control-ref of="scale bar (μm)"() -> (w365:refnum<vi>)
            n439 = control-ref of="Pixel size (nm)"() -> (w368:refnum<vi>)
            n440 = local read "TI-Ctrl"() -> (w371:T9)
            n441 = Bundle("Total x width (μm)"=w366, "Total y width (μm)"=w367, "Pixel size (nm)"=w368, "scale bar (μm)"=w365) -> (w364:T28)  [unwired: 1 in]
            n442 = call "subCalculate_SetScaleBar.vi"("ROI in"=w362, "Scale calculation cluster"=w364, "TI-Ctrl"=w371, "error in"=w359, "Handle in"=w354) -> ("error out"=w358:errorcluster, "Handle out"=w353:u32)  [unwired: 5 in]
            n443 = call "subHamamatsu_GetMaxFrameRate.vi"("ROI in"=w362, "error in"=w358, "Handle in"=w353) -> ("error out"=w357:errorcluster, "Handle out"=w356:u32, "max frame rate (Hz)"=w372:dbl)  [unwired: 6 in]
            n444 = property on="max frame rate (Hz)" class="DigNum (strict)"("Value"=w372) -> ()  [unwired: 2 in, 2 out]
            n445 = property on="ROI" class="Clust (strict)"("Value"=w362) -> ()  [unwired: 2 in, 2 out]
            n446 = property on="Live" class="Bool (strict)"() -> ("Value"=w377:bool)  [unwired: 2 in, 2 out]
            n447 = call "subHamamatsu_TurnOnOff.vi"("logic 2"=TRUE ("Status post"), "logic 1"=w377, "error in (no error)"=w357, "Handle in"=w356) -> ("error out"=w380:errorcluster, "Buffer"=w376:T22)  [unwired: 5 in, 1 out]
          }
          event "Camera Ctrl.Exposure (ms)": Value Change {
            n448 = event-data() -> ()  [unwired: 1 in, 1 out]
            n449 = property on="Handle" class="DigNum (strict)"() -> ("Value"=w385:u32)  [unwired: 2 in, 2 out]
            n450 = property on="Exposure (ms)" class="DigNum (strict)"() -> ("Value"=w388:dbl)  [unwired: 2 in, 2 out]
            n451 = call "subHamamatsu_SetExposure.vi"("Exposure (ms)"=w388, "error in (no error)"=w387, "Handle in"=w385) -> ("error out"=w389:errorcluster)  [unwired: 7 in, 1 out]
          }
          event "Run waveform": Value Change {
            n452 = event-data() -> ()  [unwired: 1 in, 1 out]
            n453 = flat-sequence {
              tunnel: [w419] -> w403
              tunnel: w402 -> [w424]
              tunnel: [w437] -> w400
              tunnel: [w450] -> w399
              tunnel: w403 -> [w445]
              tunnel: [w446] -> w401
              tunnel: w400 -> [w444]
              frame #0 {
                # "save TXT file"
                # "If camera is running, turn it off."
                # "Create full folder name with current time"
                n454 = property on="Lasers AO (V)" class="Arr (strict)"(error in=w424) -> (error out=w423:errorcluster, "Value"=w422:dbl[])  [unwired: 1 in, 1 out]
                n455 = property on="Previous Lasers AO (V)" class="Arr (strict)"("Value"=w422) -> ()  [unwired: 2 in, 2 out]
                n456 = property on="Handle" class="DigNum (strict)"() -> ("Value"=w429:u32)  [unwired: 2 in, 2 out]
                n457 = property on="Live" class="Bool (strict)"() -> ("Value"=w432:bool)  [unwired: 2 in, 2 out]
                n458 = call "subHamamatsu_TurnOnOff.vi"("logic 2"=FALSE, "logic 1"=w432, "error in (no error)"=w423, "Handle in"=w429) -> ("error out"=w436:errorcluster, "Handle out"=w431:u32)  [unwired: 5 in, 1 out]
                n459 = property on="Status" class="Str"("Value"="Acquiring .dcimg file" ("Status")) -> ()  [unwired: 2 in, 2 out]
                n460 = property on="DAQ ports" class="Clust (strict)"() -> ("Value"=w427:T25)  [unwired: 2 in, 2 out]
                n461 = call "subDAQ_WaveformPorts.vi"("DAQ ports"=w427, "Waveform channels"="Waveform channels") -> ("Waveform port selection"=w439:T33)  [unwired: 9 in]
                n462 = call "subSave_CreateSubfolder.vi"("Time (F)"=TRUE, "Subfolder name"="Sub-folder", "Base path"="Base folder") -> ("Subfolder"=w405:path)  [unwired: 8 in]
                "Full path" <- w405
                n463 = call "subAcquisition_Waveform.vi"("Waveform info"="Waveform info", "full path"=w405, "error in (no error)"=w436, "Waveform port selection"=w439, "Handle in"=w431) -> ("Error out"=w434:errorcluster, "Acquisition params"=w416:T34, "Handle out"=w437:u32, "AI Waveform"=→"AI Waveform":cluster{"xo":i32, dbl, "data":dbl[][]})  [unwired: 3 in]
                n464 = local read "Stage Status"() -> (w413:T7)
                n465 = local read "Camera Info"() -> (w411:T19)
                n466 = local read "Light control"() -> (w414:T1)
                n467 = local read "Confocal scanner"() -> (w409:T5)
                n468 = local read "Image Info"() -> (w415:T2)
                n469 = local read "Camera Ctrl"() -> (w412:T8)
                n470 = local read "TI-Ctrl"() -> (w410:T9)
                n471 = call "subAcquisition_MovieInfo.vi"("Stage Status"=w413, "Acquisition params"=w416, "Light control"=w414, "Image Info"=w415, "Confocal scanner"=w409, "TI-Ctrl"=w410, "Camera Info"=w411, "Camera Ctrl"=w412) -> ("Text"=w404:string)  [unwired: 3 in]
                n472 = property on="Previous Light control" class="Clust (strict)"() -> ("Value"=w421:T1)  [unwired: 2 in, 2 out]
                n473 = property on="DAQ ports" class="Clust (strict)"() -> ("Value"=w425:T25)  [unwired: 2 in, 2 out]
                n474 = call "subDAQ_SetLaserDO.vi"("DAQ ports"=w425, "Error in (no error)"=w434) -> ("Error out"=w426:errorcluster)  [unwired: 9 in]
                n475 = Build Path(base path=w405, name or relative path="movie_info.txt") -> (appended path=w406:path)
                n476 = call "subDAQ_SetLaserAO.vi"("DAQ ports"=w425, "Light control (All off)"=w421, "Error in (no error)"=w426) -> ("Error out"=w420:errorcluster)  [unwired: 8 in]
                n477 = property on="Lasers DO" class="Arr (strict)"(error in=w420, "Value"=bool[] [FALSE, FALSE, FALSE, FALSE, FALSE, FALSE]) -> (error out=w419:errorcluster)  [unwired: 1 in, 1 out]
                n478 = Write to Text File(file (use dialog)=w406, text=w404) -> ()  [unwired: 2 in, 3 out]
              }
              frame #1 {
                # "Reset camera settings"
                n479 = property on="Exposure (ms)" class="DigNum (strict)"() -> ("Value"=w441:dbl)  [unwired: 2 in, 2 out]
                n480 = local write "Run waveform"(FALSE) -> ()
                n481 = call "subHamamatsu_SetExposure.vi"("Exposure (ms)"=w441, "error in (no error)"=w445, "Handle in"=w444) -> ("error out"=w447:errorcluster, "Handle out"=w449:u32)  [unwired: 7 in]
                n482 = property on="Status" class="Str"("Value"="ready" ("Status")) -> ()  [unwired: 2 in, 2 out]
                n483 = property on="Live" class="Bool (strict)"() -> ("Value"=w442:bool)  [unwired: 2 in, 2 out]
                n484 = call "subHamamatsu_TurnOnOff.vi"("logic 2"=TRUE, "logic 1"=w442, "error in (no error)"=w447, "Handle in"=w449) -> ("error out"=w446:errorcluster, "Buffer"=w450:T22)  [unwired: 5 in, 1 out]
              }
            }
            n485 = control-ref of="Snap Number Counting"() -> (w394:refnum<vi>)
            n486 = control-ref of="Movie Point  Y Array"() -> (w391:refnum<vi>)
            n487 = control-ref of="Movie Point  X Array"() -> (w392:refnum<vi>)
            n488 = property on="Snap Number Counting" class="DigNum (strict)"() -> ("Value"=w393:dbl)  [unwired: 2 in, 2 out]
            n489 = control-ref of="Record Table"() -> (w390:refnum<vi>)
            n490 = property on="Stage Status" class="Clust (strict)"() -> ("Value"=w398:T7)  [unwired: 2 in, 2 out]
            n491 = call "subDAQ_GetMoviePoint.vi"("Recorde Table Refnum"=w390, "Snap Number Refnum"=w394, "Movie Point Y Arr Refnum"=w391, "Movie Point X Arr Refnum"=w392, "Snap Number Counting"=w393, "Stage Status"=w398) -> ("Snap/Movie Point cluster"=→"Movie Point cluster":cluster{"Snap Y":dbl[], "Snap X":dbl[]}, "Movie Point  Y Array"=→"Movie Point  Y Array":dbl[], "Movie Point  X Array"=→"Movie Point  X Array":dbl[])  [unwired: 3 in]
          }
          event "Stream movie": Value Change {
            n492 = event-data() -> ()  [unwired: 1 in, 1 out]
            n493 = flat-sequence {
              tunnel: w468 -> [w477]
              tunnel: [w485] -> w467
              tunnel: [w479] -> w466
              tunnel: [w478] -> w465
              tunnel: w467 -> [w505]
              tunnel: w466 -> [w495]
              tunnel: w465 -> [w501]
              tunnel: [w500] -> w464
              tunnel: [w499] -> w462
              tunnel: [w508] -> w463
              tunnel: w464 -> [w508]
              tunnel: w462 -> [w507]
              tunnel: [w507] -> w461
              frame #0 {
                n494 = property on="Handle" class="DigNum (strict)"() -> ("Value"=w470:u32)  [unwired: 2 in, 2 out]
                n495 = local read "Sub-folder"() -> (w473:string)
                n496 = local read "Base folder"() -> (w474:path)
                n497 = property on="Live" class="Bool (strict)"() -> ("Value"=w471:bool)  [unwired: 2 in, 2 out]
                n498 = call "subHamamatsu_TurnOnOff.vi"("logic 2"=FALSE, "logic 1"=w471, "error in (no error)"=w477, "Handle in"=w470) -> ("error out"=w484:errorcluster, "Handle out"=w469:u32)  [unwired: 5 in, 1 out]
                n499 = call "subSave_CreateSubfolder.vi"("Subfolder name"=w473, "Base path"=w474) -> ("Subfolder"=w475:path)  [unwired: 9 in]
                n500 = local read "Movie frame rate (Hz)"() -> (w480:dbl)
                n501 = property on="Status" class="Str"("Value"="Stream movie" ("Status")) -> ()  [unwired: 2 in, 2 out]
                n502 = Build Path(base path=w475, name or relative path="movie.dcimg" ("string")) -> (appended path=w485:path)
                n503 = local read "# frames"() -> (w483:i32)
                n504 = control-ref of="Frames Recorded"() -> (w481:refnum<vi>)
                n505 = control-ref of="Elapsed time (sec)"() -> (w482:refnum<vi>)
                n506 = call "subAcquisition_StreamMovie.vi"("Elapsed time (sec) Refnum"=w482, "Frames Recorded Refnum"=w481, "File path"=w485, "error in (no error)"=w484, "Movie frame rate (Hz)"=w480, "# frames"=w483, "Handle in"=w469) -> ("error out"=w478:errorcluster, "Handle out"=w479:u32)  [unwired: 3 in]
              }
              frame #1 {
                n507 = local read "Camera Ctrl"() -> (w488:T8)
                n508 = local read "Camera Info"() -> (w487:T19)
                n509 = local read "Image Info"() -> (w489:T2)
                n510 = local read "TI-Ctrl"() -> (w494:T9)
                n511 = local read "Confocal scanner"() -> (w493:T5)
                n512 = property on="Exposure (ms)" class="DigNum (strict)"() -> ("Value"=w498:dbl)  [unwired: 2 in, 2 out]
                n513 = local read "Light control"() -> (w492:T1)
                n514 = local read "Stage Status"() -> (w491:T7)
                n515 = call "subHamamatsu_SetExposure.vi"("Exposure (ms)"=w498, "error in (no error)"=w501, "Handle in"=w495) -> ("error out"=w504:errorcluster, "Handle out"=w503:u32)  [unwired: 7 in]
                n516 = call "subAcquisition_Info.vi"("Stage Status"=w491, "Light control"=w492, "Image Info"=w489, "Confocal scanner"=w493, "TI-Ctrl"=w494, "Camera Info"=w487, "Camera Ctrl"=w488) -> ("Text"=w490:string)  [unwired: 4 in]
                n517 = property on="Live" class="Bool (strict)"() -> ("Value"=w497:bool)  [unwired: 2 in, 2 out]
                n518 = property on="Status" class="Str"("Value"="Saving binary file" ("Status")) -> ()  [unwired: 2 in, 2 out]
                n519 = call "subSave_Dcimg2Bin.vi"("Text"=w490, ".dcimg file name"=w505) -> ()  [unwired: 9 in, 1 out]
                n520 = call "subHamamatsu_TurnOnOff.vi"("logic 2"=TRUE, "logic 1"=w497, "error in (no error)"=w504, "Handle in"=w503) -> ("error out"=w500:errorcluster, "Buffer"=w499:T22)  [unwired: 5 in, 1 out]
              }
              frame #2 {
                n521 = local write "Stream movie"(FALSE ("Acquire movie")) -> ()
                n522 = property on="Status" class="Str"("Value"="ready" ("Status")) -> ()  [unwired: 2 in, 2 out]
              }
            }
            n523 = control-ref of="Snap Number Counting"() -> (w456:refnum<vi>)
            n524 = control-ref of="Movie Point  Y Array"() -> (w459:refnum<vi>)
            n525 = control-ref of="Movie Point  X Array"() -> (w458:refnum<vi>)
            n526 = property on="Snap Number Counting" class="DigNum (strict)"() -> ("Value"=w457:dbl)  [unwired: 2 in, 2 out]
            n527 = control-ref of="Record Table"() -> (w460:refnum<vi>)
            n528 = property on="Stage Status" class="Clust (strict)"() -> ("Value"=w455:T7)  [unwired: 2 in, 2 out]
            n529 = call "subDAQ_GetMoviePoint.vi"("Recorde Table Refnum"=w460, "Snap Number Refnum"=w456, "Movie Point Y Arr Refnum"=w459, "Movie Point X Arr Refnum"=w458, "Snap Number Counting"=w457, "Stage Status"=w455) -> ("Snap/Movie Point cluster"=w452:cluster{"Snap Y":dbl[], "Snap X":dbl[]}, "Movie Point  Y Array"=w453:dbl[], "Movie Point  X Array"=w454:dbl[])  [unwired: 3 in]
            n530 = local write "Movie Point  X Array"(w454) -> ()
            n531 = local write "Movie Point  Y Array"(w453) -> ()
            n532 = local write "Movie Point cluster"(w452) -> ()
          }
          event "MD acquisition": Value Change {
            # "Timelapse Loop"
            # "Multidimensional acquisition"
            n533 = event-data() -> ()  [unwired: 1 in, 1 out]
            n534 = property on="Handle" class="DigNum (strict)"() -> ("Value"=w513:u32)  [unwired: 2 in, 2 out]
            n535 = property on="Live" class="Bool (strict)"() -> ("Value"=w514:bool)  [unwired: 2 in, 2 out]
            n536 = local read "Timelapse?"() -> (w512:bool)
            n537 = call "subHamamatsu_TurnOnOff.vi"("logic 2"=FALSE, "logic 1"=w514, "error in (no error)"=w526, "Handle in"=w513) -> ("error out"=w522:errorcluster)  [unwired: 5 in, 2 out]
            n538 = case shown="True" w512 {
              tunnel: [1 ("Timelapse Cycles") "Timelapse Cycles"] -> w511
              tunnel: [u32 0 "Period (s)"] -> w510
              frame False {
              }
              frame True {
                n539 = property on="T Acquired Progress" class="Slide (strict)"("Scale.Maximum"="Timelapse Cycles") -> ()  [unwired: 2 in, 2 out]
              }
            }
            n540 = local read "Base folder"() -> (w516:path)
            n541 = local read "Sub-folder"() -> (w518:string)
            n542 = call "subSave_CreateSubfolder.vi"("Time (F)"=TRUE, "Subfolder name"=w518, "Base path"=w516) -> ("Subfolder"=w515:path)  [unwired: 8 in]
            n543 = Tick Count (ms)() -> (millisecond timer value=w520:u32)
            n544 = for {
              N: w511 -> [_]
              tunnel: w520 -> [w567]
              tunnel: w510 -> [w545]
              shift-right: [w536] -> w521
              shift-left: w522 -> [w559]
              tunnel: "Channel settings" -> [w548]
              tunnel: w515 -> [w543]
              i -> [w566]
              # "Cycle through Colors"
              # "Wait for next time point"
              n545 = Tick Count (ms)() -> (millisecond timer value=w569:u32)
              n546 = Subtract(x=w569, y=w567) -> (x-y=w570:u32)
              n547 = local read "Timelapse Cycles"() -> (w546:i32)
              n548 = Increment(x=w566) -> (x+1=w547:i32)
              n549 = Divide(x=w570, y=1000.0) -> (x/y=w537:dbl)
              n550 = Unbundle By Name(w548) -> ("Name"=w562:string[], "Take?"=w563:bool[], "Cumulation"=w550:i32[], "Exposure time (msec)"=w551:dbl[])
              n551 = Multiply(x=u32 1000 ("y"), y=w545) -> (x*y=w549:u32)
              n552 = local read "TiE Ref"() -> (w556:T21)
              n553 = control-ref of="TI-Ctrl"() -> (w555:refnum<vi>)
              n554 = control-ref of="Light control"() -> (w553:refnum<vi>)
              n555 = control-ref of="Confocal scanner"() -> (w552:refnum<vi>)
              n556 = property on="DAQ ports" class="Clust (strict)"() -> ("Value"=w542:T25)  [unwired: 2 in, 2 out]
              n557 = property on="Confocal VISA Setting" class="VISAName"() -> ("Value"=w540:refnum<visa-resource-name>)  [unwired: 2 in, 2 out]
              n558 = property on="Channel" class="Arr (strict)"() -> ("Value"=w558:i32[])  [unwired: 2 in, 2 out]
              n559 = property on="Timelapse Time (s)" class="DigNum (strict)"("Value"=w537) -> ()  [unwired: 2 in, 2 out]
              n560 = property on="Take?" class="Arr (strict)"() -> ("Value"=w557:bool[])  [unwired: 2 in, 2 out]
              n561 = To Long Integer(number=w558) -> (32bit integer=w564:i32[])
              n562 = Bundle("TI-Ctrl"=w555, "TiE Ref"=w556) -> (w554:T35)  [unwired: 1 in]
              n563 = Array Size(array=w557) -> (size(s)=w561:i32)
              n564 = Greater?(x=w546, y=w547) -> (0:w565:bool)
              n565 = for {
                N: w561 -> [_]
                tunnel: w563 -> [w581] mode=indexing
                tunnel: w564 -> [w579] mode=indexing
                shift-right: [w583] -> w560
                shift-left: w559 -> [w584]
                tunnel: w543 -> [w582]
                tunnel: w562 -> [w580] mode=indexing
                tunnel: w554 -> [w578]
                tunnel: w551 -> [w577] mode=indexing
                tunnel: w553 -> [w576]
                tunnel: w552 -> [w575]
                tunnel: w542 -> [w574]
                tunnel: w550 -> [w573] mode=indexing
                tunnel: w547 -> [w572]
                tunnel: w540 -> [w571]
                n566 = case shown="True" w581 {
                  tunnel: w584 -> [w585 w588]
                  tunnel: [w585 w613] -> w583
                  tunnel: w582 -> [_ w616]
                  tunnel: w580 -> [_ w598]
                  tunnel: w579 -> [_ w589]
                  tunnel: w578 -> [_ w611]
                  tunnel: w577 -> [_ w594]
                  tunnel: w576 -> [_ w610]
                  tunnel: w575 -> [_ w609]
                  tunnel: w574 -> [_ w608]
                  tunnel: w573 -> [_ w599]
                  tunnel: w572 -> [_ w590]
                  tunnel: w571 -> [_ w591]
                  frame False {
                  }
                  frame True {
                    # "Filter Set cluster"
                    # "stage cluster"
                    # "zstack cluster"
                    n567 = control-ref of="Color Acquiring"() -> (w587:refnum<vi>)
                    n568 = Bundle("Filter Set"=w589, "Light control"=w610, "Confocal scanner"=w609, "Value"=w608, "Value"=w591) -> (w592:T36)  [unwired: 1 in]
                    n569 = call "subAcquisition_AcquirngColor.vi"("Bool Refnum"=w587, "Filter Set"=w589) -> ()  [unwired: 10 in]
                    n570 = Build Path(base path=w616, name or relative path=w598) -> (appended path=w603:path)
                    n571 = call "subDAQ_SetFilterSet.vi"("Ti-E cluster"=w611, "Filterset cluster"=w592, "error in"=w588) -> ("error out"=w615:errorcluster)  [unwired: 8 in]
                    n572 = property on="Handle" class="DigNum (strict)"() -> ("Value"=w593:u32)  [unwired: 2 in, 2 out]
                    n573 = local read "Timelapse?"() -> (w596:bool)
                    n574 = call "subHamamatsu_SetExposure.vi"("Exposure (ms)"=w594, "error in (no error)"=w615, "Handle in"=w593) -> ("error out"=w614:errorcluster, "Handle out"=w612:u32)  [unwired: 7 in]
                    n575 = Select(t=w590, s=w596, f=0) -> (s? t:f=w595:i32)
                    n576 = local read "Z-Stack"() -> (w607:T10)
                    n577 = control-ref of="Image Info"() -> (w605:refnum<vi>)
                    n578 = local read "Camera Ctrl"() -> (w606:T8)
                    n579 = local read "XY tiling"() -> (w602:T12)
                    n580 = control-ref of="Stage Status"() -> (w601:refnum<vi>)
                    n581 = control-ref of="Z Stack Aquired"() -> (w586:refnum<vi>)
                    n582 = Bundle("XY tiling"=w602, "Stage Status"=w601) -> (w600:T37)  [unwired: 1 in]
                    n583 = Bundle(w595, "appended path"=w603, "Z-Stack"=w607, "Arch_Dragon cumulation"=w599, "Image Info"=w605, "Camera Ctrl"=w606) -> (w604:T38)  [unwired: 1 in]
                    n584 = call "subAcquisition_3D.vi"("Z-stack cluster in"=w604, "Ti-E cluster"=w611, "Stage cluster"=w600, "error in"=w614, "Z Stack Aquired Refnum"=w586, "Handle in"=w612) -> ("error out"=w613:errorcluster)  [unwired: 5 in]
                    "Timelapse Acquired" <- w590
                    "T Acquired Progress" <- w590
                  }
                }
              }
              n585 = case shown="True" w565 {
                tunnel: w549 -> [_ w617]
                frame False {
                }
                frame True {
                  n586 = Wait (ms)(milliseconds to wait=w617) -> ()  [unwired: 1 out]
                }
              }
              n587 = property on="DAQ ports" class="Clust (strict)"() -> ("Value"=w541:T25)  [unwired: 2 in, 2 out]
              n588 = call "subDAQ_SetLaserDO.vi"("DAQ ports"=w541, "Error in (no error)"=w560) -> ("Error out"=w539:errorcluster)  [unwired: 9 in]
              n589 = property on="Lasers DO" class="Arr (strict)"(error in=w539, "Value"=bool[] [FALSE, FALSE, FALSE, FALSE, FALSE, FALSE]) -> (error out=w535:errorcluster)  [unwired: 1 in, 1 out]
              n590 = Bundle(u32 1985280, u32 16448250) -> (w533:cluster{u32, u32})  [unwired: 1 in]
              n591 = Build Array(w533) -> (w531:cluster{u32, u32}[])
              n592 = property on="Color Acquiring" class="Bool (strict)"(error in=w535, "Colors [4]"=w531) -> (error out=w536:errorcluster)  [unwired: 1 in, 1 out]
            }
            n593 = flat-sequence {
              tunnel: w521 -> [w622]
              tunnel: [w626] -> w525
              tunnel: [w625] -> w524
              frame #0 {
                n594 = property on="Handle" class="DigNum (strict)"() -> ("Value"=w618:u32)  [unwired: 2 in, 2 out]
                n595 = property on="Exposure (ms)" class="DigNum (strict)"() -> ("Value"=w620:dbl)  [unwired: 2 in, 2 out]
                n596 = call "subHamamatsu_SetExposure.vi"("Exposure (ms)"=w620, "error in (no error)"=w622, "Handle in"=w618) -> ("error out"=w624:errorcluster, "Handle out"=w623:u32)  [unwired: 7 in]
                n597 = local write "MD acquisition"(FALSE ("Capture")) -> ()
                n598 = property on="Live" class="Bool (strict)"() -> ("Value"=w619:bool)  [unwired: 2 in, 2 out]
                n599 = call "subHamamatsu_TurnOnOff.vi"("logic 2"=TRUE, "logic 1"=w619, "error in (no error)"=w624, "Handle in"=w623) -> ("error out"=w626:errorcluster, "Buffer"=w625:T22)  [unwired: 5 in, 1 out]
              }
            }
          }
        }
      }
      "Camera" <- w36
      n600 = while {
        shift-right: [w1034] -> _
        shift-left: errorcluster {"status"=FALSE, "code"=0, "source"=""} ("Error out") -> [w1035]
        stop <- w1033 stop-if-true
        # "Light control"
        n601 = event shown="[5] \"Light control.Filter Set\": Value Change" {
          selector: _ -> [_ _ _ _ _ _]
          dyn-events: _ -> [_ _ _ _ _ _]
          timeout: 50 -> [_ _ _ _ _ _]
          tunnel: w1035 -> [w1037 w1040 w1045 w1049 w1052 w1064]
          tunnel: [w1037 w1041 w1044 w1048 w1053 w1063] -> w1034
          event Timeout {
            n602 = event-data() -> ()  [unwired: 1 in, 1 out]
          }
          event "Light control.Lasers AO (V)": Value Change {
            n603 = event-data() -> ()  [unwired: 1 in, 1 out]
            n604 = local read "Light control"() -> (w1039:T1)
            n605 = property on="DAQ ports" class="Clust (strict)"() -> ("Value"=w1038:T25)  [unwired: 2 in, 2 out]
            n606 = call "subDAQ_SetLaserAO.vi"("DAQ ports"=w1038, "Light control (All off)"=w1039, "Error in (no error)"=w1040) -> ("Error out"=w1041:errorcluster)  [unwired: 8 in]
          }
          event "Light control.Lasers DO": Value Change {
            n607 = event-data() -> ()  [unwired: 1 in, 1 out]
            n608 = local read "Light control"() -> (w1043:T1)
            n609 = property on="DAQ ports" class="Clust (strict)"() -> ("Value"=w1042:T25)  [unwired: 2 in, 2 out]
            n610 = call "subDAQ_SetLaserDO.vi"("DAQ ports"=w1042, "Light control (All off)"=w1043, "Error in (no error)"=w1045) -> ("Error out"=w1044:errorcluster)  [unwired: 8 in]
          }
          event "Light control.LED": Value Change {
            n611 = event-data() -> ()  [unwired: 1 in, 1 out]
            n612 = property on="DAQ ports" class="Clust (strict)"() -> ("Value"=w1046:T25)  [unwired: 2 in, 2 out]
            n613 = local read "Light control"() -> (w1047:T1)
            n614 = call "subDAQ_SetLED.vi"("DAQ ports"=w1046, "Light control (All Off)"=w1047, "Error in (no error)"=w1049) -> ("Error out"=w1048:errorcluster)  [unwired: 8 in]
          }
          event "Light control.Global": Value Change {
            n615 = event-data() -> ()  [unwired: 1 in, 1 out]
            n616 = local read "Light control"() -> (w1051:T1)
            n617 = property on="DAQ ports" class="Clust (strict)"() -> ("Value"=w1050:T25)  [unwired: 2 in, 2 out]
            n618 = call "subDAQ_SetGlobal.vi"("DAQ ports"=w1050, "Light control (All off)"=w1051, "Error in (no error)"=w1052) -> ("Error out"=w1053:errorcluster)  [unwired: 8 in]
          }
          event "Light control.Filter Set": Value Change {
            n619 = event-data() -> ("NewVal"=w1059:i32)  [unwired: 1 in]
            n620 = property on="DAQ ports" class="Clust (strict)"() -> ("Value"=w1055:T25)  [unwired: 2 in, 2 out]
            n621 = control-ref of="Light control"() -> (w1058:refnum<vi>)
            n622 = control-ref of="Confocal scanner"() -> (w1057:refnum<vi>)
            n623 = property on="Confocal VISA Setting" class="VISAName"() -> ("Value"=w1054:refnum<visa-resource-name>)  [unwired: 2 in, 2 out]
            n624 = local read "TiE Ref"() -> (w1061:T21)
            n625 = control-ref of="TI-Ctrl"() -> (w1062:refnum<vi>)
            n626 = Bundle("NewVal"=w1059, "Light control"=w1058, "Confocal scanner"=w1057, "Value"=w1055, "Value"=w1054) -> (w1056:T39)  [unwired: 1 in]
            n627 = Bundle("TI-Ctrl"=w1062, "TiE Ref"=w1061) -> (w1060:T35)  [unwired: 1 in]
            n628 = call "subDAQ_SetFilterSet.vi"("Ti-E cluster"=w1060, "Filterset cluster"=w1056, "error in"=w1064) -> ("error out"=w1063:errorcluster)  [unwired: 8 in]
          }
        }
        n629 = local read "stop program"() -> (w1033:bool)
      }
      n630 = while {
        stop <- w39 stop-if-true
        # "Waveforms"
        n631 = event shown="[1] \"Load waveform\": Value Change" {
          selector: _ -> [_ _]
          dyn-events: _ -> [_ _]
          timeout: 50 -> [_ _]
          event Timeout {
            n632 = event-data() -> ()  [unwired: 1 in, 1 out]
          }
          event "Load waveform": Value Change {
            n633 = event-data() -> ()  [unwired: 1 in, 1 out]
            n634 = local read "Waveform channels"() -> (w46:T13)
            n635 = property on="DAQ ports" class="Clust (strict)"() -> ("Value"=w41:T25)  [unwired: 2 in, 2 out]
            n636 = local read "Waveform info"() -> (w47:T14)
            n637 = call "subDAQ_WaveformPorts.vi"("DAQ ports"=w41, "Waveform channels"=w46) -> ("Waveform port selection"=w45:T33)  [unwired: 9 in]
            n638 = call "subDAQ_GenWaveform.vi"("Waveform port selection"=w45, "Waveform info"=w47) -> ("error out"=w43:errorcluster, "Dev1 AO waveform"=→"Patch Ex. Command AO waveform":waveform(dbl), "Lasers AO waveform"=→"Lasers AO waveform":waveform(dbl)[], "Lasers DO waveform"=→"Lasers DO waveform":digitalwaveform[])  [unwired: 5 in, 1 out]
            n639 = property on="Load waveform" class="Bool (strict)"(error in=w43, "Value"=FALSE ("Load arbitrary waveform")) -> ()  [unwired: 1 in, 2 out]
          }
        }
        n640 = local read "stop program"() -> (w39:bool)
      }
      n641 = while {
        stop <- w929 stop-if-true
        # "Nikon control"
        n642 = event shown="[2] \"TI-Ctrl.Obj\": Value Change" {
          selector: _ -> [_ _ _ _ _ _ _ _ _ _ _ _ _ _]
          dyn-events: _ -> [_ _ _ _ _ _ _ _ _ _ _ _ _ _]
          timeout: 50 -> [_ _ _ _ _ _ _ _ _ _ _ _ _ _]
          event Timeout {
            # "This part reads the info\nfrom the microscope\n(based on what as been \ndeclared at the beginning)"
            n643 = event-data() -> ()  [unwired: 1 in, 2 out]
            n644 = local read "Ti-E initialized"() -> (w930:bool)
            n645 = case shown="True" w930 {
              frame False {
              }
              frame True {
                n646 = local read "TiE Ref"() -> (w936:T21)
                n647 = property on="Home" class="Bool (strict)"() -> ("Value"=w934:bool)  [unwired: 2 in, 2 out]
                n648 = call "subTiE_GetStatus.vi"("Ref"=w936) -> ("TI-Ctrl"=w935:T40)
                n649 = Select(t=T23."Disabled and Grayed Out" ("Disabled"), s=w934, f=T23."Enabled" ("Disabled")) -> (s? t:f=w931:T23)
                n650 = local write "TI-Ctrl"(w935) -> ()
                n651 = property on="Z-pos" class="DigNum (strict)"("DisabledEnum"=w931) -> ()  [unwired: 2 in, 2 out]
              }
            }
          }
          event "Scope on?": Value Change {
            n652 = event-data() -> ("NewVal"=w939:bool)  [unwired: 1 in]
            n653 = case shown="True" w939 {
              tunnel: [T23."Disabled and Grayed Out" ("Disabled") T23."Enabled" ("Disabled")] -> w938
              tunnel: [FALSE ("Ti-E initialized") TRUE ("Ti-E initialized")] -> w937
              frame False {
                n654 = local read "TiE Ref"() -> (w940:T21)
                n655 = call "subTiE_Deinitialize.vi"("Ref"=w940) -> ()  [unwired: 11 in]
              }
              frame True {
                n656 = flat-sequence {
                  frame #0 {
                    n657 = property on="Status" class="Str"("Value"="Initializing Nikon ..." ("Status")) -> ()  [unwired: 2 in, 2 out]
                  }
                  frame #1 {
                    n658 = local read "log path"() -> (w946:path)
                    n659 = call "subTiE_Initialize.vi"("Ti Control Lib"="Ti Control Lib") -> ("Ref"=→"TiE Ref":T21)  [unwired: 10 in]
                    n660 = call "subRegist_AddInfoIntoText.vi"("log path"=w946, "info to be added"=" Ti-E") -> ()  [unwired: 10 in]
                  }
                  frame #2 {
                    n661 = property on="Status" class="Str"("Value"="Ready" ("Status")) -> ()  [unwired: 2 in, 2 out]
                  }
                }
              }
            }
            "Ti-E initialized" <- w937
            n662 = property on="TI-Ctrl" class="Clust (strict)"("DisabledEnum"=w938) -> ()  [unwired: 2 in, 2 out]
          }
          event "TI-Ctrl.Obj": Value Change {
            n663 = event-data() -> ()  [unwired: 1 in, 1 out]
            n664 = local read "TiE Ref"() -> (w959:T21)
            n665 = local read "TI-Ctrl"() -> (w961:T9)
            n666 = call "subTiE_SetZEscape.vi"("Ref"=w959, "TI-Ctrl"=w961) -> ("error out"=w960:errorcluster)  [unwired: 9 in]
            n667 = call "subTiE_SetObjective.vi"("TiE Ref"=w959, "TI-Ctrl"=w961, "error in"=w960) -> ()  [unwired: 8 in, 1 out]
            n668 = property on="Handle" class="DigNum (strict)"() -> ("Value"=w958:u32)  [unwired: 2 in, 2 out]
            n669 = local read "TI-Ctrl"() -> (w957:T9)
            n670 = property on="ROI" class="Clust (strict)"() -> ("Value"=w956:T3)  [unwired: 2 in, 2 out]
            n671 = control-ref of="scale bar (μm)"() -> (w952:refnum<vi>)
            n672 = control-ref of="Total y width (μm)"() -> (w954:refnum<vi>)
            n673 = control-ref of="Pixel size (nm)"() -> (w953:refnum<vi>)
            n674 = control-ref of="Total x width (μm)"() -> (w955:refnum<vi>)
            n675 = Bundle("Total x width (μm)"=w955, "Total y width (μm)"=w954, "Pixel size (nm)"=w953, "scale bar (μm)"=w952) -> (w951:T28)  [unwired: 1 in]
            n676 = call "subCalculate_SetScaleBar.vi"("ROI in"=w956, "Scale calculation cluster"=w951, "TI-Ctrl"=w957, "Handle in"=w958) -> ()  [unwired: 6 in, 2 out]
          }
          event "TI-Ctrl.Lightpath": Value Change {
            # "Change this into subVI: \nsubTiE_SetLightpath"
            n677 = event-data() -> ()  [unwired: 1 in, 1 out]
            n678 = local read "TI-Ctrl"() -> (w966:T9)
            n679 = local read "TiE Ref"() -> (w965:T21)
            n680 = Unbundle By Name(w966) -> ("Lightpath"=w963:enum32{"EYE", "L100", "R100", "L80"})
            n681 = Unbundle By Name(w965) -> ("LightPathDrive"=w964:refnum<k7>)
            n682 = Increment(x=w963) -> (x+1=w962:enum32{"EYE", "L100", "R100", "L80"})
            n683 = To Variant(anything=w962) -> (Variant=w967:variant)
            n684 = property class="ILightPathDrive"(reference=w964, "Position"=w967) -> ()  [unwired: 1 in, 2 out]
          }
          event "TI-Ctrl.Z-Ctrl.Z-pos": Value Change {
            n685 = event-data() -> ()  [unwired: 1 in, 1 out]
            n686 = local read "TiE Ref"() -> (w968:T21)
            n687 = local read "TI-Ctrl"() -> (w969:T9)
            n688 = call "subTiE_SetZPos.vi"("Ref"=w968, "TI-Ctrl"=w969) -> ()  [unwired: 9 in, 1 out]
          }
          event "TI-Ctrl.Z-Ctrl.Sensitivity": Value Change {
            # "Change this into subVI: \nsubTiE_SetZSensitivity"
            n689 = event-data() -> ()  [unwired: 1 in, 1 out]
            n690 = local read "TI-Ctrl"() -> (w977:T9)
            n691 = local read "TiE Ref"() -> (w976:T21)
            n692 = Unbundle By Name(w977) -> ("Z-Ctrl.Sensitivity"=w971:u8)
            n693 = Unbundle By Name(w976) -> ("ZDrive"=w975:refnum<k7>)
            n694 = Decrement(x=w971) -> (x-1=w973:u8)
            n695 = Multiply(x=w973, y=u8 3) -> (x*y=w974:u8)
            n696 = Increment(x=w974) -> (x+1=w970:u8)
            n697 = To Variant(anything=w970) -> (Variant=w978:variant)
            n698 = property class="IZDrive"(reference=w975, "DialSensitivity"=w978) -> ()  [unwired: 1 in, 2 out]
          }
          event "TI-Ctrl.Z-Ctrl.Home": Value Change {
            # "Home = Escape"
            n699 = event-data() -> ()  [unwired: 1 in, 1 out]
            n700 = local read "TiE Ref"() -> (w980:T21)
            n701 = local read "TI-Ctrl"() -> (w979:T9)
            n702 = call "subTiE_SetZEscape.vi"("Ref"=w980, "TI-Ctrl"=w979) -> ()  [unwired: 9 in, 1 out]
          }
          event "TI-Ctrl.PFS-Ctrl.PFS IO": Value Change {
            # "Change this into subVI: \nsubTiE_SetPFSonOff"
            # "PFS Status\n1: PFS Possible\n2: tmp\n4,5: ON (no idea the difference)\n6: DIS\n7: NOT POSSIBLE"
            n703 = event-data() -> ()  [unwired: 1 in, 1 out]
            n704 = local read "TiE Ref"() -> (w982:T21)
            n705 = Unbundle By Name(w982) -> ("PFS"=w981:refnum<k7>)
            n706 = property class="IPFS"(reference=w981) -> (reference out=w986:refnum<k7>, "Status"=w984:variant, "IsEnabled"=w988:variant)  [unwired: 1 in, 1 out]
            n707 = Variant To Data(type=0, Variant=w984) -> (data=w985:i32)  [unwired: 1 in, 1 out]
            n708 = Variant To Data(type=0, Variant=w988) -> (data=w989:i32)  [unwired: 1 in, 1 out]
            n709 = case shown="1" w985 {
              tunnel: w986 -> [w990 _ w997]
              tunnel: w989 -> [_ _ _]
              frame Default {
                n710 = local read "TI-Ctrl"() -> (w992:T9)
                n711 = Unbundle By Name(w992) -> ("PFS-Ctrl.PFS IO"=w991:bool)
                n712 = case shown="False" w991 {
                  selector: w991 -> [w994 _]
                  tunnel: w990 -> [w993 _]
                  frame False {
                    n713 = Boolean To (0,1)(Boolean=w994) -> (0, 1=w996:i16)
                    n714 = To Variant(anything=w996) -> (Variant=w995:variant)
                    n715 = property class="IPFS"(reference=w993, "IsEnabled"=w995) -> ()  [unwired: 1 in, 2 out]
                  }
                  frame True {
                  }
                }
              }
              frame 7 {
              }
              frame 1 {
                n716 = local read "TI-Ctrl"() -> (w999:T9)
                n717 = Unbundle By Name(w999) -> ("PFS-Ctrl.PFS IO"=w998:bool)
                n718 = case shown="True" w998 {
                  selector: w998 -> [_ w1001]
                  tunnel: w997 -> [_ w1000]
                  frame False {
                  }
                  frame True {
                    n719 = Boolean To (0,1)(Boolean=w1001) -> (0, 1=w1003:i16)
                    n720 = To Variant(anything=w1003) -> (Variant=w1002:variant)
                    n721 = property class="IPFS"(reference=w1000, "IsEnabled"=w1002) -> ()  [unwired: 1 in, 2 out]
                  }
                }
              }
            }
          }
          event "TI-Ctrl.PFS-Ctrl.PSF Pos": Value Change {
            # "Change this into subVI: \nsubTiE_SetPFSpos"
            # "PFS Status\n1: PFS Possible\n2: tmp\n4,5: ON (no idea the difference)\n6: DIS\n7: NOT POSSIBLE"
            n722 = event-data() -> ()  [unwired: 1 in, 1 out]
            n723 = local read "TiE Ref"() -> (w1005:T21)
            n724 = Unbundle By Name(w1005) -> ("PFS"=w1004:refnum<k7>)
            n725 = property class="IPFS"(reference=w1004) -> (reference out=w1009:refnum<k7>, "Status"=w1007:variant)  [unwired: 1 in, 1 out]
            n726 = Variant To Data(type=0, Variant=w1007) -> (data=w1008:i32)  [unwired: 1 in, 1 out]
            n727 = case shown="4, 5" w1008 {
              tunnel: w1009 -> [_ w1013]
              frame Default {
              }
              frame 4, 5 {
                n728 = local read "TI-Ctrl"() -> (w1011:T9)
                n729 = Unbundle By Name(w1011) -> ("PFS-Ctrl.PSF Pos"=w1012:u32)
                n730 = To Variant(anything=w1012) -> (Variant=w1010:variant)
                n731 = property class="IPFS"(reference=w1013, "Position"=w1010) -> ()  [unwired: 1 in, 2 out]
              }
            }
          }
          event "TI-Ctrl.Condenser": Value Change {
            # "Change this into subVI: \nsubTiE_SetCondenser"
            n732 = event-data() -> ()  [unwired: 1 in, 1 out]
            n733 = local read "TiE Ref"() -> (w1016:T21)
            n734 = local read "TI-Ctrl"() -> (w1017:T9)
            n735 = Unbundle By Name(w1016) -> ("CondenserCassette"=w1015:refnum<k7>)
            n736 = Unbundle By Name(w1017) -> ("Condenser"=w1014:u16)
            n737 = To Variant(anything=w1014) -> (Variant=w1018:variant)
            n738 = property class="ICondenserCassette"(reference=w1015, "Position"=w1018) -> ()  [unwired: 1 in, 2 out]
          }
          event "TI-Ctrl.Cube Bottom": Value Change {
            n739 = event-data() -> ()  [unwired: 1 in, 1 out]
            n740 = local read "TI-Ctrl"() -> (w1019:T9)
            n741 = local read "TiE Ref"() -> (w1020:T21)
            n742 = call "subTiE_SetCubeBottom.vi"("Ref"=w1020, "TI-Ctrl"=w1019) -> ()  [unwired: 10 in]
          }
          event "TI-Ctrl.Cube Top": Value Change {
            n743 = event-data() -> ()  [unwired: 1 in, 1 out]
            n744 = local read "TI-Ctrl"() -> (w1021:T9)
            n745 = local read "TiE Ref"() -> (w1022:T21)
            n746 = call "subTiE_SetCubeTop.vi"("Ref"=w1022, "TI-Ctrl"=w1021) -> ()  [unwired: 10 in]
          }
          event "Define 1": Value Change {
            n747 = event-data() -> ()  [unwired: 1 in, 6 out]
            n748 = local write "Define 1"(FALSE) -> ()
            n749 = local read "TI-Ctrl"() -> (w1027:T9)
            n750 = Unbundle By Name(w1027) -> ("Z-Ctrl.Z-pos"=w1025:dbl)
            n751 = local read "Z-Stack"() -> (w1023:T10)
            n752 = Bundle By Name(cluster=w1023, "Z0"=w1025) -> (w1024:T10)
            n753 = local write "Z-Stack"(w1024) -> ()
          }
          event "Define 2": Value Change {
            n754 = event-data() -> ()  [unwired: 1 in, 6 out]
            n755 = local read "TI-Ctrl"() -> (w1032:T9)
            n756 = Unbundle By Name(w1032) -> ("Z-Ctrl.Z-pos"=w1030:dbl)
            n757 = local write "Define 2"(FALSE) -> ()
            n758 = local read "Z-Stack"() -> (w1029:T10)
            n759 = Bundle By Name(cluster=w1029, "Z end"=w1030) -> (w1028:T10)
            n760 = local write "Z-Stack"(w1028) -> ()
          }
        }
        n761 = local read "stop program"() -> (w929:bool)
      }
      n762 = property on="Confocal VISA Setting" class="VISAName"() -> ("Value"=w32:refnum<visa-resource-name>)  [unwired: 2 in, 2 out]
      n763 = while {
        shift-right: [w728] -> _
        shift-left: errorcluster {"status"=FALSE, "code"=0, "source"=""} ("Confocal") -> [w732]
        tunnel: w32 -> [w731]
        stop <- w729 stop-if-true
        # "Confocal scanner"
        n764 = event shown="[0] Timeout" {
          selector: _ -> [_ _ _ _ _ _ _]
          dyn-events: _ -> [_ _ _ _ _ _ _]
          timeout: 50 -> [_ _ _ _ _ _ _]
          tunnel: w732 -> [w735 w748 w765 w768 w772 w776 w780]
          tunnel: [w733 w744 w764 w767 w771 w775 w779] -> w728
          tunnel: w731 -> [w736 w749 w762 w769 w773 w777 w781]
          event Timeout {
            n765 = event-data() -> ()  [unwired: 1 in, 1 out]
            n766 = local read "SDC initialized"() -> (w734:bool)
            n767 = case shown="True" w734 {
              tunnel: w736 -> [_ w739]
              tunnel: w735 -> [w737 w741]
              tunnel: [w737 w740] -> w733
              frame False {
              }
              frame True {
                n768 = call "SubConfocal_GetInfo.vi"("Error In"=w741, "Confocal line (VISA IN)"=w739) -> ("Error out"=w740:errorcluster, "Confocal Info"=→"Confocal Info":T20)  [unwired: 8 in]
              }
            }
          }
          event "Confocal on?": Value Change {
            n769 = event-data() -> ("NewVal"=w747:bool)  [unwired: 1 in]
            n770 = case shown="False" w747 {
              tunnel: w749 -> [w753 w760]
              tunnel: w748 -> [w752 w759]
              tunnel: [w750 w758] -> w743
              tunnel: [T23."Disabled and Grayed Out" ("Disabled") T23."Enabled" ("Disabled")] -> w746
              tunnel: [T24 {"SDC shutter"=FALSE, "FWPosition"=3, "FW speed"=3, "Disk spinning?"=FALSE, "Disk speed (rpm)"=3000.0} ("Confocal scanner") w756] -> w745
              tunnel: [FALSE ("SDC initialized") TRUE ("SDC initialized")] -> w742
              frame False {
                n771 = call "SubConfocal_StartStop.vi"("Error In"=w752, "Confocal line (VISA IN)"=w753) -> ("Error out"=w750:errorcluster)  [unwired: 9 in]
              }
              frame True {
                n772 = local read "Confocal scanner"() -> (w756:T5)
                n773 = call "SubConfocal_StartStop.vi"("Confocal scanner"=w756, "Error In"=w759, "Confocal line (VISA IN)"=w760) -> ("Error out"=w758:errorcluster)  [unwired: 8 in]
              }
            }
            n774 = property on="Confocal scanner" class="Clust (strict)"("DisabledEnum"=w746) -> ()  [unwired: 2 in, 2 out]
            n775 = property on="Confocal scanner" class="Clust (strict)"("Value"=w745) -> ()  [unwired: 2 in, 2 out]
            n776 = property on="SDC initialized" class="Bool (strict)"(error in=w743, "Value"=w742) -> (error out=w744:errorcluster)  [unwired: 1 in, 1 out]
          }
          event "Confocal scanner.SDC shutter": Value Change {
            n777 = event-data() -> ()  [unwired: 1 in, 1 out]
            n778 = local read "Confocal scanner"() -> (w763:T5)
            n779 = call "SubConfocal_SetShutterStatus.vi"("Confocal scanner"=w763, "Error In"=w765, "Confocal line (VISA IN)"=w762) -> ("Error out"=w764:errorcluster)  [unwired: 7 in, 1 out]
          }
          event "Confocal scanner.Filter wheel": Value Change {
            n780 = event-data() -> ()  [unwired: 1 in, 1 out]
            n781 = local read "Confocal scanner"() -> (w766:T5)
            n782 = call "SubConfocal_SetFWpos.vi"("Confocal scanner"=w766, "Error In"=w768, "Confocal line (VISA IN)"=w769) -> ("Error out"=w767:errorcluster)  [unwired: 7 in, 1 out]
          }
          event "Confocal scanner.FW speed": Value Change {
            n783 = event-data() -> ()  [unwired: 1 in, 1 out]
            n784 = local read "Confocal scanner"() -> (w770:T5)
            n785 = call "SubConfocal_SetFWSpeed.vi"("Confocal scanner"=w770, "Error In"=w772, "Confocal line  (VISA IN)"=w773) -> ("Error out"=w771:errorcluster)  [unwired: 7 in, 1 out]
          }
          event "Confocal scanner.Disk spinning": Value Change {
            n786 = event-data() -> ()  [unwired: 1 in, 1 out]
            n787 = local read "Confocal scanner"() -> (w774:T5)
            n788 = call "SubConfocal_DiskSpinningOnOff.vi"("Confocal scanner"=w774, "Error In"=w776, "Confocal line (VISA IN)"=w777) -> ("Error out"=w775:errorcluster)  [unwired: 7 in, 1 out]
          }
          event "Confocal scanner.Disk speed (rpm)": Value Change {
            n789 = event-data() -> ()  [unwired: 1 in, 1 out]
            n790 = local read "Confocal scanner"() -> (w778:T5)
            n791 = call "SubConfocal_SetDiskSpinningSpeed.vi"("Confocal scanner"=w778, "Error In"=w780, "Confocal line (VISA IN)"=w781) -> ("Error out"=w779:errorcluster)  [unwired: 7 in, 1 out]
          }
        }
        "Confocal" <- w728
        n792 = local read "stop program"() -> (w729:bool)
      }
    }
    frame #2 {
      # "Close camera, stage, and deinitialize"
      n793 = flat-sequence {
        frame #0 {
          n794 = local read "Camera on?"() -> (w1070:bool)
          n795 = local read "Confocal on?"() -> (w1072:bool)
          n796 = local read "Stage on?"() -> (w1071:bool)
          n797 = case shown="True" w1070 {
            tunnel: errorcluster {"status"=FALSE, "code"=0, "source"=""} ("error in (no error)") -> [w1074 w1078]
            tunnel: [w1074 w1077] -> w1069
            frame False {
            }
            frame True {
              n798 = property on="Handle" class="DigNum (strict)"() -> ("Value"=w1075:u32)  [unwired: 2 in, 2 out]
              n799 = property on="Live" class="Bool (strict)"() -> ("Value"=w1076:bool)  [unwired: 2 in, 2 out]
              n800 = call "subHamamatsu_TurnOnOff.vi"("logic 2"=FALSE, "logic 1"=w1076, "error in (no error)"=w1078, "Handle in"=w1075) -> ("error out"=w1080:errorcluster, "Handle out"=w1079:u32)  [unwired: 5 in, 1 out]
              n801 = call "subHamamatsu_Deinitialization.vi"("error in (no error)"=w1080, "Handle"=w1079) -> ("error out"=w1077:errorcluster)  [unwired: 9 in]
            }
          }
          n802 = case shown="True" w1071 {
            frame False {
            }
            frame True {
              n803 = local read "Stage Status"() -> (w1083:T7)
              n804 = call "Disconnect.vi"("Stage Info"=w1083) -> ()  [unwired: 10 in, 1 out]
              n805 = property on="Stage Status" class="Clust (strict)"("Value"=T7 {" Current Position"=[-1.0, -12.0, 0.0], "Number of Axis"=3, "ILSID"=1} ("Stage Info")) -> ()  [unwired: 2 in, 2 out]
            }
          }
          n806 = case shown="True" w1072 {
            frame False {
            }
            frame True {
              n807 = property on="Confocal VISA Setting" class="VISAName"() -> ("Value"=w1084:refnum<visa-resource-name>)  [unwired: 2 in, 2 out]
              n808 = call "SubConfocal_StartStop.vi"("Confocal line (VISA IN)"=w1084) -> ()  [unwired: 10 in, 1 out]
              n809 = property on="Confocal scanner" class="Clust (strict)"("Value"=T5 {"SDC shutter"=FALSE, "Filter wheel"=3, "FW speed"=3, "Disk spinning"=FALSE, "Disk speed (rpm)"=3000.0} ("Confocal scanner")) -> ()  [unwired: 2 in, 2 out]
            }
          }
          n810 = property on="DAQ ports" class="Clust (strict)"() -> ("Value"=w1065:T25)  [unwired: 2 in, 2 out]
          n811 = call "subDAQ_SetLaserDO.vi"("DAQ ports"=w1065) -> ("Error out"=w1066:errorcluster)  [unwired: 10 in]
          n812 = local write "Camera"(w1069) -> ()
          n813 = call "subDAQ_SetLED.vi"("DAQ ports"=w1065, "Error in (no error)"=w1066) -> ()  [unwired: 9 in, 1 out]
          n814 = local read "Scope on?"() -> (w1067:bool)
          n815 = case shown="True" w1067 {
            frame False {
            }
            frame True {
              n816 = local read "TiE Ref"() -> (w1073:T21)
              n817 = call "subTiE_Deinitialize.vi"("Ref"=w1073) -> ()  [unwired: 11 in]
            }
          }
        }
        frame #1 {
          w1086 = FALSE ("stop program")
          w1090 = "\t"
          n818 = local read "log path"() -> (w1087:path)
          n819 = local write "Camera initialized"(bool[] [FALSE, FALSE] ("Camera initialized")) -> ()
          n820 = local write "Stage on?"(w1086) -> ()
          n821 = local write "Scope on?"(w1086) -> ()
          n822 = local write "Confocal on?"(w1086) -> ()
          n823 = local write "Camera on?"(w1086) -> ()
          n824 = local write "Stage initialized"(w1086) -> ()
          n825 = local write "Ti-E initialized"(w1086) -> ()
          n826 = local write "SDC initialized"(w1086) -> ()
          n827 = local write "stop program"(w1086) -> ()
          n828 = Format Date/Time String(time format string (%c)="%X") -> (date/time string=w1089:string)  [unwired: 2 in]
          n829 = Read from Text File(file (use dialog)=w1087) -> (refnum out=w1094:refnum<file>, text=w1092:string)  [unwired: 3 in, 2 out]
          n830 = Concatenate Strings(w1092, "\r", w1090, w1090, w1090, w1090, w1089) -> (w1093:string)
          n831 = Close File(refnum=w1094) -> (path=w1095:path)  [unwired: 1 in, 1 out]
          n832 = property on="Live" class="Bool (strict)"("Value"=w1086) -> ()  [unwired: 2 in, 2 out]
          n833 = Write to Text File(file (use dialog)=w1095, text=w1093) -> ()  [unwired: 2 in, 3 out]
        }
      }
    }
  }
